vi "MC_7_26_12c_JW.vi"() -> ()   [LabVIEW 2011]
uses:
  <vilib>/Utility/file.llb/Read From Spreadsheet File (string).vi
  <vilib>/Utility/inputDevices.llb/keyboardAcquire.vi
  <vilib>/Utility/file.llb/Write To Spreadsheet File (DBL).vi
  <vilib>/Utility/file.llb/Write To Spreadsheet File (string).vi
  <vilib>/regexp/Match Regular Expression.xnode
panel:
  in  "Room Temp":dbl=294.0
  out "No Image 2":path=path "\\\\acad1\\physics/Jurchescu-group/JW-PD/Image Not Found.png"
  out "Save1 Array":string[][](array[string])
  out "XY Graph-Lin":cluster{dbl[], dbl[]}[](graph)
  out "Lin Vd":dbl
  out "Lin-Vg Array-Used":dbl[](array[numeric])
  out "Lin Id-Used":dbl[](array[numeric])
  out "Comments":string
  out "Folder Index":dbl caption="Length"
  out "Current \nRecord":string[](array[string])
  out "Transformer \nHeaders":string[](array[string])
  out "Current Device ID":string
  out "Column":string
  out "Row":string
  out "Rec: Concentration":dbl
  out "Rec: Solvent":string
  out "Rec: Method":string
  in  "?":T1(tab)
  out "Rec: Material":string
  in  "Treatment Concentration (mM):":dbl=30.0
  in  "Surface Treatment:":string
  in  "# Drops*:":dbl=inf
  in  "Solution Temp (C):":dbl=55.0
  in  "Relative Humidity (%):":dbl=nan
  in  "Room Temp (F):":dbl=nan
  in  "Time (s):":dbl=80.0
  out "Accel (RPM/s):":dbl
  in  "RPM:":dbl=1000.0
  in  "Wait Time (s):":dbl=10.0
  in  "Sample #:":dbl=1.0
  in  "Fabricator:":string="Jeremy"
  in  "Data File":path
  out "Data Folder":path
  in  "Image Folder":path
  out "Image File":path=path "D:/UserData/Desktop/Jeremy/WFU/Research/Programs/VI mods/Image Not Found.png"
  in  "Ramp (s):":dbl=3.0
  out "Calc: On/Off":dbl caption="On/Off-Sat" format="%#.2e"
  out "Calc: Off I-Sat":dbl caption="Off I-Sat" format="%#.2e"
  in  "Manuel-Dielectric":bool
  in  "Manuel-Length":bool
  out "Calc: VT-Lin":dbl
  out "New: VT-Lin":dbl
  out "Rec: VT-Lin":dbl caption="VT-Lin" format="%#_3g"
  out "Calc: Trap Density-STS":dbl format="%#.2e"
  out "New: Trap Density-STS":dbl format="%#.2e"
  out "Rec: Trap Density-STS":dbl caption="N-Sat (STS)" format="%#.2e"
  out "Calc: Trap Density-VT":dbl format="%#.2e"
  out "New: Trap Density-VT":dbl format="%#.2e"
  out "Rec: Trap Density-VT":dbl caption="N-Sat (VT)" format="%#.2e"
  out "Calc: Mobility-Lin":dbl format="%#.2e"
  out "New: Mobility-Lin":dbl format="%#_4e"
  out "Rec: Mobility-Lin":dbl caption="Mobility-Lin" format="%#_3e"
  out "Calc: Mobility-Sat":dbl format="%#.2e"
  out "Rec: Length":dbl caption="Length" format="%#_3g"
  out "Rec: Width":dbl caption="Width" format="%#_4g"
  out "Rec: Dielectric (d)":dbl caption="Dielectric (d)" format="%#_3g"
  out "XY Graph":cluster{dbl[], dbl[]}[](graph)
  in  "NumPts":dbl=5.0
  in  "Cancel Button":bool
  in  "Next Button":bool
  in  "Previous Button":bool
  in  "Up Button":bool
  in  "Down Button":bool
  out "Data Name:":string
  in  "Save Changes?":bool
  in  "New: Dielectric":dbl
  in  "New: Length":dbl
  in  "New: Width":dbl
  out "New: Mobility-Sat":dbl format="%#.2e"
  in  "Slide":dbl(slide) step=1.0 scale=-22.0..202.0 scale format="%#_1p"
  in  "Blank Button":bool
  in  "Zoom":i16(slide)=-3 scale=-5.0..5.0
  out "Image Out 2":T2(plugin-control)
  out "Image Out":T2(plugin-control)
  in  "Magnification":u16(ring) items=["5x", "10x", "20x", "50x", "80x"]
  out "Total Width":dbl
  out "Distances":dbl[](array[numeric])
  in  "Undo Button":bool
  in  "Remove Button":bool
  out "Rec: Mobility-Sat":dbl caption="Mobility-Sat" format="%#.2e"
  out "Index":string
  out "Image Name":string
  in  "Export":bool
  out "Calc: VT-Sat":dbl format="%#.2g"
  out "New: VT-Sat":dbl format="%#.2g"
  in  "Manual-Width":bool caption="Manual"
  out "XY Graph 2":cluster{dbl[], dbl[]}[](graph)
  in  "Next Button 2":bool
  in  "Previous Button 2":bool
  in  "Slide 2":dbl(slide) step=1.0 scale=-1.0..82.0 scale format="%#_1p"
  out "Calc: STS":dbl format="%#.2g"
  out "New: STS":dbl format="%#.2g"
  in  "NumPts 2":dbl=5.0 caption="NumPts"
  out "Rec: VT-Sat":dbl caption="VT-Sat" format="%#.2g"
  out "Rec: STS":dbl caption="STS-Sat" format="%#.2g"
  out "Rec: On/Off":dbl caption="On/Off-Sat" format="%#.2e"
  in  "Save Changes? 2":bool
  in  "Save Changes? 3":bool
  out "Date Recorded":string="Date Recorded" caption="Measured"
  out "Date Created":string caption="Fabricated"
  out "Rec: Temp":dbl caption="Sample Temp" format="%.1f"
  out "New: Temp":dbl format="%.1f"
  out "Rec: Off I-Sat":dbl caption="Off I-Sat" format="%#.2e"
  in  "Independant Variable":string(combo)="Length (um):"
  out "String":string
  in  "No Image":path=path "\\\\acad1\\physics/Jurchescu-group/JW-PD/Image Not Found.png"
  in  "Project":path=path "\\\\acad1\\physics/Jurchescu-group/JW-PD/Group Library/Origin Project Files/DeviceData_7_25a_JWW.opj"
  out "Index 2":dbl
  out "Sat Id-Log-Used":dbl[](array[numeric])
  out "Vg Array-Log-Used":dbl[](array[numeric])
  out "ROI Descriptor out":T3 {"Contours"."Type" items=["No Selection", "Point", "Line", "Rectangle", "Oval", "Polygon", "Freehand Region", "Annulus", "Unused2", "Unused3", "Broken Line", "Freehand Line", "Rotated Rectangle"]}
  out "ROI Descriptor":T3 {"Contours"."Type" items=["No Selection", "Point", "Line", "Rectangle", "Oval", "Polygon", "Freehand Region", "Annulus", "Unused2", "Unused3", "Broken Line", "Freehand Line", "Rotated Rectangle"]}
  out "Numeric 3":dbl
  out "Array 6":dbl[][](array[numeric])
  out "Cluster":T4
  out "Array 5":dbl[](array[numeric])
  out "Array 4":dbl[](array[numeric])
  out "Array 3":dbl[](array[numeric])
  out "Numeric 2":dbl
  out "Numeric":dbl
  out "Sat Id-Used":dbl[](array[numeric])
  out "Sat Vg Array-Used":dbl[](array[numeric])
  out "MobVi Index":dbl
  in  "Row Start":dbl=20.0
  # "Data Locations"
  # "Data Location"
  # "Image Location"
  # "Sample Properties"
  # "*     Inf = Full coverage\n   NaN = Unknown or Not Applicable"
  # "Recorded"
  # "Calculated"
  # "Re-Calculated"
  # "Manual"
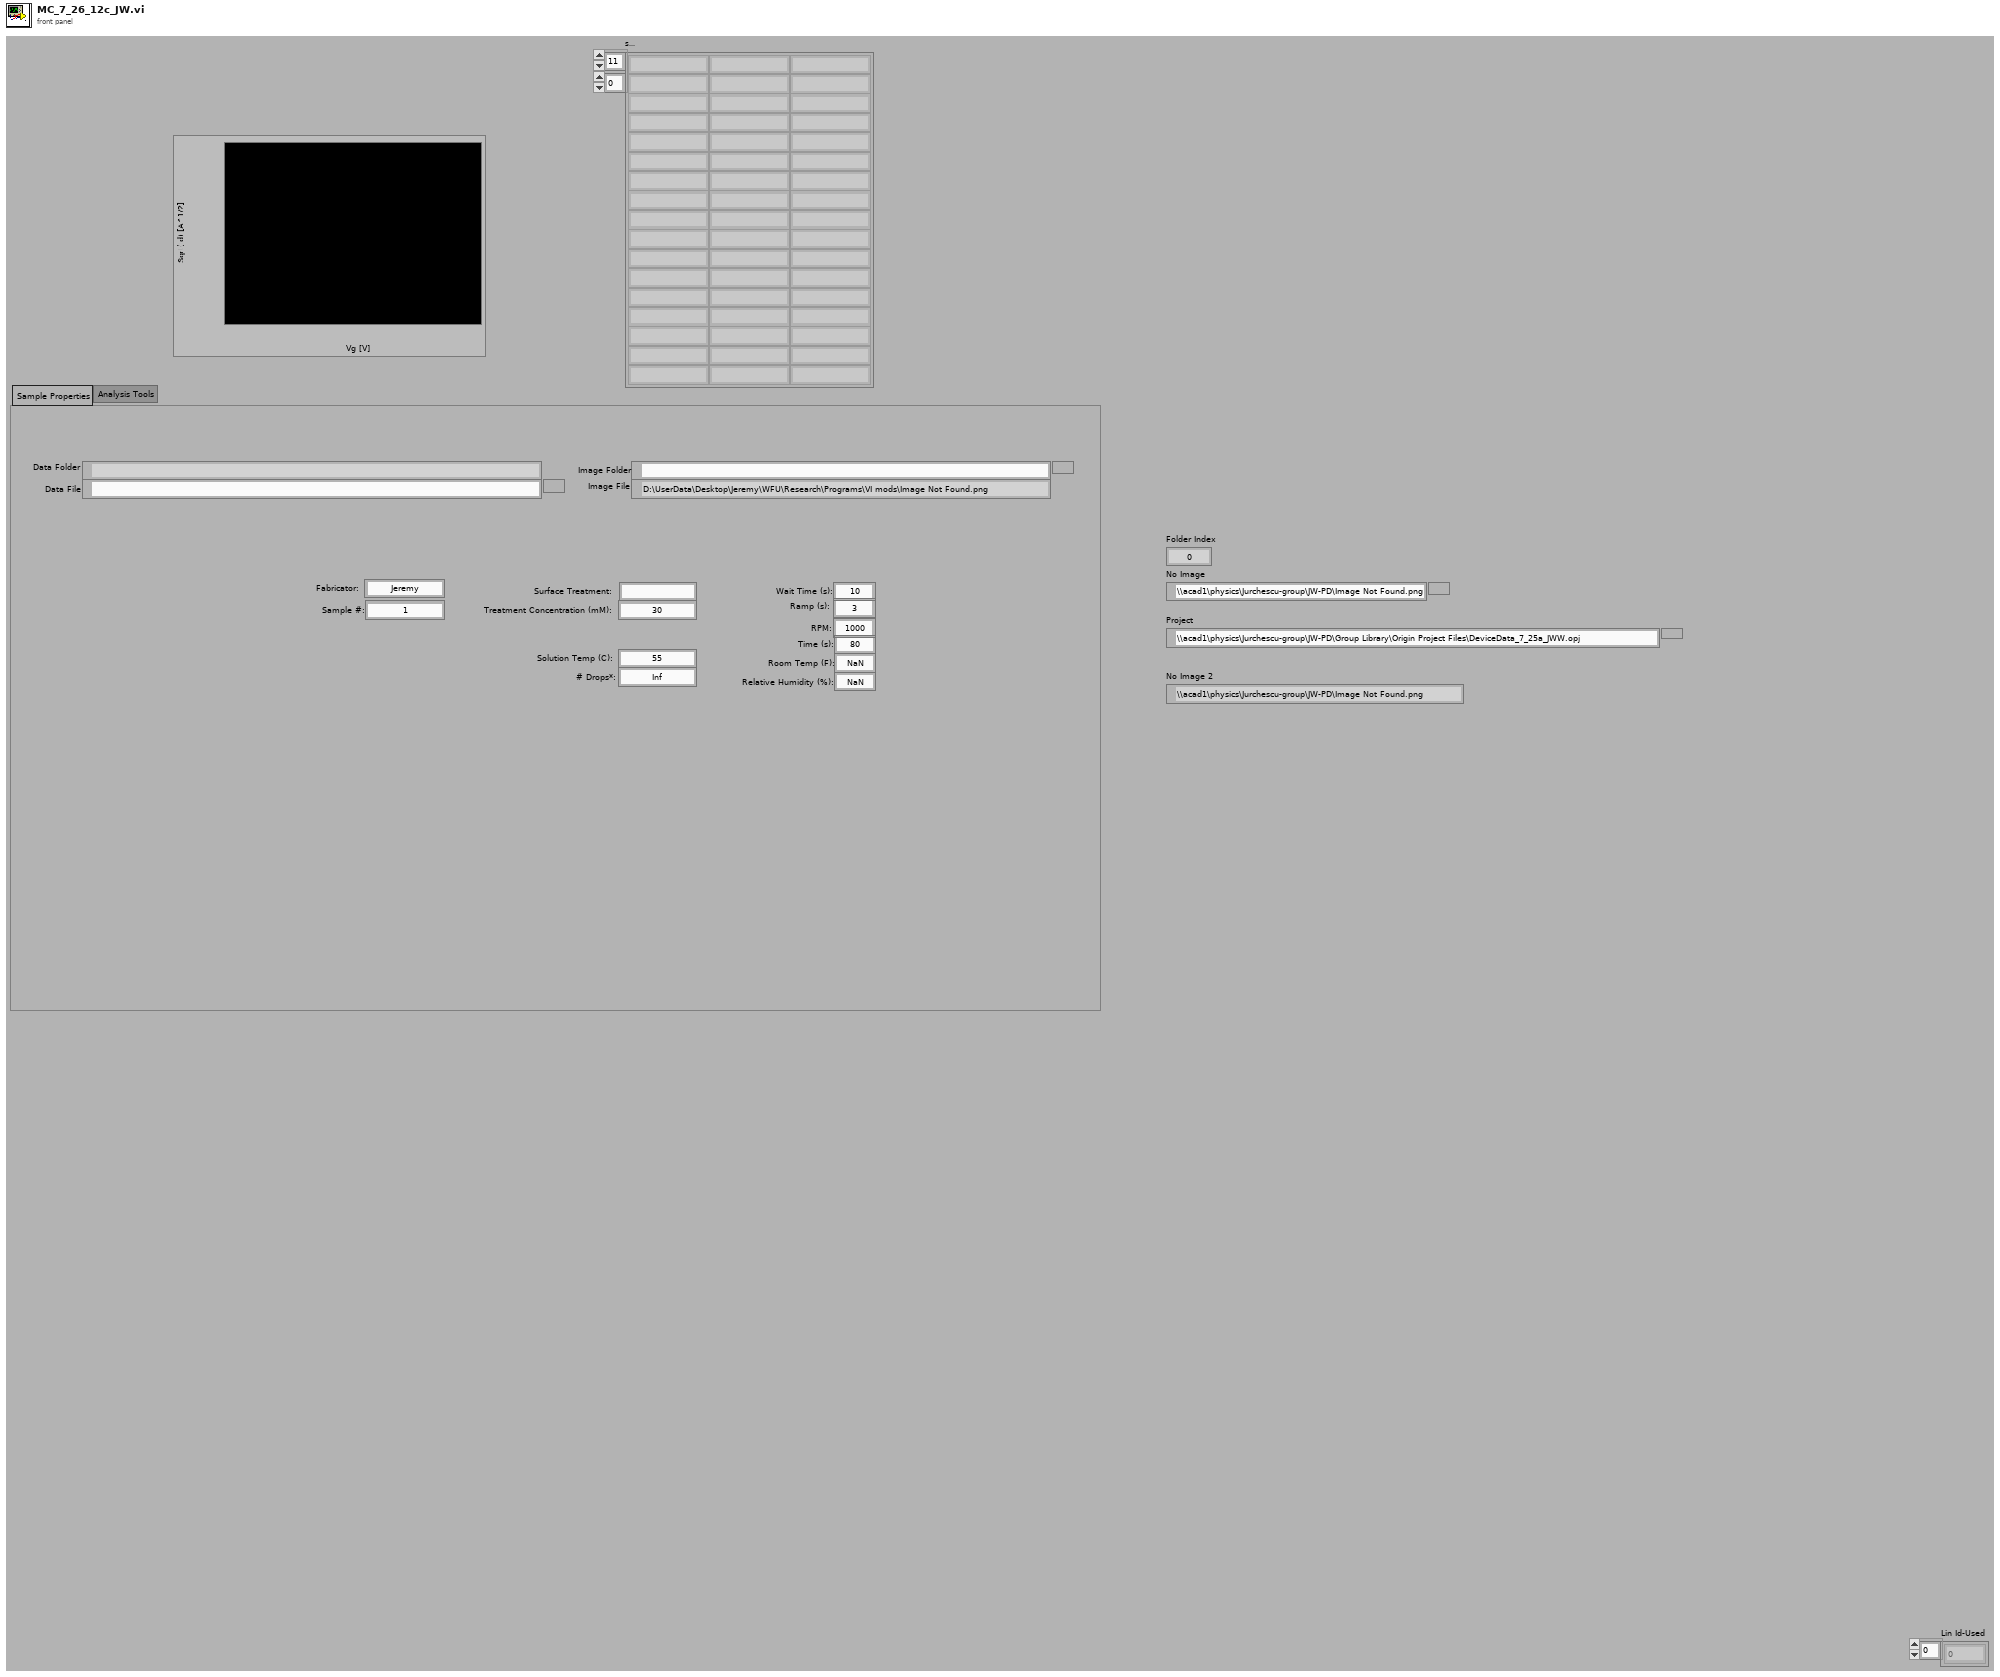
[diagram p1: front panel]
types:
  T1 = enum32{"Sample Properties", "Analysis Tools", "Current Database"}
  T2 = typedef "IMAQ Image.ctl" = refnum<image>
  T3 = typedef "ROI Descriptor" = cluster{"Global Rectangle":i32[], "Contours":cluster{"ID":enum32{"External", "Internal"}, "Type":u32, "Coordinates":i32[]}[]}
  T4 = cluster{"Numeric":dbl, "Numeric 2":dbl, "Numeric 3":dbl, "Numeric 4":dbl}
  T5 = cluster{"Mobility-Sat":dbl, "Moblitity-Lin":dbl, "On/Off":dbl, "Off Current":dbl, "Vt-Sat":dbl, "STS":dbl, "Trap Density-VT":dbl, "Trap Density-STS":dbl}
  T6 = cluster{"Date Recorded":string, "Index":string, "Length":dbl, "Width":dbl, "Sample Temp":dbl}
  T7 = cluster{"Date Created":string, "Material":string, "Solvent":string, "Concentration":dbl, "Method":string, "Dielectric (nm)":dbl, "Treatment":string, "Comments":string}
  T8 = cluster{"Mobility-Sat":dbl, "Vt-Sat":dbl, "Mobility-Lin":dbl, "Vt-Lin":dbl, "Off I-Sat":dbl, "On/Off I-Sat":dbl}
  T9 = cluster{"[0]":cluster{dbl[], dbl[]}, "[1]":cluster{dbl[], dbl[]}, "[2]":cluster{dbl[], dbl[]}, "[3]":cluster{dbl[], dbl[]}, "[4]":cluster{dbl[], dbl[]}, "[5]":cluster{dbl[], dbl[]}, "[6]":cluster{dbl[], dbl[]}, "[7]":cluster{dbl[], dbl[]}, "[8]":cluster{dbl[], dbl[]}}
  T10 = cluster{"Global Rectangle":i32[], "Contours":cluster{"Contour Type":u32, "ROI Type":u32, "Points":i32[]}[]}
  T11 = typedef "LVBoundsTypeDef.ctl" = cluster{"Width":u32, "Height":u32}
  T12 = enum16{"0", "1", "2", "3", "4", "5", "6", "7", "8", "9", "A", "B", "C", "D", "E", "F", "G", "H", "I", "J", "K", "L", "M", "N", "O", "P", "Q", "R", "S", "T", "U", "V", "W", "X", "Y", "Z", "F1", "F2", "F3", "F4", "F5", "F6", "F7", "F8", "F9", "F10", "F11", "F12", "F13", "F14", "F15", "ADD", "BACK", "BACKSLASH", "CAPITAL", "COMMA", "DECIMAL", "DELETE", "DIVIDE", "DOWN", "END", "EQUALS", "ESCAPE", "GRAVE (`)", "HOME", "INSERT", "LBRACKET", "LCONTROL", "LEFT", "L ALT", "LSHIFT", "LWIN", "MINUS", "MULTIPLY", "NEXT", "NUMLOCK", "NUMPAD_0", "NUMPAD_1", "NUMPAD_2", "NUMPAD_3", "NUMPAD_4", "NUMPAD_5", "NUMPAD_6", "NUMPAD_7", "NUMPAD_8", "NUMPAD_9", "PAUSE", "PERIOD", "PRIOR (PG UP)", "RBRACKET", "RCONTROL", "RETURN", "RIGHT", "R ALT", "RSHIFT", "RWIN", "SCROLL", "SEMICOLON", "SLASH", "SPACE", "SUBTRACT", "TAB", "UP", "ENTER (num pad)", "' (quote)"}[]
  T13 = enum16{"0", "1", "2", "3", "4", "5", "6", "7", "8", "9", "A", "B", "C", "D", "E", "F", "G", "H", "I", "J", "K", "L", "M", "N", "O", "P", "Q", "R", "S", "T", "U", "V", "W", "X", "Y", "Z", "F1", "F2", "F3", "F4", "F5", "F6", "F7", "F8", "F9", "F10", "F11", "F12", "F13", "F14", "F15", "ADD", "BACK", "BACKSLASH", "CAPITAL", "COMMA", "DECIMAL", "DELETE", "DIVIDE", "DOWN", "END", "EQUALS", "ESCAPE", "GRAVE (`)", "HOME", "INSERT", "LBRACKET", "LCONTROL", "LEFT", "L ALT", "LSHIFT", "LWIN", "MINUS", "MULTIPLY", "NEXT", "NUMLOCK", "NUMPAD_0", "NUMPAD_1", "NUMPAD_2", "NUMPAD_3", "NUMPAD_4", "NUMPAD_5", "NUMPAD_6", "NUMPAD_7", "NUMPAD_8", "NUMPAD_9", "PAUSE", "PERIOD", "PRIOR (PG UP)", "RBRACKET", "RCONTROL", "RETURN", "RIGHT", "R ALT", "RSHIFT", "RWIN", "SCROLL", "SEMICOLON", "SLASH", "SPACE", "SUBTRACT", "TAB", "UP", "ENTER (num pad)", "' (quote)"}
  T14 = cluster{"Contour Type":u32, "ROI Type":u32, "Points":i32[]}[]
  T15 = cluster{i32[], cluster{"Contour Type":u32, "ROI Type":u32, "Points":i32[]}[]}
  T16 = cluster{string, sgl, bool, bool, bool, bool, bool, bool, i32}
  T17 = cluster{i32, cluster{string, sgl, bool, bool, bool, bool, bool, bool, i32}, i32, i32}
  T18 = cluster{"Contour Type":u32, "ROI Type":u32, "Points":i32[]}
  T19 = cluster{"Points[0]":i32, "Points[1]":i32, "Points[2]":i32, "Points[3]":i32, "Points[4]":i32, "Points[5]":i32, "Points[6]":i32, "Points[7]":i32, "Points[8]":i32}
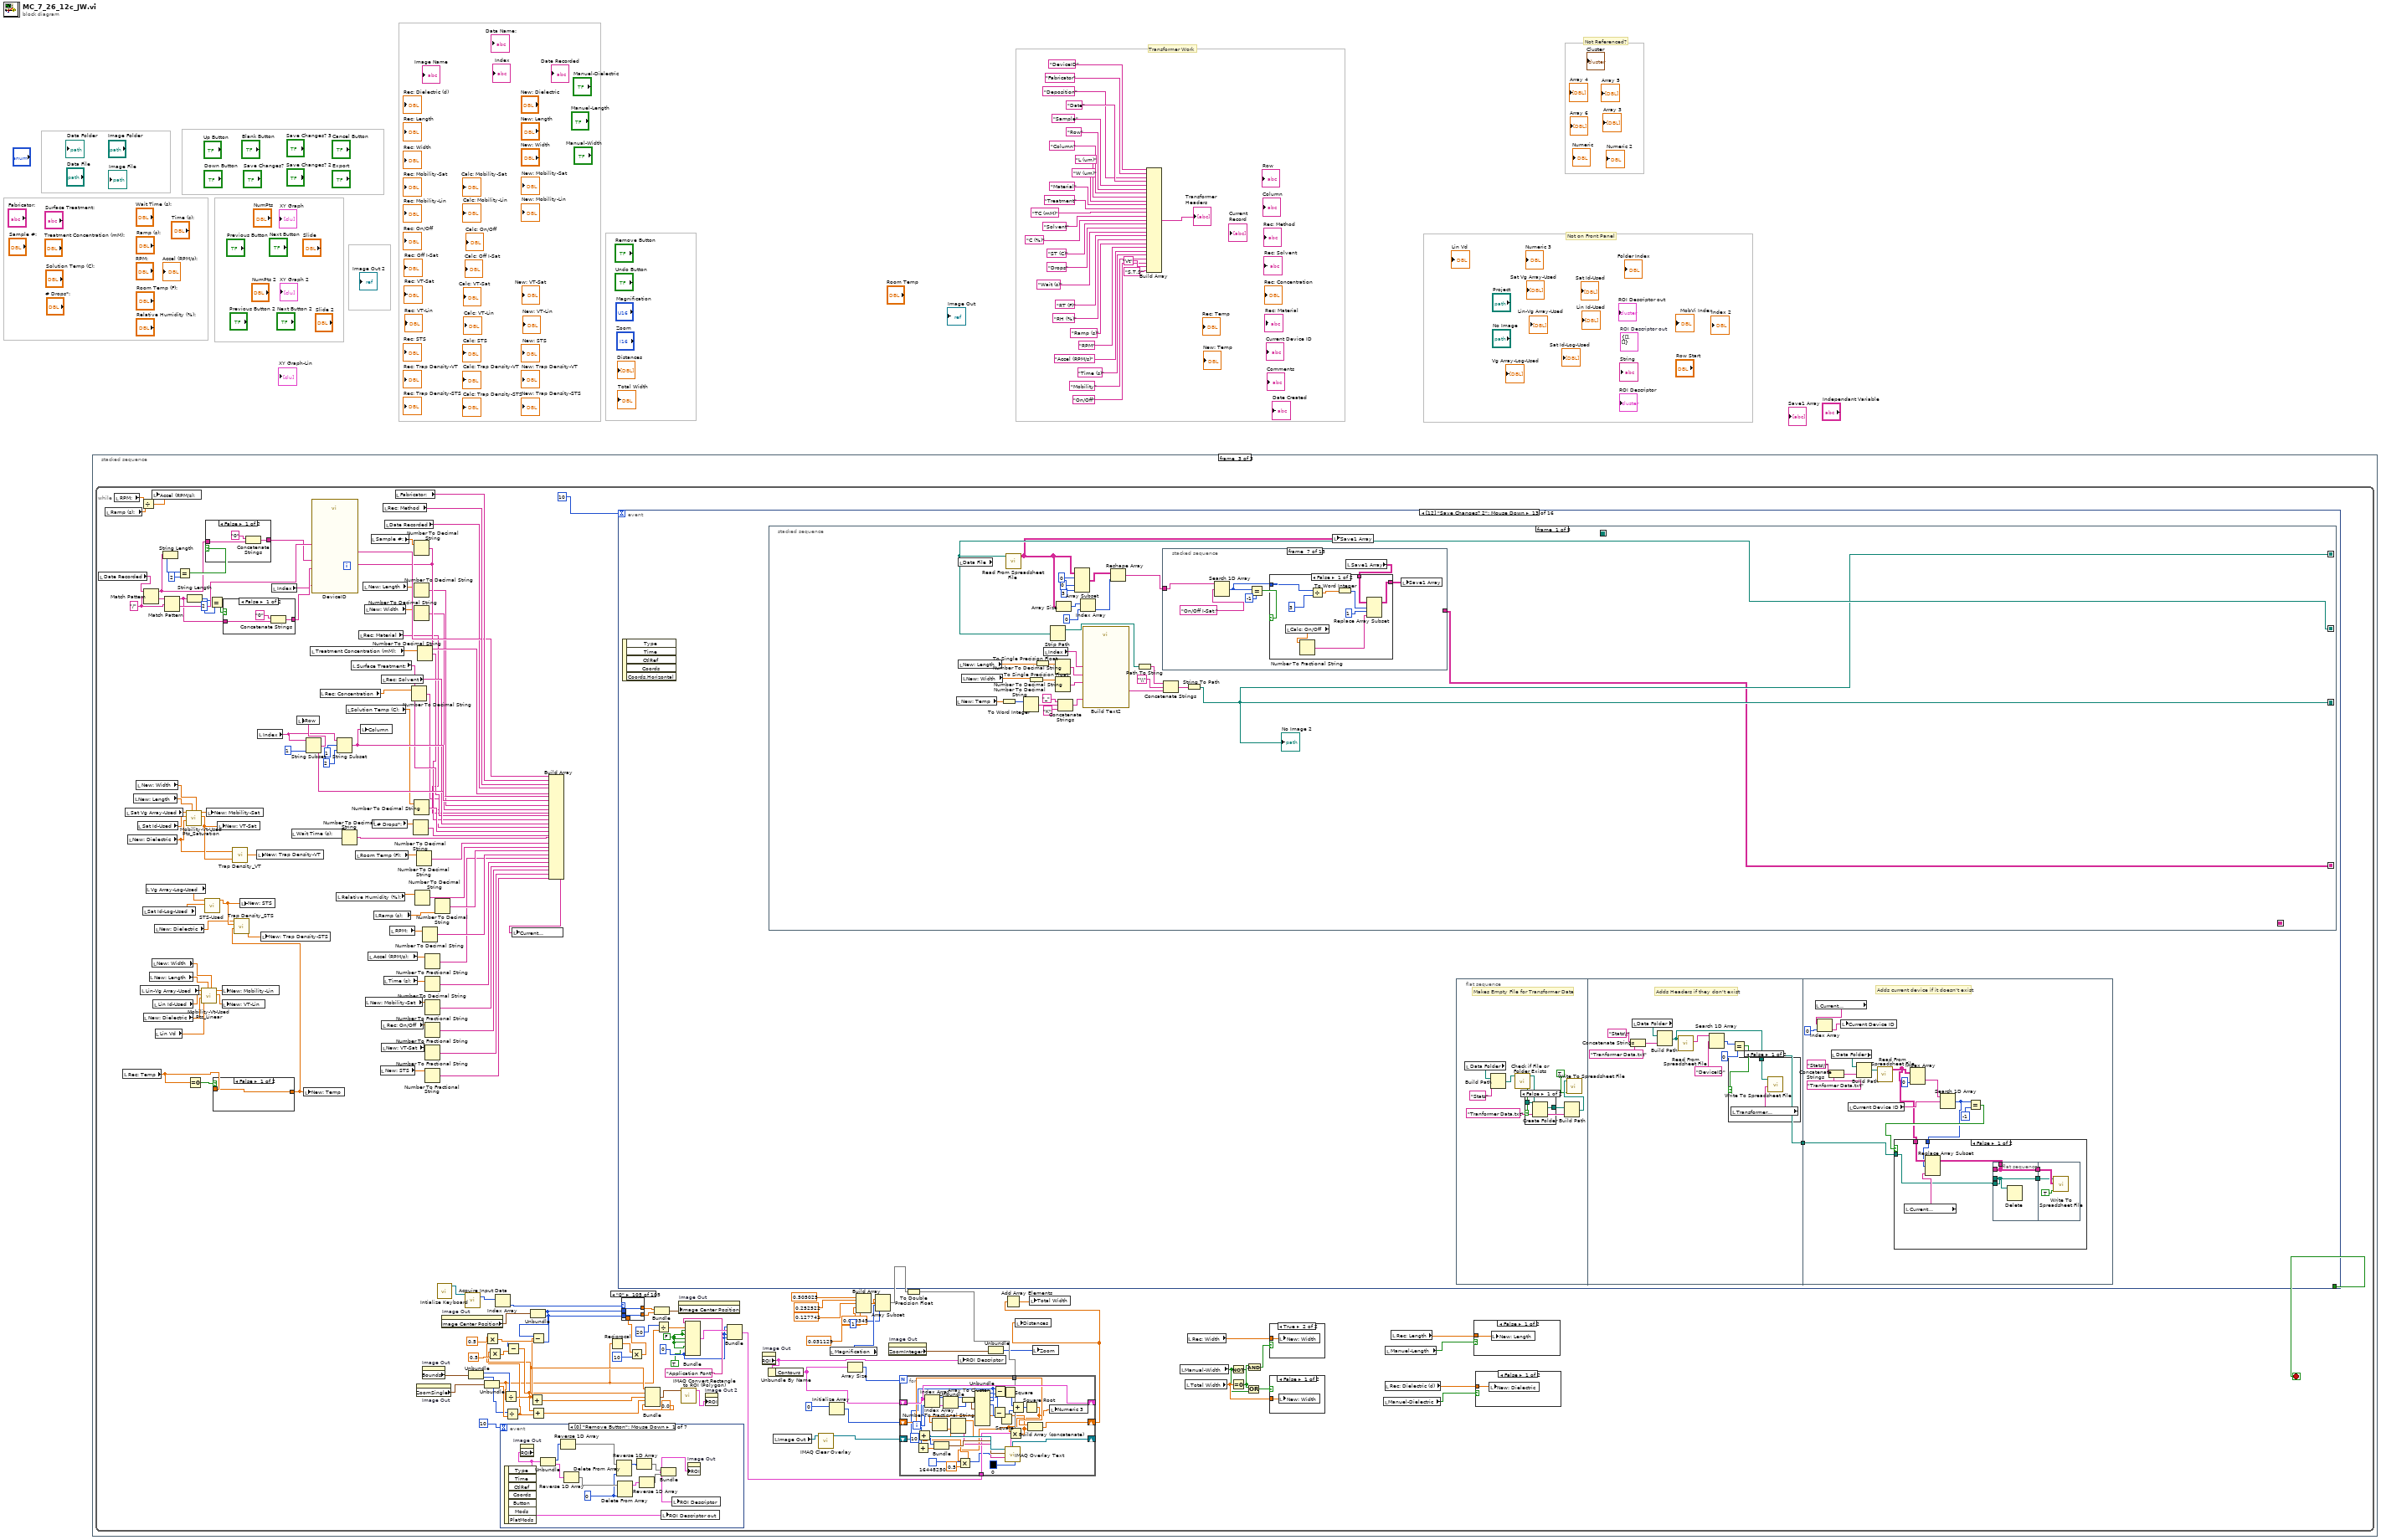
[diagram p0: block diagram]
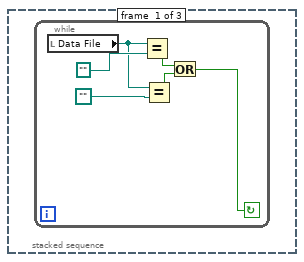
[diagram p2: hidden frame]
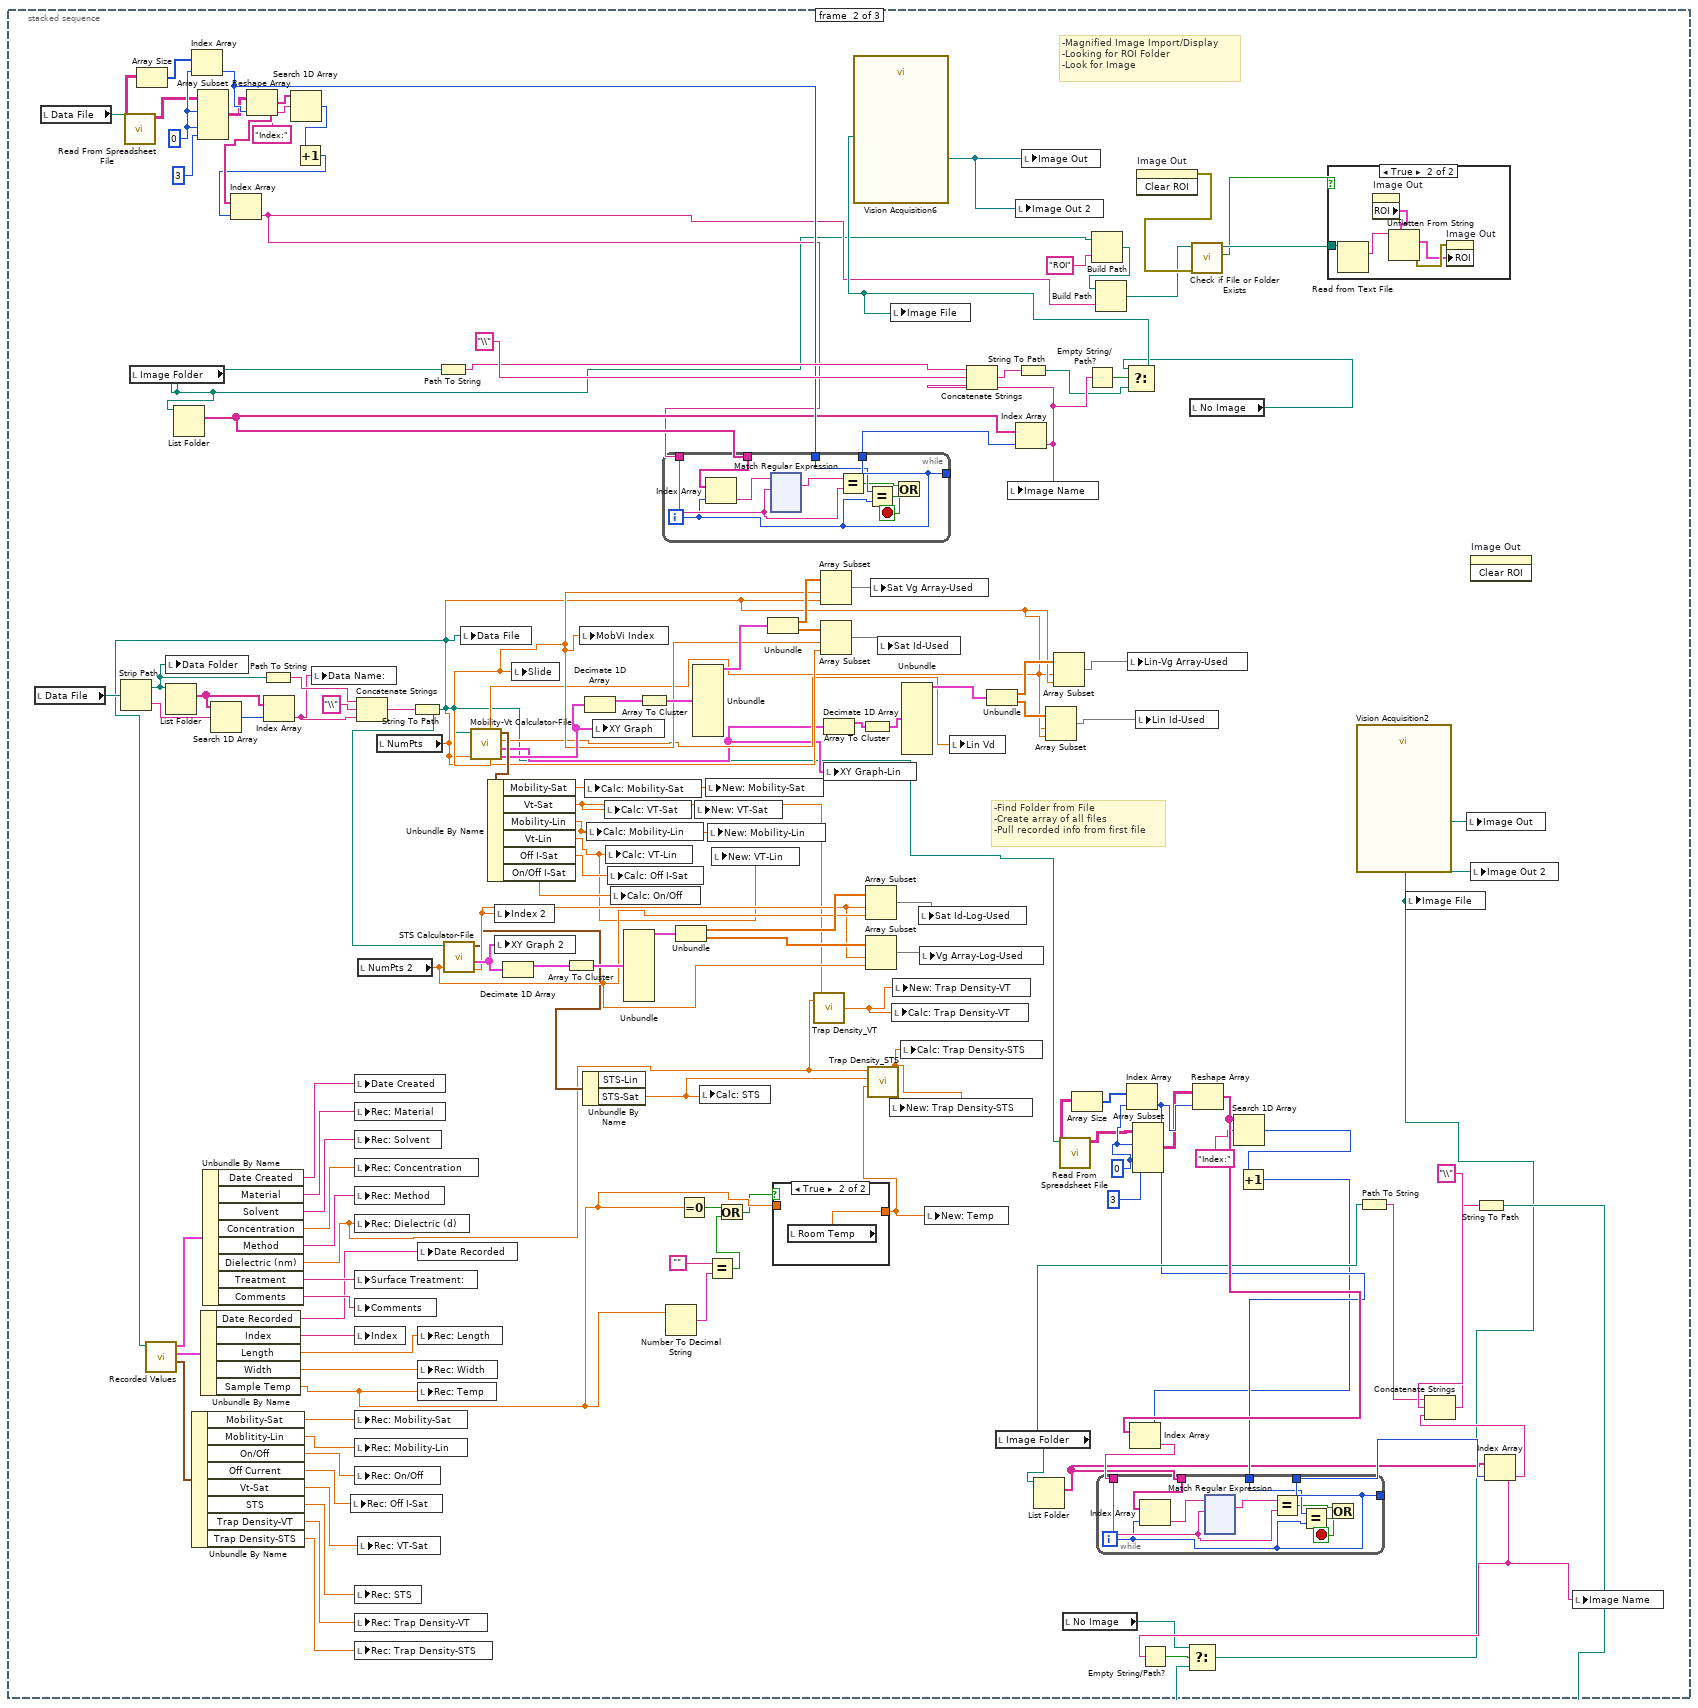
[diagram p3: hidden frame]
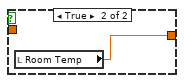
[diagram p6: hidden frame]
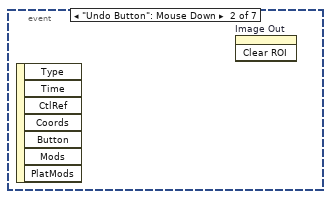
[diagram p13: hidden frame]
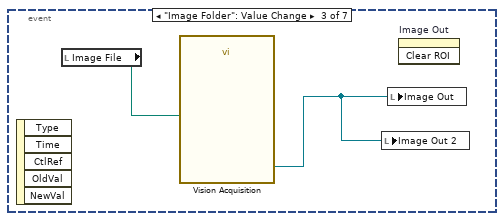
[diagram p14: hidden frame]
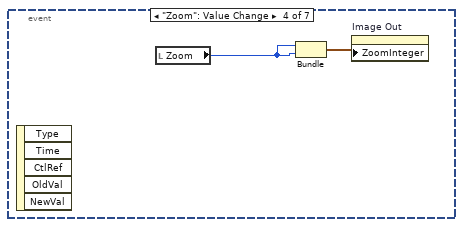
[diagram p15: hidden frame]
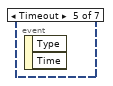
[diagram p16: hidden frame]
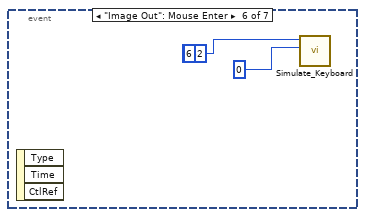
[diagram p17: hidden frame]
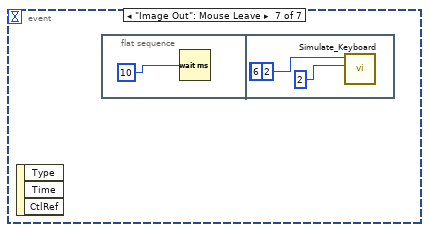
[diagram p18: hidden frame]
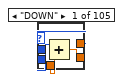
[diagram p19: hidden frame]
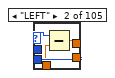
[diagram p20: hidden frame]
diagram:
  (unwired) T3 {"Global Rectangle"=[], "Contours"=[]}  # ROI Descriptor out
  # "Not Referenced?"
  # "Transformer Work"
  # "Not on Front Panel"
  n1 = stacked-sequence {
    frame #0 {
      n2 = while {
        stop <- w29 continue-if-true
        n3 = local read "Data File"() -> (w31:path)
        n4 = Equal?(x=w31, y=path "") -> (x = y?=w33:bool)
        n5 = Equal?(x=w31, y=path "") -> (x = y?=w32:bool)
        n6 = Or(x=w33, y=w32) -> (x .or. y?=w29:bool)
      }
    }
    frame #1 {
      w133 = 0
      w157 = 0
      # "-Find Folder from File\n-Create array of all files\n-Pull recorded info from first file"
      # "-Magnified Image Import/Display\n-Looking for ROI Folder\n-Look for Image"
      n7 = local read "Data File"() -> (w137:path)
      n8 = local read "Data File"() -> (w152:path)
      n9 = Strip Path(path=w137) -> (stripped path=w138:path, name=w124:string)
      n10 = call-poly <vilib>:"Read From Spreadsheet File.vi"("file path (dialog if empty)"=w152) -> ("all rows"=w155:string[][])  [unwired: 6 in, 4 out]
      n11 = local read "Image Folder"() -> (w94:path)
      n12 = Array Size(array=w155) -> (size(s)=w156:i32[])
      n13 = local write "Data Folder"(w138) -> ()
      n14 = List Folder(path=w138) -> (filenames=w128:string[])  [unwired: 3 in, 3 out]
      n15 = List Folder(path=w94) -> (filenames=w161:string[])  [unwired: 3 in, 3 out]
      n16 = Index Array(array=w156, index=w157) -> (element=w163:i32)
      n17 = Array Subset(array=w155, index (row)=w157, index (col)=w157, length (col)=3) -> (w154:string[][])  [unwired: 1 in]
      n18 = Search 1D Array(1D array=w128, element=w124) -> (index of element=w127:i32)  [unwired: 1 in]
      n19 = Reshape Array(w154, w163) -> (w168:string[])
      n20 = Path To String(path=w138) -> (string=w123:string)
      n21 = Index Array(array=w128, index=w127) -> (element=w93:string)
      n22 = Search 1D Array(1D array=w168, element="Index:") -> (index of element=w160:i32)  [unwired: 1 in]
      n23 = Increment(x=w160) -> (x+1=w159:i32)
      n24 = Index Array(array=w168, index=w159) -> (element=w95:string)
      n25 = local write "Data Name:"(w93) -> ()
      n26 = Concatenate Strings(w123, "\\", w93) -> (w125:string)
      n27 = local read "NumPts 2"() -> (w68:dbl)
      n28 = local read "NumPts"() -> (w59:dbl)
      n29 = String To Path(string=w125) -> (path=w52:path)
      n30 = call "Recorded Values.vi"("Path"=w52) -> ("Recorded Char"=w91:T5, "Recorded Prop"=w90:T6, "Fabrication Prop"=w92:T7)  [unwired: 8 in]
      n31 = Unbundle By Name(w91) -> ("Mobility-Sat"=w79:dbl, "Moblitity-Lin"=w78:dbl, "On/Off"=w77:dbl, "Off Current"=w76:dbl, "Vt-Sat"=w38:dbl, "STS"=w75:dbl, "Trap Density-VT"=w74:dbl, "Trap Density-STS"=w73:dbl)
      n32 = Unbundle By Name(w90) -> ("Date Recorded"=w83:string, "Index"=w82:string, "Length"=w81:dbl, "Width"=w80:dbl, "Sample Temp"=w44:dbl)
      n33 = Unbundle By Name(w92) -> ("Date Created"=w72:string, "Material"=w89:string, "Solvent"=w88:string, "Concentration"=w87:dbl, "Method"=w86:string, "Dielectric (nm)"=w48:dbl, "Treatment"=w85:string, "Comments"=w84:string)
      n34 = local write "Rec: Off I-Sat"(w76) -> ()
      n35 = local write "Date Created"(w72) -> ()
      n36 = local write "Rec: Material"(w89) -> ()
      n37 = local write "Rec: Solvent"(w88) -> ()
      n38 = local write "Rec: Concentration"(w87) -> ()
      n39 = local write "Rec: Method"(w86) -> ()
      n40 = local write "Rec: Dielectric (d)"(w48) -> ()
      n41 = local write "Surface Treatment:"(w85) -> ()
      n42 = local write "Comments"(w84) -> ()
      n43 = local write "Index"(w82) -> ()
      n44 = local write "Rec: Mobility-Sat"(w79) -> ()
      n45 = local write "Rec: Mobility-Lin"(w78) -> ()
      n46 = local write "Rec: On/Off"(w77) -> ()
      n47 = local write "Rec: STS"(w75) -> ()
      n48 = local write "Rec: Trap Density-VT"(w74) -> ()
      n49 = local write "Rec: Trap Density-STS"(w73) -> ()
      n50 = local write "Rec: VT-Sat"(w38) -> ()
      n51 = local write "Date Recorded"(w83) -> ()
      n52 = local write "Rec: Length"(w81) -> ()
      n53 = local write "Rec: Width"(w80) -> ()
      n54 = local write "Rec: Temp"(w44) -> ()
      n55 = Path To String(path=w94) -> (string=w165:string)
      n56 = call "STS Calculator-File.vi"("NumPts"=w68, "Path"=w52) -> ("STS Index-Sat"=w66:dbl, "XY Graph-Sat"=w67:cluster{dbl[], dbl[]}[], "Ouput"=w65:cluster{"STS-Sat":dbl, "STS-Lin":dbl})  [unwired: 5 in, 2 out]
      n57 = local write "Data File"(w52) -> ()
      n58 = call "Mobility-Vt Calculator-File.vi"("NumPts"=w59, "Path"=w52) -> ("XY Graph-Sat"=w70:cluster{dbl[], dbl[]}[], "XY Graph-Lin"=w54:cluster{dbl[], dbl[]}[], "Lin Vd"=w55:dbl, "Output"=w71:T8, "Index-Sat"=w69:dbl, "Index-Lin"=w58:dbl)  [unwired: 4 in]
      n59 = Unbundle By Name(w71) -> ("Mobility-Sat"=w47:dbl, "Vt-Sat"=w46:dbl, "Mobility-Lin"=w37:dbl, "Vt-Lin"=w35:dbl, "Off I-Sat"=w53:dbl, "On/Off I-Sat"=w36:dbl)
      n60 = local write "Index 2"(w66) -> ()
      n61 = local write "XY Graph 2"(w67) -> ()
      n62 = Decimate 1D Array(w67) -> (w115:cluster{dbl[], dbl[]}[])  [unwired: 1 out]
      n63 = local write "Slide"(w69) -> ()
      n64 = Array To Cluster(array=w115) -> (cluster=w117:T9)
      n65 = local write "MobVi Index"(w69) -> ()
      n66 = Unbundle By Name(w65) -> ("STS-Sat"=w51:dbl)  [unwired: 1 out]
      n67 = Decimate 1D Array(w70) -> (w151:cluster{dbl[], dbl[]}[])  [unwired: 1 out]
      n68 = local write "Calc: Mobility-Sat"(w47) -> ()
      n69 = local write "Calc: Mobility-Lin"(w37) -> ()
      n70 = local write "XY Graph"(w70) -> ()
      n71 = local write "Calc: VT-Sat"(w46) -> ()
      n72 = local write "Calc: VT-Lin"(w35) -> ()
      n73 = local write "Calc: Off I-Sat"(w53) -> ()
      n74 = local write "Calc: On/Off"(w36) -> ()
      n75 = Unbundle(w117) -> ("[0]"=w116:cluster{dbl[], dbl[]})  [unwired: 8 out]
      n76 = Array To Cluster(array=w151) -> (cluster=w149:T9)
      n77 = while {
        tunnel: w161 -> [w303]
        tunnel: w95 -> [w301]
        tunnel: [w300] -> _
        tunnel: [w300] -> w162
        tunnel: w163 -> [w299]
        i -> [w300]
        stop <- w296 stop-if-true
        n78 = Index Array(array=w303, index=w300) -> (element=w304:string)
        n79 = xnode "Match Regular Expression"("input string"=w304, "regular expression"=w301) -> ("whole match"=w302:string)  [unwired: 4 in, 4 out]
        n80 = Equal?(x=w302, y=w301) -> (x = y?=w298:bool)
        n81 = Equal?(x=w299, y=w300) -> (x = y?=w297:bool)
        n82 = Or(x=w298, y=w297) -> (x .or. y?=w296:bool)
      }
      n83 = Number To Decimal String(number=w44) -> (decimal integer string=w42:string)  [unwired: 1 in]
      n84 = Unbundle(w116) -> (w113:dbl[], w112:dbl[])
      n85 = Equal To 0?(x=w44) -> (x = 0?=w43:bool)
      n86 = Unbundle(w149) -> ("[0]"=w150:cluster{dbl[], dbl[]})  [unwired: 8 out]
      n87 = local write "New: VT-Sat"(w46) -> ()
      n88 = local write "Calc: STS"(w51) -> ()
      n89 = local write "New: Mobility-Sat"(w47) -> ()
      n90 = Equal?(x="", y=w42) -> (x = y?=w40:bool)
      n91 = local write "New: Mobility-Lin"(w37) -> ()
      n92 = local write "New: VT-Lin"(w35) -> ()
      n93 = Or(x=w43, y=w40) -> (x .or. y?=w39:bool)
      n94 = Unbundle(w150) -> (w114:dbl[], w118:dbl[])
      n95 = case shown="True" w39 {
        tunnel: [w169 w170] -> w50
        tunnel: w44 -> [w169 _]
        frame False {
        }
        frame True {
          n96 = local read "Room Temp"() -> (w170:dbl)
        }
      }
      n97 = call "Trap Density_VT.vi"("VT"=w46, "Dielectric"=w48) -> ("Trap Density-VT"=w45:dbl)
      n98 = Array Subset(array=w114, index=w69, length=w59) -> (w121:dbl[])
      n99 = Array Subset(array=w118, index=w69, length=w59) -> (w122:dbl[])
      n100 = Decimate 1D Array(w54) -> (w64:cluster{dbl[], dbl[]}[])  [unwired: 1 out]
      n101 = local write "XY Graph-Lin"(w54) -> ()
      n102 = Array To Cluster(array=w64) -> (cluster=w63:T9)
      n103 = Array Subset(array=w113, index=w66, length=w68) -> (w120:dbl[])
      n104 = Array Subset(array=w112, index=w66, length=w68) -> (w119:dbl[])
      n105 = call "Trap Density_STS.vi"("Temp (T) [K]"=w50, "S.T.S. (S)"=w51, "Dielectric"=w48) -> ("Trap Density (N)"=w49:dbl)  [unwired: 8 in]
      n106 = local write "Sat Vg Array-Used"(w121) -> ()
      n107 = local write "Sat Id-Used"(w122) -> ()
      n108 = local write "New: Trap Density-STS"(w49) -> ()
      n109 = local write "Calc: Trap Density-VT"(w45) -> ()
      n110 = local write "New: Trap Density-VT"(w45) -> ()
      n111 = local write "Calc: Trap Density-STS"(w49) -> ()
      n112 = Unbundle(w63) -> ("[0]"=w62:cluster{dbl[], dbl[]})  [unwired: 8 out]
      n113 = local write "Sat Id-Log-Used"(w120) -> ()
      n114 = local write "Vg Array-Log-Used"(w119) -> ()
      n115 = local write "New: Temp"(w50) -> ()
      n116 = local write "Lin Vd"(w55) -> ()
      n117 = Unbundle(w62) -> (w61:dbl[], w60:dbl[])
      n118 = local read "Image Folder"() -> (w144:path)
      n119 = Index Array(array=w161, index=w162) -> (element=w111:string)
      n120 = Concatenate Strings(w165, "\\", w111) -> (w166:string)
      n121 = local write "Image Name"(w111) -> ()
      n122 = String To Path(string=w166) -> (path=w109:path)
      n123 = List Folder(path=w144) -> (filenames=w140:string[])  [unwired: 3 in, 3 out]
      n124 = Array Subset(array=w60, index=w58, length=w59) -> (w56:dbl[])
      n125 = Array Subset(array=w61, index=w58, length=w59) -> (w57:dbl[])
      n126 = call-poly <vilib>:"Read From Spreadsheet File.vi"("file path (dialog if empty)"=w52) -> ("all rows"=w131:string[][])  [unwired: 6 in, 4 out]
      n127 = local read "No Image"() -> (w103:path)
      n128 = Array Size(array=w131) -> (size(s)=w132:i32[])
      n129 = Empty String/Path?(string/path=w111) -> (empty?=w110:bool)
      n130 = Build Path(base path=w94, name or relative path="ROI") -> (appended path=w97:path)
      n131 = Build Path(base path=w97, name or relative path=w95) -> (appended path=w96:path)
      n132 = Index Array(array=w132, index=w133) -> (element=w143:i32)
      n133 = local write "Lin-Vg Array-Used"(w57) -> ()
      n134 = Array Subset(array=w131, index (row)=w133, index (col)=w133, length (col)=3) -> (w130:string[][])  [unwired: 1 in]
      n135 = local write "Lin Id-Used"(w56) -> ()
      n136 = invoke on="Image Out" class="ImageControl" method="Clear ROI"() -> (error out=w101:errorcluster)  [unwired: 3 in, 2 out]
      n137 = local read "No Image"() -> (w102:path)
      n138 = Select(t=w102, s=w110, f=w109) -> (s? t:f=w108:path)
      n139 = call "Vision Acquisition6"("Image Path"=w108) -> ("Image Out"=w164:T2)  [unwired: 25 in, 1 out]
      n140 = local write "Image File"(w108) -> ()
      n141 = local write "Image Out 2"(w164) -> ()
      n142 = local write "Image Out"(w164) -> ()
      n143 = call <vilib>:"Check if File or Folder Exists.vi"("error in (no error)"=w101, "path"=w96) -> ("file or folder exists?"=w99:bool, "dup path"=w100:path)  [unwired: 7 in, 1 out]
      n144 = Reshape Array(w130, w143) -> (w148:string[])
      n145 = Search 1D Array(1D array=w148, element="Index:") -> (index of element=w136:i32)  [unwired: 1 in]
      n146 = Increment(x=w136) -> (x+1=w135:i32)
      n147 = Index Array(array=w148, index=w135) -> (element=w141:string)
      n148 = while {
        tunnel: w140 -> [w183]
        tunnel: w141 -> [w181]
        tunnel: [w180] -> _
        tunnel: [w180] -> w142
        tunnel: w143 -> [w179]
        i -> [w180]
        stop <- w176 stop-if-true
        n149 = Index Array(array=w183, index=w180) -> (element=w184:string)
        n150 = xnode "Match Regular Expression"("input string"=w184, "regular expression"=w181) -> ("whole match"=w182:string)  [unwired: 4 in, 4 out]
        n151 = Equal?(x=w182, y=w181) -> (x = y?=w178:bool)
        n152 = Equal?(x=w179, y=w180) -> (x = y?=w177:bool)
        n153 = Or(x=w178, y=w177) -> (x .or. y?=w176:bool)
      }
      n154 = case shown="True" w99 {
        tunnel: w100 -> [_ w171]
        frame False {
        }
        frame True {
          n155 = Read from Text File(file (use dialog)=w171) -> (text=w175:string)  [unwired: 3 in, 3 out]
          n156 = property on="Image Out" class="ImageControl"() -> ("ROI"=w172:T10)  [unwired: 2 in, 2 out]
          n157 = Unflatten From String(type=w172, binary string=w175) -> (value=w173:T10, error out=w174:errorcluster)  [unwired: 3 in, 1 out]
          n158 = property on="Image Out" class="ImageControl"(error in=w174, "ROI"=w173) -> ()  [unwired: 1 in, 2 out]
        }
      }
      n159 = Path To String(path=w144) -> (string=w145:string)
      n160 = invoke on="Image Out" class="ImageControl" method="Clear ROI"() -> ()  [unwired: 3 in, 3 out]
      n161 = Index Array(array=w140, index=w142) -> (element=w106:string)
      n162 = Empty String/Path?(string/path=w106) -> (empty?=w107:bool)
      n163 = Concatenate Strings(w145, "\\", w106) -> (w146:string)
      n164 = String To Path(string=w146) -> (path=w105:path)
      n165 = Select(t=w103, s=w107, f=w105) -> (s? t:f=w104:path)
      n166 = call "Vision Acquisition2"("Image Path"=w104) -> ("Image Out"=w139:T2)  [unwired: 25 in, 1 out]
      n167 = local write "Image File"(w104) -> ()
      n168 = local write "Image Out"(w139) -> ()
      n169 = local write "Image Out 2"(w139) -> ()
      n170 = local write "Image Name"(w106) -> ()
    }
    frame #2 {
      n171 = while {
        stop <- w581 stop-if-true
        w477 = "/"
        w531 = FALSE
        w529 = 0
        n172 = local read "Date Recorded"() -> (w480:string)
        n173 = local read "Ramp (s):"() -> (w447:dbl)
        n174 = local read "RPM:"() -> (w448:dbl)
        n175 = local read "Rec: Temp"() -> (w419:dbl)
        n176 = local read "Sat Vg Array-Used"() -> (w436:dbl[])
        n177 = local read "New: Dielectric"() -> (w421:dbl)
        n178 = local read "New: Length"() -> (w437:dbl)
        n179 = local read "New: Width"() -> (w439:dbl)
        n180 = local read "Sat Id-Used"() -> (w435:dbl[])
        n181 = local read "Lin-Vg Array-Used"() -> (w430:dbl[])
        n182 = Divide(x=w448, y=w447) -> (x/y=w446:dbl)
        n183 = local read "Sat Id-Log-Used"() -> (w434:dbl[])
        n184 = local read "New: Dielectric"() -> (w427:dbl)
        n185 = Match Pattern(string=w480, regular expression=w477) -> (before substring=w471:string, after substring=w478:string)  [unwired: 1 in, 2 out]
        n186 = local read "Vg Array-Log-Used"() -> (w433:dbl[])
        n187 = local read "New: Length"() -> (w429:dbl)
        n188 = local write "Accel (RPM/s):"(w446) -> ()
        n189 = local read "New: Width"() -> (w426:dbl)
        n190 = local read "Lin Id-Used"() -> (w431:dbl[])
        n191 = local read "New: Dielectric"() -> (w423:dbl)
        n192 = local read "Lin Vd"() -> (w425:dbl)
        n193 = String Length(string=w471) -> (length=w474:i32)
        n194 = Match Pattern(string=w478, regular expression=w477) -> (before substring=w465:string, after substring=w476:string)  [unwired: 1 in, 2 out]
        n195 = Equal?(x=w474, y=2) -> (x = y?=w472:bool)
        n196 = call "Mobility-Vt-Used Pts_Saturation.vi"("Width"=w439, "Length"=w437, "Dielectric (d)"=w421, "Sat Id Used"=w435, "Vg Used"=w436) -> ("Vt"=w422:dbl, "Mobility"=w438:dbl)  [unwired: 4 in, 1 out]
        n197 = String Length(string=w465) -> (length=w467:i32)
        n198 = Equal To 0?(x=w419) -> (x = 0?=w418:bool)
        n199 = call "Mobility-Vt-Used Pts_Linear.vi"("Width"=w426, "Length"=w429, "Vd"=w425, "Dielectric (d)"=w427, "Sat Id Used"=w431, "Vg Used"=w430) -> ("Vt"=w432:dbl, "Mobility"=w428:dbl)  [unwired: 3 in, 1 out]
        n200 = call "STS-Used.vi"("Id Used"=w434, "Vg-Used"=w433) -> ("STS"=w424:dbl)  [unwired: 9 in]
        n201 = case shown="False" w472 {
          tunnel: w471 -> [w591 w593]
          tunnel: [w590 w593] -> w470
          frame False {
            n202 = Concatenate Strings("0", w591) -> (w590:string)
          }
          frame True {
          }
        }
        n203 = local write "New: Mobility-Sat"(w438) -> ()
        n204 = Equal?(x=w467, y=2) -> (x = y?=w469:bool)
        n205 = case shown="False" w418 {
          tunnel: [w582 w583] -> w416
          tunnel: w419 -> [w582 _]
          frame False {
          }
          frame True {
            n206 = local read "Room Temp"() -> (w583:dbl)
          }
        }
        n207 = local write "New: VT-Sat"(w422) -> ()
        n208 = local write "New: Mobility-Lin"(w428) -> ()
        n209 = local write "New: VT-Lin"(w432) -> ()
        n210 = case shown="False" w469 {
          tunnel: w465 -> [w587 w589]
          tunnel: [w586 w589] -> w466
          frame False {
            n211 = Concatenate Strings("0", w587) -> (w586:string)
          }
          frame True {
          }
        }
        n212 = call "Trap Density_VT.vi"("VT"=w422, "Dielectric"=w421) -> ("Trap Density-VT"=w420:dbl)
        n213 = call "Trap Density_STS.vi"("Temp (T) [K]"=w416, "S.T.S. (S)"=w424, "Dielectric"=w423) -> ("Trap Density (N)"=w417:dbl)  [unwired: 8 in]
        n214 = local write "New: STS"(w424) -> ()
        n215 = local write "New: Trap Density-VT"(w420) -> ()
        n216 = local read "Index"() -> (w450:string)
        n217 = local write "New: Trap Density-STS"(w417) -> ()
        n218 = local read "Index"() -> (w464:string)
        n219 = local read "Wait Time (s):"() -> (w510:dbl)
        n220 = local write "New: Temp"(w416) -> ()
        n221 = String Subset(string=w450, length (rest)=1) -> (substring=w505:string)  [unwired: 1 in]
        n222 = local write "Row"(w505) -> ()
        n223 = local read "Treatment Concentration (mM):"() -> (w458:dbl)
        n224 = local read "Rec: Concentration"() -> (w445:dbl)
        n225 = local read "Relative Humidity (%):"() -> (w455:dbl)
        n226 = String Subset(string=w450, offset (0)=1, length (rest)=2) -> (substring=w506:string)
        n227 = Number To Decimal String(number=w510) -> (decimal integer string=w511:string)  [unwired: 1 in]
        n228 = local read "Solution Temp (C):"() -> (w499:dbl)
        n229 = local read "Surface Treatment:"() -> (w457:string)
        n230 = local read "Room Temp (F):"() -> (w503:dbl)
        n231 = local read "Rec: Material"() -> (w453:string)
        n232 = local write "Column"(w506) -> ()
        n233 = local read "New: Length"() -> (w463:dbl)
        n234 = local read "New: Width"() -> (w462:dbl)
        n235 = local read "New: Mobility-Sat"() -> (w492:dbl)
        n236 = local read "Accel (RPM/s):"() -> (w490:dbl)
        n237 = local read "Sample #:"() -> (w482:dbl)
        n238 = local read "# Drops*:"() -> (w500:dbl)
        n239 = local read "Ramp (s):"() -> (w508:dbl)
        n240 = local read "New: STS"() -> (w484:dbl)
        n241 = local read "Rec: Solvent"() -> (w459:string)
        n242 = local read "New: VT-Sat"() -> (w486:dbl)
        n243 = local read "Rec: On/Off"() -> (w488:dbl)
        n244 = local read "Rec: Method"() -> (w483:string)
        n245 = local read "Time (s):"() -> (w495:dbl)
        n246 = local read "Date Recorded"() -> (w479:string)
        n247 = local read "RPM:"() -> (w496:dbl)
        n248 = local read "Fabricator:"() -> (w504:string)
        n249 = Number To Decimal String(number=w445) -> (decimal integer string=w444:string)  [unwired: 1 in]
        n250 = Number To Decimal String(number=w500) -> (decimal integer string=w501:string)  [unwired: 1 in]
        n251 = Number To Decimal String(number=w482) -> (decimal integer string=w475:string)  [unwired: 1 in]
        n252 = call "DeviceID"("Sample"=w475, "Year"=w476, "Month"=w470, "Day"=w466, "Index"=w464) -> ("Result"=w481:string)  [unwired: 9 in, 1 out]
        n253 = Number To Decimal String(number=w463) -> (decimal integer string=w461:string)  [unwired: 1 in]
        n254 = Number To Decimal String(number=w462) -> (decimal integer string=w460:string)  [unwired: 1 in]
        n255 = Number To Decimal String(number=w499) -> (decimal integer string=w498:string)  [unwired: 1 in]
        n256 = Number To Decimal String(number=w455) -> (decimal integer string=w454:string)  [unwired: 1 in]
        n257 = Number To Decimal String(number=w503) -> (decimal integer string=w502:string)  [unwired: 1 in]
        n258 = property on="Image Out" class="ImageControl"() -> ("ZoomSingle"=w549:cluster{"X":sgl, "Y":sgl})  [unwired: 2 in, 2 out]
        n259 = Number To Decimal String(number=w458) -> (decimal integer string=w456:string)  [unwired: 1 in]
        n260 = property on="Image Out" class="ImageControl"() -> ("Bounds"=w550:T11)  [unwired: 2 in, 2 out]
        n261 = Number To Decimal String(number=w496) -> (decimal integer string=w497:string)  [unwired: 1 in]
        n262 = Number To Fractional String(number=w490) -> (F-format string=w491:string)  [unwired: 3 in]
        n263 = Number To Decimal String(number=w495) -> (decimal integer string=w494:string)  [unwired: 1 in]
        n264 = Number To Fractional String(number=w492) -> (F-format string=w493:string)  [unwired: 3 in]
        n265 = Number To Fractional String(number=w488) -> (F-format string=w489:string)  [unwired: 3 in]
        n266 = Number To Fractional String(number=w486) -> (F-format string=w487:string)  [unwired: 3 in]
        n267 = Number To Fractional String(number=w484) -> (F-format string=w485:string)  [unwired: 3 in]
        n268 = Number To Decimal String(number=w508) -> (decimal integer string=w509:string)  [unwired: 1 in]
        n269 = call <vilib>:"Intialize Keyboard.vi"() -> ("device ID"=w561:refnum<k1>)  [unwired: 10 in, 1 out]
        n270 = property on="Image Out" class="ImageControl"() -> ("Image Center Position"=w556:cluster{"X":u32, "Y":u32})  [unwired: 2 in, 2 out]
        n271 = call-poly <vilib>:"Acquire Input Data.vi"("device ID"=w561) -> ("keys pressed"=w560:T12)  [unwired: 16 in, 2 out]
        n272 = Unbundle(w550) -> ("Width"=w547:u32, "Height"=w546:u32)
        n273 = Unbundle(w549) -> ("X"=w524:sgl, "Y"=w548:sgl)
        n274 = Index Array(array=w560) -> (element=w564:T13)  [unwired: 1 in]
        n275 = event shown="[0] \"Remove Button\": Mouse Down" {
          selector: _ -> [_ _ _ _ _ _ _]
          dyn-events: _ -> [_ _ _ _ _ _ _]
          timeout: 10 -> [_ _ _ _ _ _ _]
          event "Remove Button": Mouse Down {
            w598 = 0
            n276 = event-data() -> ()  [unwired: 1 in, 7 out]
            n277 = property on="Image Out" class="ImageControl"() -> ("ROI"=w596:T10)  [unwired: 2 in, 2 out]
            n278 = Unbundle(w596) -> ("Global Rectangle"=w599:i32[], "Contours"=w601:T14)
            n279 = Reverse 1D Array(array=w599) -> (reversed array=w600:i32[])
            n280 = Reverse 1D Array(array=w601) -> (reversed array=w602:T14)
            n281 = Delete From Array(array=w600, index=w598) -> (array with subset deleted=w603:i32[])  [unwired: 1 in, 1 out]
            n282 = Delete From Array(array=w602, index=w598) -> (array with subset deleted=w604:T14)  [unwired: 1 in, 1 out]
            n283 = Reverse 1D Array(array=w603) -> (reversed array=w605:i32[])
            n284 = Reverse 1D Array(array=w604) -> (reversed array=w606:T14)
            n285 = Bundle(w605, w606) -> (w597:T15)  [unwired: 1 in]
            n286 = local write "ROI Descriptor out"(w596) -> ()
            n287 = local write "ROI Descriptor"(w597) -> ()
            n288 = property on="Image Out" class="ImageControl"("ROI"=w597) -> ()  [unwired: 2 in, 2 out]
          }
          event "Undo Button": Mouse Down {
            n289 = event-data() -> ()  [unwired: 1 in, 7 out]
            n290 = invoke on="Image Out" class="ImageControl" method="Clear ROI"() -> ()  [unwired: 3 in, 3 out]
          }
          event "Image Folder": Value Change {
            n291 = event-data() -> ()  [unwired: 1 in, 5 out]
            n292 = local read "Image File"() -> (w608:path)
            n293 = call "Vision Acquisition"("Image Path"=w608) -> ("Image Out"=w607:T2)  [unwired: 25 in, 1 out]
            n294 = local write "Image Out 2"(w607) -> ()
            n295 = local write "Image Out"(w607) -> ()
            n296 = invoke on="Image Out" class="ImageControl" method="Clear ROI"() -> ()  [unwired: 3 in, 3 out]
          }
          event "Zoom": Value Change {
            n297 = event-data() -> ()  [unwired: 1 in, 5 out]
            n298 = local read "Zoom"() -> (w609:i16)
            n299 = Bundle("Zoom"=w609, "Zoom"=w609) -> (w610:cluster{"Zoom":i16, "Zoom":i16})  [unwired: 1 in]
            n300 = property on="Image Out" class="ImageControl"("ZoomInteger"=w610) -> ()  [unwired: 2 in, 2 out]
          }
          event Timeout {
            n301 = event-data() -> ()  [unwired: 1 in, 2 out]
          }
          event "Image Out": Mouse Enter {
            (unwired) 6
            n302 = event-data() -> ()  [unwired: 1 in, 3 out]
            n303 = call "Simulate_Keyboard.vi"("Action"=0, "Virtual Key"=162) -> ()  [unwired: 7 in, 1 out]
          }
          event "Image Out": Mouse Leave {
            n304 = event-data() -> ()  [unwired: 1 in, 3 out]
            n305 = flat-sequence {
              frame #0 {
                n306 = Wait (ms)(milliseconds to wait=10) -> ()  [unwired: 1 out]
              }
              frame #1 {
                (unwired) 6
                n307 = call "Simulate_Keyboard.vi"("Action"=2, "Virtual Key"=162) -> ()  [unwired: 7 in, 1 out]
              }
            }
          }
        }
        n308 = Divide(x=w547, y=w524) -> (x/y=w537:sgl)
        n309 = Multiply(x=w537, y=0.5) -> (x*y=w543:dbl)
        n310 = Divide(x=w546, y=w548) -> (x/y=w536:sgl)
        n311 = Multiply(x=w536, y=0.5) -> (x*y=w542:dbl)
        n312 = Unbundle(w556) -> ("X"=w538:u32, "Y"=w539:u32)
        n313 = Subtract(x=w539, y=w542) -> (x-y=w540:dbl)
        n314 = Subtract(x=w538, y=w543) -> (x-y=w541:dbl)
        n315 = Add(x=w541, y=w537) -> (x+y=w555:dbl)
        n316 = Add(x=w540, y=w536) -> (x+y=w554:dbl)
        n317 = Build Array(w481, w504, w483, w479, w475, w505, w506, w461, w460, w453, w457, w456, w459, w444, w498, w501, w511, w502, w454, w509, w497, w491, w494, w493, w489, w487, w485) -> (w507:string[])
        n318 = local write "Current \nRecord"(w507) -> ()
        n319 = Reciprocal(x=w524) -> (1/x=w523:sgl)
        n320 = event shown="[12] \"Save Changes? 2\": Mouse Down" {
          selector: _ -> [_ _ _ _ _ _ _ _ _ _ _ _ _ _ _ _]
          dyn-events: _ -> [_ _ _ _ _ _ _ _ _ _ _ _ _ _ _ _]
          timeout: 10 -> [_ _ _ _ _ _ _ _ _ _ _ _ _ _ _ _]
          tunnel: [_ _ _ _ _ _ _ _ _ _ _ _ _ TRUE _ TRUE] -> w581
          event Timeout {
            n321 = event-data() -> ()  [unwired: 1 in, 2 out]
          }
          event "Down Button": Mouse Down {
            w950 = 0
            n322 = event-data() -> ()  [unwired: 1 in, 7 out]
            n323 = local read "Data File"() -> (w955:path)
            n324 = Strip Path(path=w955) -> (stripped path=w946:path, name=w964:string)
            n325 = local write "Data Folder"(w946) -> ()
            n326 = List Folder(path=w946) -> (filenames=w960:string[], error out=w900:errorcluster)  [unwired: 3 in, 2 out]
            n327 = local read "Folder Index"() -> (w902:dbl)
            n328 = property on="Image Out" class="ImageControl"() -> (error out=w903:errorcluster, "Image Center Position"=w907:cluster{"X":u32, "Y":u32})  [unwired: 2 in, 1 out]
            n329 = Array Size(array=w960) -> (size(s)=w956:i32)
            n330 = Search 1D Array(1D array=w960, element=w964) -> (index of element=w957:i32)  [unwired: 1 in]
            n331 = Decrement(x=w956) -> (x-1=w958:i32)
            n332 = Equal?(x=w957, y=w958) -> (x = y?=w959:bool)
            n333 = invoke on="Image Out" class="ImageControl" method="Clear ROI"() -> ()  [unwired: 3 in, 3 out]
            n334 = case shown="False" w959 {
              tunnel: w902 -> [w1117 _]
              tunnel: [w1116 0] -> w901
              tunnel: w900 -> [w1115 w1118]
              tunnel: [w1115 w1118] -> w899
              frame False {
                n335 = Increment(x=w1117) -> (x+1=w1116:dbl)
              }
              frame True {
              }
            }
            n336 = Unbundle(w907) -> ("X"=w905:u32)  [unwired: 1 out]
            n337 = local write "Folder Index"(w901) -> ()
            n338 = Bundle("X"=w905, 0) -> (w906:cluster{"X":u32, i32})  [unwired: 1 in]
            n339 = property on="Image Out" class="ImageControl"(error in=w903, "Image Center Position"=w906) -> ()  [unwired: 1 in, 2 out]
            n340 = Path To String(path=w946) -> (string=w965:string)
            n341 = Index Array(array=w960, index=w901) -> (element=w961:string)
            n342 = local write "Data Name:"(w961) -> ()
            n343 = Concatenate Strings(w965, "\\", w961) -> (w963:string)
            n344 = String To Path(string=w963) -> (path=w873:path)
            n345 = call "Recorded Values.vi"("Path"=w873) -> ("Recorded Char"=w967:T5, "Recorded Prop"=w968:T6, "Fabrication Prop"=w966:T7)  [unwired: 8 in]
            n346 = Unbundle By Name(w967) -> ("Mobility-Sat"=w980:dbl, "Moblitity-Lin"=w981:dbl, "On/Off"=w982:dbl, "Off Current"=w983:dbl, "Vt-Sat"=w868:dbl, "STS"=w984:dbl, "Trap Density-VT"=w985:dbl, "Trap Density-STS"=w986:dbl)
            n347 = Unbundle By Name(w966) -> ("Date Created"=w987:string, "Material"=w969:string, "Solvent"=w970:string, "Concentration"=w971:dbl, "Method"=w972:string, "Dielectric (nm)"=w973:dbl, "Treatment"=w974:string, "Comments"=w975:string)
            n348 = Unbundle By Name(w968) -> ("Date Recorded"=w976:string, "Index"=w977:string, "Length"=w978:dbl, "Width"=w979:dbl, "Sample Temp"=w870:dbl)
            n349 = local write "Date Created"(w987) -> ()
            n350 = local write "Rec: Off I-Sat"(w983) -> ()
            n351 = local write "Rec: Material"(w969) -> ()
            n352 = local write "Rec: VT-Sat"(w868) -> ()
            n353 = local write "Rec: Concentration"(w971) -> ()
            n354 = local write "Rec: Method"(w972) -> ()
            n355 = local write "Rec: Dielectric (d)"(w973) -> ()
            n356 = local write "Surface Treatment:"(w974) -> ()
            n357 = local write "Comments"(w975) -> ()
            n358 = local write "Index"(w977) -> ()
            n359 = local write "Rec: Mobility-Sat"(w980) -> ()
            n360 = local write "Rec: Mobility-Lin"(w981) -> ()
            n361 = local write "Rec: On/Off"(w982) -> ()
            n362 = local write "Rec: STS"(w984) -> ()
            n363 = local write "Rec: Trap Density-VT"(w985) -> ()
            n364 = local write "Rec: Trap Density-STS"(w986) -> ()
            n365 = local write "Rec: Solvent"(w970) -> ()
            n366 = local write "Date Recorded"(w976) -> ()
            n367 = local write "Rec: Length"(w978) -> ()
            n368 = local write "Rec: Width"(w979) -> ()
            n369 = local write "Rec: Temp"(w870) -> ()
            n370 = Equal To 0?(x=w870) -> (x = 0?=w871:bool)
            n371 = case shown="True" w871 {
              tunnel: [w988 w989] -> w869
              tunnel: w870 -> [w988 _]
              frame False {
              }
              frame True {
                n372 = local read "Room Temp"() -> (w989:dbl)
              }
            }
            n373 = local read "NumPts 2"() -> (w894:dbl)
            n374 = local read "NumPts"() -> (w898:dbl)
            n375 = local write "Data File"(w873) -> ()
            n376 = call-poly <vilib>:"Read From Spreadsheet File.vi"("file path (dialog if empty)"=w873) -> ("all rows"=w952:string[][])  [unwired: 6 in, 4 out]
            n377 = call "Mobility-Vt Calculator-File.vi"("NumPts"=w898, "Path"=w873) -> ("XY Graph-Sat"=w896:cluster{dbl[], dbl[]}[], "XY Graph-Lin"=w867:cluster{dbl[], dbl[]}[], "Output"=w897:T8, "Index-Sat"=w895:dbl, "Index-Lin"=w881:dbl)  [unwired: 4 in, 1 out]
            n378 = local read "New: Dielectric"() -> (w878:dbl)
            n379 = call "STS Calculator-File.vi"("NumPts"=w894, "Path"=w873) -> ("STS Index-Sat"=w893:dbl, "XY Graph-Sat"=w892:cluster{dbl[], dbl[]}[], "Ouput"=w891:cluster{"STS-Sat":dbl, "STS-Lin":dbl})  [unwired: 5 in, 2 out]
            n380 = Unbundle By Name(w897) -> ("Mobility-Sat"=w890:dbl, "Vt-Sat"=w877:dbl, "Mobility-Lin"=w889:dbl, "Vt-Lin"=w888:dbl, "Off I-Sat"=w874:dbl, "On/Off I-Sat"=w866:dbl)
            n381 = Unbundle By Name(w891) -> ("STS-Sat"=w872:dbl)  [unwired: 1 out]
            n382 = local write "Index 2"(w893) -> ()
            n383 = local write "XY Graph 2"(w892) -> ()
            n384 = local write "MobVi Index"(w895) -> ()
            n385 = local write "Slide"(w895) -> ()
            n386 = local write "XY Graph"(w896) -> ()
            n387 = Array Size(array=w952) -> (size(s)=w951:i32[])
            n388 = call "Trap Density_VT.vi"("VT"=w877, "Dielectric"=w878) -> ("Trap Density-VT"=w876:dbl)
            n389 = call "Trap Density_STS.vi"("Temp (T) [K]"=w869, "S.T.S. (S)"=w872, "Dielectric"=w878) -> ("Trap Density (N)"=w875:dbl)  [unwired: 8 in]
            n390 = local write "New: STS"(w872) -> ()
            n391 = local write "Calc: STS"(w872) -> ()
            n392 = local write "Calc: Mobility-Sat"(w890) -> ()
            n393 = local write "Calc: Off I-Sat"(w888) -> ()
            n394 = local write "Calc: Mobility-Lin"(w889) -> ()
            n395 = Index Array(array=w951, index=w950) -> (element=w932:i32)
            n396 = Decimate 1D Array(w892) -> (w926:cluster{dbl[], dbl[]}[])  [unwired: 1 out]
            n397 = Decimate 1D Array(w896) -> (w936:cluster{dbl[], dbl[]}[])  [unwired: 1 out]
            n398 = local write "Calc: Off I-Sat"(w874) -> ()
            n399 = local write "Calc: On/Off"(w866) -> ()
            n400 = Decimate 1D Array(w867) -> (w887:cluster{dbl[], dbl[]}[])  [unwired: 1 out]
            n401 = local write "Calc: VT-Sat"(w877) -> ()
            n402 = Array Subset(array=w952, index (row)=w950, index (col)=w950, length (col)=3) -> (w953:string[][])  [unwired: 1 in]
            n403 = local write "Calc: Trap Density-VT"(w876) -> ()
            n404 = local write "Calc: Trap Density-STS"(w875) -> ()
            n405 = local write "New: Trap Density-STS"(w875) -> ()
            n406 = local write "New: Trap Density-VT"(w876) -> ()
            n407 = local write "XY Graph-Lin"(w867) -> ()
            n408 = Array To Cluster(array=w926) -> (cluster=w924:T9)
            n409 = Array To Cluster(array=w936) -> (cluster=w938:T9)
            n410 = local write "New: VT-Lin"(w888) -> ()
            n411 = local write "New: VT-Sat"(w877) -> ()
            n412 = local write "New: Mobility-Sat"(w890) -> ()
            n413 = local write "New: Mobility-Lin"(w889) -> ()
            n414 = Reshape Array(w953, w932) -> (w939:string[])
            n415 = Array To Cluster(array=w887) -> (cluster=w886:T9)
            n416 = Subtract(x=w932, y=20) -> (x-y=w931:i32)
            n417 = property on="Slide" class="Slide (strict)"("Scale.Maximum"=w931) -> ()  [unwired: 2 in, 2 out]
            n418 = Unbundle(w924) -> ("[0]"=w925:cluster{dbl[], dbl[]})  [unwired: 8 out]
            n419 = Unbundle(w938) -> ("[0]"=w937:cluster{dbl[], dbl[]})  [unwired: 8 out]
            n420 = Unbundle(w886) -> ("[0]"=w883:cluster{dbl[], dbl[]})  [unwired: 8 out]
            n421 = Search 1D Array(1D array=w939, element="Index:") -> (index of element=w947:i32)  [unwired: 1 in]
            n422 = local read "NumPts"() -> (w882:dbl)
            n423 = Unbundle(w883) -> (w885:dbl[], w884:dbl[])
            n424 = Increment(x=w947) -> (x+1=w948:i32)
            n425 = Unbundle(w925) -> (w923:dbl[], w922:dbl[])
            n426 = Unbundle(w937) -> (w928:dbl[], w927:dbl[])
            n427 = Array Subset(array=w885, index=w881, length=w882) -> (w880:dbl[])
            n428 = Array Subset(array=w884, index=w881, length=w882) -> (w879:dbl[])
            n429 = Array Subset(array=w923, index=w893, length=w894) -> (w930:dbl[])
            n430 = Array Subset(array=w922, index=w893, length=w894) -> (w929:dbl[])
            n431 = Array Subset(array=w928, index=w895, length=w898) -> (w935:dbl[])
            n432 = Array Subset(array=w927, index=w895, length=w898) -> (w934:dbl[])
            n433 = Index Array(array=w939, index=w948) -> (element=w911:string)
            n434 = local write "Lin-Vg Array-Used"(w880) -> ()
            n435 = local write "Sat Vg Array-Used"(w935) -> ()
            n436 = local write "Vg Array-Log-Used"(w929) -> ()
            n437 = local write "Lin Id-Used"(w879) -> ()
            n438 = local read "Image Folder"() -> (w909:path)
            n439 = local write "Sat Id-Used"(w934) -> ()
            n440 = local write "Sat Id-Log-Used"(w930) -> ()
            n441 = List Folder(path=w909, error in=w899) -> (filenames=w945:string[], error out=w912:errorcluster)  [unwired: 2 in, 2 out]
            n442 = while {
              tunnel: w945 -> [w1002]
              tunnel: w911 -> [w1000]
              tunnel: [w999] -> _
              tunnel: [w999] -> w944
              tunnel: w932 -> [w998]
              i -> [w999]
              stop <- w995 stop-if-true
              n443 = Index Array(array=w1002, index=w999) -> (element=w1003:string)
              n444 = xnode "Match Regular Expression"("input string"=w1003, "regular expression"=w1000) -> ("whole match"=w1001:string)  [unwired: 4 in, 4 out]
              n445 = Equal?(x=w1001, y=w1000) -> (x = y?=w997:bool)
              n446 = Equal?(x=w998, y=w999) -> (x = y?=w996:bool)
              n447 = Or(x=w997, y=w996) -> (x .or. y?=w995:bool)
            }
            n448 = Build Path(base path=w909, name or relative path="ROI") -> (appended path=w908:path)
            n449 = Path To String(path=w909) -> (string=w942:string)
            n450 = Index Array(array=w945, index=w944) -> (element=w920:string)
            n451 = invoke on="Image Out" class="ImageControl" method="Clear ROI"(error in=w912) -> (error out=w915:errorcluster)  [unwired: 2 in, 2 out]
            n452 = local write "Image Name"(w920) -> ()
            n453 = Build Path(base path=w908, name or relative path=w911) -> (appended path=w916:path)
            n454 = call <vilib>:"Check if File or Folder Exists.vi"("error in (no error)"=w915, "path"=w916) -> ("file or folder exists?"=w913:bool, "dup path"=w914:path)  [unwired: 7 in, 1 out]
            n455 = Concatenate Strings(w942, "\\", w920) -> (w941:string)
            n456 = case shown="False" w913 {
              tunnel: w914 -> [_ w990]
              frame False {
              }
              frame True {
                n457 = Read from Text File(file (use dialog)=w990) -> (text=w994:string)  [unwired: 3 in, 3 out]
                n458 = property on="Image Out" class="ImageControl"() -> ("ROI"=w991:T10)  [unwired: 2 in, 2 out]
                n459 = Unflatten From String(type=w991, binary string=w994) -> (value=w992:T10, error out=w993:errorcluster)  [unwired: 3 in, 1 out]
                n460 = property on="Image Out" class="ImageControl"(error in=w993, "ROI"=w992) -> ()  [unwired: 1 in, 2 out]
              }
            }
            n461 = String To Path(string=w941) -> (path=w919:path)
            n462 = Empty String/Path?(string/path=w920) -> (empty?=w921:bool)
            n463 = local read "No Image"() -> (w917:path)
            n464 = Select(t=w917, s=w921, f=w919) -> (s? t:f=w918:path)
            n465 = local write "Image File"(w918) -> ()
            n466 = call "Vision Acquisition4"("Image Path"=w918) -> ("Image Out"=w943:T2)  [unwired: 25 in, 1 out]
            n467 = local write "Image Out"(w943) -> ()
            n468 = local write "Image Out 2"(w943) -> ()
          }
          event "Data File": Value Change {
            w1226 = 0
            n469 = event-data() -> ()  [unwired: 1 in, 5 out]
            n470 = local read "Data File"() -> (w1222:path)
            n471 = Strip Path(path=w1222) -> (stripped path=w1221:path, name=w1235:string)
            n472 = local write "Data Folder"(w1221) -> ()
            n473 = property on="Image Out" class="ImageControl"() -> (error out=w1177:errorcluster, "Image Center Position"=w1181:cluster{"X":u32, "Y":u32})  [unwired: 2 in, 1 out]
            n474 = List Folder(path=w1221) -> (filenames=w1231:string[], error out=w1187:errorcluster)  [unwired: 3 in, 2 out]
            n475 = Search 1D Array(1D array=w1231, element=w1235) -> (index of element=w1176:i32)  [unwired: 1 in]
            n476 = local write "Folder Index"(w1176) -> ()
            n477 = Unbundle(w1181) -> ("X"=w1179:u32)  [unwired: 1 out]
            n478 = Path To String(path=w1221) -> (string=w1236:string)
            n479 = Index Array(array=w1231, index=w1176) -> (element=w1232:string)
            n480 = Bundle("X"=w1179, 0) -> (w1180:cluster{"X":u32, i32})  [unwired: 1 in]
            n481 = local write "Data Name:"(w1232) -> ()
            n482 = property on="Image Out" class="ImageControl"(error in=w1177, "Image Center Position"=w1180) -> ()  [unwired: 1 in, 2 out]
            n483 = Concatenate Strings(w1236, "\\", w1232) -> (w1234:string)
            n484 = String To Path(string=w1234) -> (path=w1127:path)
            n485 = call "Recorded Values.vi"("Path"=w1127) -> ("Recorded Char"=w1174:T5, "Recorded Prop"=w1173:T6, "Fabrication Prop"=w1175:T7)  [unwired: 8 in]
            n486 = Unbundle By Name(w1174) -> ("Mobility-Sat"=w1161:dbl, "Moblitity-Lin"=w1160:dbl, "On/Off"=w1159:dbl, "Off Current"=w1158:dbl, "Vt-Sat"=w1123:dbl, "STS"=w1157:dbl, "Trap Density-VT"=w1156:dbl, "Trap Density-STS"=w1155:dbl)
            n487 = Unbundle By Name(w1175) -> ("Date Created"=w1154:string, "Material"=w1172:string, "Solvent"=w1171:string, "Concentration"=w1170:dbl, "Method"=w1169:string, "Dielectric (nm)"=w1168:dbl, "Treatment"=w1167:string, "Comments"=w1166:string)
            n488 = Unbundle By Name(w1173) -> ("Date Recorded"=w1165:string, "Index"=w1164:string, "Length"=w1163:dbl, "Width"=w1162:dbl, "Sample Temp"=w1125:dbl)
            n489 = local write "Date Created"(w1154) -> ()
            n490 = local write "Rec: Material"(w1172) -> ()
            n491 = local write "Rec: Off I-Sat"(w1158) -> ()
            n492 = local write "Rec: VT-Sat"(w1123) -> ()
            n493 = local write "Rec: Concentration"(w1170) -> ()
            n494 = local write "Rec: Method"(w1169) -> ()
            n495 = local write "Rec: Dielectric (d)"(w1168) -> ()
            n496 = local write "Surface Treatment:"(w1167) -> ()
            n497 = local write "Comments"(w1166) -> ()
            n498 = local write "Index"(w1164) -> ()
            n499 = local write "Rec: Mobility-Sat"(w1161) -> ()
            n500 = local write "Rec: Mobility-Lin"(w1160) -> ()
            n501 = local write "Rec: On/Off"(w1159) -> ()
            n502 = local write "Rec: STS"(w1157) -> ()
            n503 = local write "Rec: Trap Density-VT"(w1156) -> ()
            n504 = local write "Rec: Trap Density-STS"(w1155) -> ()
            n505 = local write "Rec: Solvent"(w1171) -> ()
            n506 = local write "Date Recorded"(w1165) -> ()
            n507 = local write "Rec: Length"(w1163) -> ()
            n508 = local write "Rec: Width"(w1162) -> ()
            n509 = local write "Rec: Temp"(w1125) -> ()
            n510 = Equal To 0?(x=w1125) -> (x = 0?=w1126:bool)
            n511 = case shown="False" w1126 {
              tunnel: [w1237 w1238] -> w1124
              tunnel: w1125 -> [w1237 _]
              frame False {
              }
              frame True {
                n512 = local read "Room Temp"() -> (w1238:dbl)
              }
            }
            n513 = local read "NumPts 2"() -> (w1149:dbl)
            n514 = local write "Data File"(w1127) -> ()
            n515 = local read "NumPts"() -> (w1150:dbl)
            n516 = call-poly <vilib>:"Read From Spreadsheet File.vi"("file path (dialog if empty)"=w1127) -> ("all rows"=w1228:string[][])  [unwired: 6 in, 4 out]
            n517 = local read "New: Dielectric"() -> (w1133:dbl)
            n518 = call "STS Calculator-File.vi"("NumPts"=w1149, "Path"=w1127) -> ("STS Index-Sat"=w1147:dbl, "XY Graph-Sat"=w1148:cluster{dbl[], dbl[]}[], "Ouput"=w1146:cluster{"STS-Sat":dbl, "STS-Lin":dbl})  [unwired: 5 in, 2 out]
            n519 = call "Mobility-Vt Calculator-File.vi"("NumPts"=w1150, "Path"=w1127) -> ("XY Graph-Sat"=w1153:cluster{dbl[], dbl[]}[], "XY Graph-Lin"=w1122:cluster{dbl[], dbl[]}[], "Output"=w1151:T8, "Index-Sat"=w1152:dbl, "Index-Lin"=w1139:dbl)  [unwired: 4 in, 1 out]
            n520 = Unbundle By Name(w1151) -> ("Mobility-Sat"=w1135:dbl, "Vt-Sat"=w1129:dbl, "Mobility-Lin"=w1134:dbl, "Vt-Lin"=w1120:dbl, "Off I-Sat"=w1128:dbl, "On/Off I-Sat"=w1121:dbl)
            n521 = local write "Index 2"(w1147) -> ()
            n522 = local write "XY Graph 2"(w1148) -> ()
            n523 = Unbundle By Name(w1146) -> ("STS-Sat"=w1130:dbl)  [unwired: 1 out]
            n524 = local write "MobVi Index"(w1152) -> ()
            n525 = Array Size(array=w1228) -> (size(s)=w1227:i32[])
            n526 = call "Trap Density_VT.vi"("VT"=w1129, "Dielectric"=w1133) -> ("Trap Density-VT"=w1132:dbl)
            n527 = call "Trap Density_STS.vi"("Temp (T) [K]"=w1124, "S.T.S. (S)"=w1130, "Dielectric"=w1133) -> ("Trap Density (N)"=w1131:dbl)  [unwired: 8 in]
            n528 = local write "Slide"(w1152) -> ()
            n529 = local write "Calc: Mobility-Lin"(w1134) -> ()
            n530 = local write "Calc: Mobility-Sat"(w1135) -> ()
            n531 = local write "Calc: VT-Sat"(w1129) -> ()
            n532 = local write "Calc: Off I-Sat"(w1128) -> ()
            n533 = local write "Calc: VT-Lin"(w1120) -> ()
            n534 = local write "Calc: On/Off"(w1121) -> ()
            n535 = local write "Calc: STS"(w1130) -> ()
            n536 = Decimate 1D Array(w1122) -> (w1145:cluster{dbl[], dbl[]}[])  [unwired: 1 out]
            n537 = local write "Calc: Trap Density-VT"(w1132) -> ()
            n538 = local write "Calc: Trap Density-STS"(w1131) -> ()
            n539 = local write "New: Trap Density-STS"(w1131) -> ()
            n540 = local write "New: Trap Density-VT"(w1132) -> ()
            n541 = local write "XY Graph-Lin"(w1122) -> ()
            n542 = local write "New: VT-Sat"(w1129) -> ()
            n543 = Decimate 1D Array(w1148) -> (w1202:cluster{dbl[], dbl[]}[])  [unwired: 1 out]
            n544 = Index Array(array=w1227, index=w1226) -> (element=w1208:i32)
            n545 = Decimate 1D Array(w1153) -> (w1211:cluster{dbl[], dbl[]}[])  [unwired: 1 out]
            n546 = local write "XY Graph"(w1153) -> ()
            n547 = local write "New: Mobility-Lin"(w1134) -> ()
            n548 = Array Subset(array=w1228, index (row)=w1226, index (col)=w1226, length (col)=3) -> (w1229:string[][])  [unwired: 1 in]
            n549 = local write "New: VT-Lin"(w1120) -> ()
            n550 = Array To Cluster(array=w1145) -> (cluster=w1144:T9)
            n551 = local write "New: STS"(w1130) -> ()
            n552 = local write "New: Mobility-Sat"(w1135) -> ()
            n553 = Array To Cluster(array=w1202) -> (cluster=w1200:T9)
            n554 = Array To Cluster(array=w1211) -> (cluster=w1213:T9)
            n555 = Reshape Array(w1229, w1208) -> (w1214:string[])
            n556 = Subtract(x=w1208, y=20) -> (x-y=w1206:i32)
            n557 = Unbundle(w1144) -> ("[0]"=w1143:cluster{dbl[], dbl[]})  [unwired: 8 out]
            n558 = property on="Slide" class="Slide (strict)"("Scale.Maximum"=w1206) -> ()  [unwired: 2 in, 2 out]
            n559 = local read "NumPts"() -> (w1140:dbl)
            n560 = Unbundle(w1143) -> (w1142:dbl[], w1141:dbl[])
            n561 = Unbundle(w1200) -> ("[0]"=w1201:cluster{dbl[], dbl[]})  [unwired: 8 out]
            n562 = Unbundle(w1213) -> ("[0]"=w1212:cluster{dbl[], dbl[]})  [unwired: 8 out]
            n563 = Search 1D Array(1D array=w1214, element="Index:") -> (index of element=w1223:i32)  [unwired: 1 in]
            n564 = local read "NumPts"() -> (w1136:dbl)
            n565 = Array Subset(array=w1142, index=w1139, length=w1140) -> (w1138:dbl[])
            n566 = Array Subset(array=w1141, index=w1139, length=w1140) -> (w1137:dbl[])
            n567 = Increment(x=w1223) -> (x+1=w1224:i32)
            n568 = Unbundle(w1201) -> (w1198:dbl[], w1197:dbl[])
            n569 = Unbundle(w1212) -> (w1199:dbl[], w1203:dbl[])
            n570 = local read "Image Folder"() -> (w1183:path)
            n571 = local write "Lin-Vg Array-Used"(w1138) -> ()
            n572 = Array Subset(array=w1198, index=w1147, length=w1149) -> (w1205:dbl[])
            n573 = Array Subset(array=w1197, index=w1147, length=w1149) -> (w1204:dbl[])
            n574 = Array Subset(array=w1199, index=w1152, length=w1136) -> (w1210:dbl[])
            n575 = Array Subset(array=w1203, index=w1152, length=w1136) -> (w1209:dbl[])
            n576 = Index Array(array=w1214, index=w1224) -> (element=w1185:string)
            n577 = local write "Lin Id-Used"(w1137) -> ()
            n578 = local write "Sat Vg Array-Used"(w1210) -> ()
            n579 = local write "Vg Array-Log-Used"(w1204) -> ()
            n580 = local write "Sat Id-Log-Used"(w1205) -> ()
            n581 = local write "Sat Id-Used"(w1209) -> ()
            n582 = local write "Index"(w1185) -> ()
            n583 = List Folder(path=w1183, error in=w1187) -> (filenames=w1219:string[], error out=w1186:errorcluster)  [unwired: 2 in, 2 out]
            n584 = Build Path(base path=w1183, name or relative path="ROI") -> (appended path=w1182:path)
            n585 = while {
              tunnel: w1219 -> [w1251]
              tunnel: w1185 -> [w1249]
              tunnel: [w1248] -> _
              tunnel: [w1248] -> w1218
              tunnel: w1208 -> [w1247]
              i -> [w1248]
              stop <- w1244 stop-if-true
              n586 = Index Array(array=w1251, index=w1248) -> (element=w1252:string)
              n587 = xnode "Match Regular Expression"("input string"=w1252, "regular expression"=w1249) -> ("whole match"=w1250:string)  [unwired: 4 in, 4 out]
              n588 = Equal?(x=w1250, y=w1249) -> (x = y?=w1246:bool)
              n589 = Equal?(x=w1247, y=w1248) -> (x = y?=w1245:bool)
              n590 = Or(x=w1246, y=w1245) -> (x .or. y?=w1244:bool)
            }
            n591 = invoke on="Image Out" class="ImageControl" method="Clear ROI"(error in=w1186) -> (error out=w1190:errorcluster)  [unwired: 2 in, 2 out]
            n592 = Build Path(base path=w1182, name or relative path=w1185) -> (appended path=w1191:path)
            n593 = call <vilib>:"Check if File or Folder Exists.vi"("error in (no error)"=w1190, "path"=w1191) -> ("file or folder exists?"=w1188:bool, "dup path"=w1189:path)  [unwired: 7 in, 1 out]
            n594 = case shown="True" w1188 {
              tunnel: w1189 -> [_ w1239]
              frame False {
              }
              frame True {
                n595 = Read from Text File(file (use dialog)=w1239) -> (text=w1243:string)  [unwired: 3 in, 3 out]
                n596 = property on="Image Out" class="ImageControl"() -> ("ROI"=w1240:T10)  [unwired: 2 in, 2 out]
                n597 = Unflatten From String(type=w1240, binary string=w1243) -> (value=w1241:T10, error out=w1242:errorcluster)  [unwired: 3 in, 1 out]
                n598 = property on="Image Out" class="ImageControl"(error in=w1242, "ROI"=w1241) -> ()  [unwired: 1 in, 2 out]
              }
            }
            n599 = invoke on="Image Out" class="ImageControl" method="Clear ROI"() -> ()  [unwired: 3 in, 3 out]
            n600 = Path To String(path=w1183) -> (string=w1217:string)
            n601 = Index Array(array=w1219, index=w1218) -> (element=w1195:string)
            n602 = Concatenate Strings(w1217, "\\", w1195) -> (w1216:string)
            n603 = local write "Image Name"(w1195) -> ()
            n604 = String To Path(string=w1216) -> (path=w1194:path)
            n605 = Empty String/Path?(string/path=w1195) -> (empty?=w1196:bool)
            n606 = local read "No Image"() -> (w1192:path)
            n607 = Select(t=w1192, s=w1196, f=w1194) -> (s? t:f=w1193:path)
            n608 = local write "Image File"(w1193) -> ()
            n609 = call "Vision Acquisition3"("Image Path"=w1193) -> ("Image Out"=w1220:T2)  [unwired: 25 in, 1 out]
            n610 = local write "Image Out"(w1220) -> ()
            n611 = local write "Image Out 2"(w1220) -> ()
          }
          event "Up Button": Mouse Down {
            w1471 = 0
            n612 = event-data() -> ()  [unwired: 1 in, 5 out]
            n613 = local read "Data File"() -> (w1467:path)
            n614 = Strip Path(path=w1467) -> (stripped path=w1466:path, name=w1482:string)
            n615 = local write "Data Folder"(w1466) -> ()
            n616 = List Folder(path=w1466) -> (filenames=w1476:string[], error out=w1433:errorcluster)  [unwired: 3 in, 2 out]
            n617 = Array Size(array=w1476) -> (size(s)=w1421:i32)
            n618 = Search 1D Array(1D array=w1476, element=w1482) -> (index of element=w1477:i32)  [unwired: 1 in]
            n619 = Equal To 0?(x=w1477) -> (x = 0?=w1478:bool)
            n620 = local read "Folder Index"() -> (w1420:dbl)
            n621 = property on="Image Out" class="ImageControl"() -> (error out=w1423:errorcluster, "Image Center Position"=w1427:cluster{"X":u32, "Y":u32})  [unwired: 2 in, 1 out]
            n622 = case shown="True" w1478 {
              tunnel: w1420 -> [w1612 _]
              tunnel: [w1611 w1613] -> w1419
              tunnel: w1421 -> [_ w1614]
              frame False {
                n623 = Decrement(x=w1612) -> (x-1=w1611:dbl)
              }
              frame True {
                n624 = Decrement(x=w1614) -> (x-1=w1613:i32)
              }
            }
            n625 = Unbundle(w1427) -> ("X"=w1425:u32)  [unwired: 1 out]
            n626 = local write "Folder Index"(w1419) -> ()
            n627 = Bundle("X"=w1425, 0) -> (w1426:cluster{"X":u32, i32})  [unwired: 1 in]
            n628 = Path To String(path=w1466) -> (string=w1483:string)
            n629 = Index Array(array=w1476, index=w1419) -> (element=w1479:string)
            n630 = local write "Data Name:"(w1479) -> ()
            n631 = property on="Image Out" class="ImageControl"(error in=w1423, "Image Center Position"=w1426) -> ()  [unwired: 1 in, 2 out]
            n632 = Concatenate Strings(w1483, "\\", w1479) -> (w1481:string)
            n633 = String To Path(string=w1481) -> (path=w1370:path)
            n634 = call "Recorded Values.vi"("Path"=w1370) -> ("Recorded Char"=w1417:T5, "Recorded Prop"=w1416:T6, "Fabrication Prop"=w1418:T7)  [unwired: 8 in]
            n635 = Unbundle By Name(w1417) -> ("Mobility-Sat"=w1404:dbl, "Moblitity-Lin"=w1403:dbl, "On/Off"=w1402:dbl, "Off Current"=w1401:dbl, "Vt-Sat"=w1366:dbl, "STS"=w1400:dbl, "Trap Density-VT"=w1399:dbl, "Trap Density-STS"=w1398:dbl)
            n636 = Unbundle By Name(w1418) -> ("Date Created"=w1397:string, "Material"=w1415:string, "Solvent"=w1414:string, "Concentration"=w1413:dbl, "Method"=w1412:string, "Dielectric (nm)"=w1411:dbl, "Treatment"=w1410:string, "Comments"=w1409:string)
            n637 = Unbundle By Name(w1416) -> ("Date Recorded"=w1408:string, "Index"=w1407:string, "Length"=w1406:dbl, "Width"=w1405:dbl, "Sample Temp"=w1367:dbl)
            n638 = local write "Date Created"(w1397) -> ()
            n639 = local write "Rec: Material"(w1415) -> ()
            n640 = local write "Rec: Off I-Sat"(w1401) -> ()
            n641 = local write "Rec: VT-Sat"(w1366) -> ()
            n642 = local write "Rec: Solvent"(w1414) -> ()
            n643 = local write "Rec: Concentration"(w1413) -> ()
            n644 = local write "Rec: Method"(w1412) -> ()
            n645 = local write "Rec: Dielectric (d)"(w1411) -> ()
            n646 = local write "Surface Treatment:"(w1410) -> ()
            n647 = local write "Comments"(w1409) -> ()
            n648 = local write "Index"(w1407) -> ()
            n649 = local write "Rec: Mobility-Sat"(w1404) -> ()
            n650 = local write "Rec: Mobility-Lin"(w1403) -> ()
            n651 = local write "Rec: On/Off"(w1402) -> ()
            n652 = local write "Rec: STS"(w1400) -> ()
            n653 = local write "Rec: Trap Density-VT"(w1399) -> ()
            n654 = local write "Rec: Trap Density-STS"(w1398) -> ()
            n655 = local write "Date Recorded"(w1408) -> ()
            n656 = local write "Rec: Length"(w1406) -> ()
            n657 = local write "Rec: Width"(w1405) -> ()
            n658 = local write "Rec: Temp"(w1367) -> ()
            n659 = Equal To 0?(x=w1367) -> (x = 0?=w1369:bool)
            n660 = case shown="False" w1369 {
              tunnel: [w1484 w1485] -> w1368
              tunnel: w1367 -> [w1484 _]
              frame False {
              }
              frame True {
                n661 = local read "Room Temp"() -> (w1485:dbl)
              }
            }
            n662 = local read "NumPts 2"() -> (w1392:dbl)
            n663 = local write "Data File"(w1370) -> ()
            n664 = local read "NumPts"() -> (w1396:dbl)
            n665 = local read "New: Dielectric"() -> (w1376:dbl)
            n666 = call "Mobility-Vt Calculator-File.vi"("NumPts"=w1396, "Path"=w1370) -> ("XY Graph-Sat"=w1394:cluster{dbl[], dbl[]}[], "XY Graph-Lin"=w1365:cluster{dbl[], dbl[]}[], "Output"=w1395:T8, "Index-Sat"=w1393:dbl, "Index-Lin"=w1380:dbl)  [unwired: 4 in, 1 out]
            n667 = call "STS Calculator-File.vi"("NumPts"=w1392, "Path"=w1370) -> ("STS Index-Sat"=w1391:dbl, "XY Graph-Sat"=w1390:cluster{dbl[], dbl[]}[], "Ouput"=w1389:cluster{"STS-Sat":dbl, "STS-Lin":dbl})  [unwired: 5 in, 2 out]
            n668 = call-poly <vilib>:"Read From Spreadsheet File.vi"("file path (dialog if empty)"=w1370) -> ("all rows"=w1473:string[][])  [unwired: 6 in, 4 out]
            n669 = Unbundle By Name(w1395) -> ("Mobility-Sat"=w1379:dbl, "Vt-Sat"=w1372:dbl, "Mobility-Lin"=w1378:dbl, "Vt-Lin"=w1377:dbl, "Off I-Sat"=w1371:dbl, "On/Off I-Sat"=w1364:dbl)
            n670 = Unbundle By Name(w1389) -> ("STS-Sat"=w1373:dbl)  [unwired: 1 out]
            n671 = local write "Index 2"(w1391) -> ()
            n672 = local write "XY Graph 2"(w1390) -> ()
            n673 = local write "MobVi Index"(w1393) -> ()
            n674 = local write "Slide"(w1393) -> ()
            n675 = local write "XY Graph"(w1394) -> ()
            n676 = local write "Calc: Mobility-Sat"(w1379) -> ()
            n677 = local write "Calc: VT-Sat"(w1372) -> ()
            n678 = local write "Calc: Mobility-Lin"(w1378) -> ()
            n679 = local write "Calc: Off I-Sat"(w1371) -> ()
            n680 = local write "Calc: On/Off"(w1364) -> ()
            n681 = Array Size(array=w1473) -> (size(s)=w1472:i32[])
            n682 = local write "Calc: VT-Lin"(w1377) -> ()
            n683 = call "Trap Density_VT.vi"("VT"=w1372, "Dielectric"=w1376) -> ("Trap Density-VT"=w1375:dbl)
            n684 = call "Trap Density_STS.vi"("Temp (T) [K]"=w1368, "S.T.S. (S)"=w1373, "Dielectric"=w1376) -> ("Trap Density (N)"=w1374:dbl)  [unwired: 8 in]
            n685 = local write "Calc: STS"(w1373) -> ()
            n686 = local write "New: STS"(w1373) -> ()
            n687 = Decimate 1D Array(w1365) -> (w1388:cluster{dbl[], dbl[]}[])  [unwired: 1 out]
            n688 = local write "Calc: Trap Density-VT"(w1375) -> ()
            n689 = local write "New: VT-Sat"(w1372) -> ()
            n690 = local write "Calc: Trap Density-STS"(w1374) -> ()
            n691 = local write "New: Trap Density-STS"(w1374) -> ()
            n692 = local write "New: Trap Density-VT"(w1375) -> ()
            n693 = local write "XY Graph-Lin"(w1365) -> ()
            n694 = local write "New: VT-Lin"(w1377) -> ()
            n695 = local write "New: Mobility-Sat"(w1379) -> ()
            n696 = local write "New: Mobility-Lin"(w1378) -> ()
            n697 = Decimate 1D Array(w1390) -> (w1450:cluster{dbl[], dbl[]}[])  [unwired: 1 out]
            n698 = Index Array(array=w1472, index=w1471) -> (element=w1456:i32)
            n699 = Decimate 1D Array(w1394) -> (w1460:cluster{dbl[], dbl[]}[])  [unwired: 1 out]
            n700 = Array To Cluster(array=w1388) -> (cluster=w1387:T9)
            n701 = Array Subset(array=w1473, index (row)=w1471, index (col)=w1471, length (col)=3) -> (w1474:string[][])  [unwired: 1 in]
            n702 = Array To Cluster(array=w1450) -> (cluster=w1448:T9)
            n703 = Array To Cluster(array=w1460) -> (cluster=w1462:T9)
            n704 = Reshape Array(w1474, w1456) -> (w1463:string[])
            n705 = Subtract(x=w1456, y=20) -> (x-y=w1455:i32)
            n706 = Unbundle(w1387) -> ("[0]"=w1384:cluster{dbl[], dbl[]})  [unwired: 8 out]
            n707 = property on="Slide" class="Slide (strict)"("Scale.Maximum"=w1455) -> ()  [unwired: 2 in, 2 out]
            n708 = Unbundle(w1448) -> ("[0]"=w1449:cluster{dbl[], dbl[]})  [unwired: 8 out]
            n709 = Unbundle(w1462) -> ("[0]"=w1461:cluster{dbl[], dbl[]})  [unwired: 8 out]
            n710 = local read "NumPts"() -> (w1381:dbl)
            n711 = Unbundle(w1384) -> (w1383:dbl[], w1382:dbl[])
            n712 = Search 1D Array(1D array=w1463, element="Index:") -> (index of element=w1468:i32)  [unwired: 1 in]
            n713 = Increment(x=w1468) -> (x+1=w1469:i32)
            n714 = Unbundle(w1449) -> (w1447:dbl[], w1446:dbl[])
            n715 = Unbundle(w1461) -> (w1454:dbl[], w1453:dbl[])
            n716 = Array Subset(array=w1383, index=w1380, length=w1381) -> (w1385:dbl[])
            n717 = Array Subset(array=w1382, index=w1380, length=w1381) -> (w1386:dbl[])
            n718 = local read "Image Folder"() -> (w1422:path)
            n719 = local write "Lin-Vg Array-Used"(w1385) -> ()
            n720 = Array Subset(array=w1447, index=w1391, length=w1392) -> (w1452:dbl[])
            n721 = Array Subset(array=w1446, index=w1391, length=w1392) -> (w1451:dbl[])
            n722 = Array Subset(array=w1454, index=w1393, length=w1396) -> (w1459:dbl[])
            n723 = Array Subset(array=w1453, index=w1393, length=w1396) -> (w1458:dbl[])
            n724 = local write "Lin Id-Used"(w1386) -> ()
            n725 = Index Array(array=w1463, index=w1469) -> (element=w1429:string)
            n726 = local write "Sat Vg Array-Used"(w1459) -> ()
            n727 = local write "Vg Array-Log-Used"(w1451) -> ()
            n728 = local write "Sat Id-Log-Used"(w1452) -> ()
            n729 = local write "Sat Id-Used"(w1458) -> ()
            n730 = local write "Index"(w1429) -> ()
            n731 = List Folder(path=w1422, error in=w1433) -> (filenames=w1465:string[], error out=w1432:errorcluster)  [unwired: 2 in, 2 out]
            n732 = Build Path(base path=w1422, name or relative path="ROI") -> (appended path=w1430:path)
            n733 = while {
              tunnel: w1465 -> [w1498]
              tunnel: w1429 -> [w1496]
              tunnel: [w1495] -> w1464
              tunnel: w1456 -> [w1494]
              i -> [w1495]
              stop <- w1491 stop-if-true
              n734 = Index Array(array=w1498, index=w1495) -> (element=w1499:string)
              n735 = xnode "Match Regular Expression"("input string"=w1499, "regular expression"=w1496) -> ("whole match"=w1497:string)  [unwired: 4 in, 4 out]
              n736 = Equal?(x=w1497, y=w1496) -> (x = y?=w1493:bool)
              n737 = Equal?(x=w1494, y=w1495) -> (x = y?=w1492:bool)
              n738 = Or(x=w1493, y=w1492) -> (x .or. y?=w1491:bool)
            }
            n739 = invoke on="Image Out" class="ImageControl" method="Clear ROI"(error in=w1432) -> (error out=w1436:errorcluster)  [unwired: 2 in, 2 out]
            n740 = Build Path(base path=w1430, name or relative path=w1429) -> (appended path=w1428:path)
            n741 = call <vilib>:"Check if File or Folder Exists.vi"("error in (no error)"=w1436, "path"=w1428) -> ("file or folder exists?"=w1434:bool, "dup path"=w1435:path)  [unwired: 7 in, 1 out]
            n742 = case shown="True" w1434 {
              tunnel: w1435 -> [_ w1486]
              frame False {
              }
              frame True {
                n743 = Read from Text File(file (use dialog)=w1486) -> (text=w1490:string)  [unwired: 3 in, 3 out]
                n744 = property on="Image Out" class="ImageControl"() -> ("ROI"=w1487:T10)  [unwired: 2 in, 2 out]
                n745 = Unflatten From String(type=w1487, binary string=w1490) -> (value=w1488:T10, error out=w1489:errorcluster)  [unwired: 3 in, 1 out]
                n746 = property on="Image Out" class="ImageControl"(error in=w1489, "ROI"=w1488) -> ()  [unwired: 1 in, 2 out]
              }
            }
            n747 = Index Array(array=w1465, index=w1464) -> (element=w1438:string)
            n748 = local write "Image Name"(w1438) -> ()
            n749 = Empty String/Path?(string/path=w1438) -> (empty?=w1445:bool)
            n750 = Build Path(base path=w1422, name or relative path=w1438) -> (appended path=w1437:path)
            n751 = local read "No Image"() -> (w1444:path)
            n752 = Select(t=w1444, s=w1445, f=w1437) -> (s? t:f=w1439:path)
            n753 = call <vilib>:"Get File Extension.vi"("file"=w1439) -> ("lowercase file extension"=w1441:string)  [unwired: 7 in, 3 out]
            n754 = local write "Image File"(w1439) -> ()
            n755 = local write "String"(w1441) -> ()
            n756 = Search 1D Array(1D array=string[] ["bmp", "jpeg", "png", "jpg", "gif"], element=w1441) -> (index of element=w1440:i32)  [unwired: 1 in]
            n757 = call "Vision Acquisition5"("Image Path"=w1439) -> ("Image Out"=w1443:T2)  [unwired: 25 in, 1 out]
            n758 = Less Than 0?(x=w1440) -> ()  [unwired: 1 out]
            n759 = local write "Image Out"(w1443) -> ()
            n760 = local write "Image Out 2"(w1443) -> ()
          }
          event "Save Changes? 3": Mouse Down {
            n761 = event-data() -> ()  [unwired: 1 in, 7 out]
            n762 = local read "Image Folder"() -> (w1615:path)
            n763 = Build Path(base path=w1615, name or relative path="ROI") -> (appended path=w1622:path)
            n764 = call <vilib>:"Check if File or Folder Exists.vi"("path"=w1622) -> ("file or folder exists?"=w1624:bool, "dup path"=w1621:path)  [unwired: 8 in, 1 out]
            n765 = case shown="False" w1624 {
              tunnel: w1621 -> [w1626 w1627]
              tunnel: [w1625 w1627] -> w1616
              frame False {
                n766 = Create Folder(path (use dialog)=w1626) -> (created path=w1625:path)  [unwired: 2 in, 2 out]
              }
              frame True {
              }
            }
            n767 = local read "Index"() -> (w1618:string)
            n768 = property on="Image Out" class="ImageControl"() -> ("ROI"=w1620:T10)  [unwired: 2 in, 2 out]
            n769 = Build Path(base path=w1616, name or relative path=w1618) -> (appended path=w1617:path)
            n770 = Flatten To String(anything=w1620) -> (data string=w1619:string)  [unwired: 3 in, 2 out]
            n771 = Write to Text File(file (use dialog)=w1617, text=w1619) -> ()  [unwired: 2 in, 3 out]
          }
          event "Next Button": Mouse Down {
            n772 = event-data() -> ()  [unwired: 1 in, 5 out]
            n773 = local read "XY Graph"() -> (w1640:cluster{dbl[], dbl[]}[])
            n774 = Decimate 1D Array(w1640) -> (w1636:cluster{dbl[], dbl[]}[], w1635:cluster{dbl[], dbl[]}[])
            n775 = Array To Cluster(array=w1636) -> (cluster=w1646:T9)
            n776 = local read "MobVi Index"() -> (w1642:dbl)
            n777 = Unbundle(w1646) -> ("[0]"=w1645:cluster{dbl[], dbl[]})  [unwired: 8 out]
            n778 = local read "NumPts"() -> (w1641:dbl)
            n779 = Unbundle(w1645) -> (w1644:dbl[], w1643:dbl[])
            n780 = Increment(x=w1642) -> (x+1=w1637:dbl)
            n781 = local read "New: Dielectric"() -> (w1631:dbl)
            n782 = local read "New: Length"() -> (w1630:dbl)
            n783 = local read "New: Width"() -> (w1629:dbl)
            n784 = local write "MobVi Index"(w1637) -> ()
            n785 = Array Subset(array=w1644, index=w1637, length=w1641) -> (w1633:dbl[])
            n786 = Array Subset(array=w1643, index=w1637, length=w1641) -> (w1632:dbl[])
            n787 = local write "Sat Vg Array-Used"(w1633) -> ()
            n788 = local write "Sat Id-Used"(w1632) -> ()
            n789 = call "Mobility-Vt-Used Pts_Saturation.vi"("Width"=w1629, "Length"=w1630, "Dielectric (d)"=w1631, "Sat Id Used"=w1632, "Vg Used"=w1633) -> ("Vt"=w1628:dbl, "Mobility"=w1634:dbl)  [unwired: 4 in, 1 out]
            n790 = Bundle(w1633, w1632) -> (w1639:cluster{dbl[], dbl[]})  [unwired: 1 in]
            n791 = Build Array (concatenate)(w1636, w1635, w1639) -> (w1638:cluster{dbl[], dbl[]}[])
            n792 = local write "New: Mobility-Sat"(w1634) -> ()
            n793 = local write "New: VT-Sat"(w1628) -> ()
            n794 = local write "XY Graph"(w1638) -> ()
          }
          event "Next Button 2": Mouse Down {
            n795 = event-data() -> ()  [unwired: 1 in, 7 out]
            n796 = local read "XY Graph 2"() -> (w1655:cluster{dbl[], dbl[]}[])
            n797 = Decimate 1D Array(w1655) -> (w1651:cluster{dbl[], dbl[]}[], w1650:cluster{dbl[], dbl[]}[])
            n798 = Array To Cluster(array=w1651) -> (cluster=w1661:T9)
            n799 = local read "Index 2"() -> (w1657:dbl)
            n800 = Unbundle(w1661) -> ("[0]"=w1660:cluster{dbl[], dbl[]})  [unwired: 8 out]
            n801 = local read "NumPts 2"() -> (w1656:dbl)
            n802 = Unbundle(w1660) -> (w1659:dbl[], w1658:dbl[])
            n803 = Increment(x=w1657) -> (x+1=w1652:dbl)
            n804 = local write "Index 2"(w1652) -> ()
            n805 = Array Subset(array=w1658, index=w1652, length=w1656) -> (w1647:dbl[])
            n806 = Array Subset(array=w1659, index=w1652, length=w1656) -> (w1648:dbl[])
            n807 = call "STS-Used.vi"("Id Used"=w1648, "Vg-Used"=w1647) -> ("STS"=w1649:dbl)  [unwired: 9 in]
            n808 = Bundle(w1648, w1647) -> (w1654:cluster{dbl[], dbl[]})  [unwired: 1 in]
            n809 = local write "Vg Array-Log-Used"(w1647) -> ()
            n810 = local write "Sat Id-Log-Used"(w1648) -> ()
            n811 = local write "New: STS"(w1649) -> ()
            n812 = Build Array (concatenate)(w1651, w1650, w1654) -> (w1653:cluster{dbl[], dbl[]}[])
            n813 = local write "XY Graph 2"(w1653) -> ()
          }
          event "Previous Button 2": Mouse Down {
            n814 = event-data() -> ()  [unwired: 1 in, 7 out]
            n815 = local read "XY Graph 2"() -> (w1671:cluster{dbl[], dbl[]}[])
            n816 = Decimate 1D Array(w1671) -> (w1668:cluster{dbl[], dbl[]}[], w1667:cluster{dbl[], dbl[]}[])
            n817 = Array To Cluster(array=w1668) -> (cluster=w1676:T9)
            n818 = local read "Index 2"() -> (w1664:dbl)
            n819 = Unbundle(w1676) -> ("[0]"=w1675:cluster{dbl[], dbl[]})  [unwired: 8 out]
            n820 = local read "NumPts 2"() -> (w1672:dbl)
            n821 = Unbundle(w1675) -> (w1674:dbl[], w1673:dbl[])
            n822 = Decrement(x=w1664) -> (x-1=w1665:dbl)
            n823 = local write "Index 2"(w1665) -> ()
            n824 = Array Subset(array=w1674, index=w1665, length=w1672) -> (w1662:dbl[])
            n825 = Array Subset(array=w1673, index=w1665, length=w1672) -> (w1663:dbl[])
            n826 = local write "Vg Array-Log-Used"(w1663) -> ()
            n827 = local write "Sat Id-Log-Used"(w1662) -> ()
            n828 = Bundle(w1662, w1663) -> (w1670:cluster{dbl[], dbl[]})  [unwired: 1 in]
            n829 = call "STS-Used.vi"("Id Used"=w1662, "Vg-Used"=w1663) -> ("STS"=w1666:dbl)  [unwired: 9 in]
            n830 = Build Array (concatenate)(w1668, w1667, w1670) -> (w1669:cluster{dbl[], dbl[]}[])
            n831 = local write "New: STS"(w1666) -> ()
            n832 = local write "XY Graph 2"(w1669) -> ()
          }
          event "Previous Button": Mouse Down {
            n833 = event-data() -> ()  [unwired: 1 in, 5 out]
            n834 = local read "XY Graph"() -> (w1690:cluster{dbl[], dbl[]}[])
            n835 = Decimate 1D Array(w1690) -> (w1687:cluster{dbl[], dbl[]}[], w1686:cluster{dbl[], dbl[]}[])
            n836 = Array To Cluster(array=w1687) -> (cluster=w1695:T9)
            n837 = local read "MobVi Index"() -> (w1685:dbl)
            n838 = Unbundle(w1695) -> ("[0]"=w1694:cluster{dbl[], dbl[]})  [unwired: 8 out]
            n839 = local read "NumPts"() -> (w1691:dbl)
            n840 = Unbundle(w1694) -> (w1693:dbl[], w1692:dbl[])
            n841 = Decrement(x=w1685) -> (x-1=w1684:dbl)
            n842 = local read "New: Dielectric"() -> (w1678:dbl)
            n843 = local read "New: Length"() -> (w1679:dbl)
            n844 = local read "New: Width"() -> (w1680:dbl)
            n845 = local write "MobVi Index"(w1684) -> ()
            n846 = Array Subset(array=w1693, index=w1684, length=w1691) -> (w1683:dbl[])
            n847 = Array Subset(array=w1692, index=w1684, length=w1691) -> (w1682:dbl[])
            n848 = local write "Sat Vg Array-Used"(w1683) -> ()
            n849 = local write "Sat Id-Used"(w1682) -> ()
            n850 = call "Mobility-Vt-Used Pts_Linear.vi"("Width"=w1680, "Length"=w1679, "Dielectric (d)"=w1678, "Sat Id Used"=w1682, "Vg Used"=w1683) -> ("Vt"=w1677:dbl, "Mobility"=w1681:dbl)  [unwired: 4 in, 1 out]
            n851 = Bundle(w1683, w1682) -> (w1689:cluster{dbl[], dbl[]})  [unwired: 1 in]
            n852 = local write "New: VT-Sat"(w1677) -> ()
            n853 = Build Array (concatenate)(w1687, w1686, w1689) -> (w1688:cluster{dbl[], dbl[]}[])
            n854 = local write "New: Mobility-Sat"(w1681) -> ()
            n855 = local write "XY Graph"(w1688) -> ()
          }
          event "Slide": Value Change {
            n856 = event-data() -> ()  [unwired: 1 in, 5 out]
            n857 = local read "XY Graph"() -> (w1708:cluster{dbl[], dbl[]}[])
            n858 = Decimate 1D Array(w1708) -> (w1705:cluster{dbl[], dbl[]}[], w1704:cluster{dbl[], dbl[]}[])
            n859 = Array To Cluster(array=w1705) -> (cluster=w1713:T9)
            n860 = Unbundle(w1713) -> ("[0]"=w1712:cluster{dbl[], dbl[]})  [unwired: 8 out]
            n861 = local read "NumPts"() -> (w1709:dbl)
            n862 = local read "Slide"() -> (w1697:dbl)
            n863 = Unbundle(w1712) -> (w1711:dbl[], w1710:dbl[])
            n864 = local read "New: Dielectric"() -> (w1698:dbl)
            n865 = local read "New: Length"() -> (w1699:dbl)
            n866 = local read "New: Width"() -> (w1700:dbl)
            n867 = local write "MobVi Index"(w1697) -> ()
            n868 = Array Subset(array=w1711, index=w1697, length=w1709) -> (w1703:dbl[])
            n869 = Array Subset(array=w1710, index=w1697, length=w1709) -> (w1702:dbl[])
            n870 = local write "Sat Vg Array-Used"(w1703) -> ()
            n871 = local write "Sat Id-Used"(w1702) -> ()
            n872 = call "Mobility-Vt-Used Pts_Linear.vi"("Width"=w1700, "Length"=w1699, "Dielectric (d)"=w1698, "Sat Id Used"=w1702, "Vg Used"=w1703) -> ("Vt"=w1696:dbl, "Mobility"=w1701:dbl)  [unwired: 4 in, 1 out]
            n873 = Bundle(w1703, w1702) -> (w1707:cluster{dbl[], dbl[]})  [unwired: 1 in]
            n874 = local write "New: VT-Sat"(w1696) -> ()
            n875 = Build Array (concatenate)(w1705, w1704, w1707) -> (w1706:cluster{dbl[], dbl[]}[])
            n876 = local write "New: Mobility-Sat"(w1701) -> ()
            n877 = local write "XY Graph"(w1706) -> ()
          }
          event "Slide 2": Value Change {
            n878 = event-data() -> ()  [unwired: 1 in, 5 out]
            n879 = local read "XY Graph 2"() -> (w1722:cluster{dbl[], dbl[]}[])
            n880 = Decimate 1D Array(w1722) -> (w1719:cluster{dbl[], dbl[]}[], w1718:cluster{dbl[], dbl[]}[])
            n881 = Array To Cluster(array=w1719) -> (cluster=w1727:T9)
            n882 = Unbundle(w1727) -> ("[0]"=w1726:cluster{dbl[], dbl[]})  [unwired: 8 out]
            n883 = local read "NumPts 2"() -> (w1723:dbl)
            n884 = local read "Slide 2"() -> (w1717:dbl)
            n885 = Unbundle(w1726) -> (w1725:dbl[], w1724:dbl[])
            n886 = local write "Index 2"(w1717) -> ()
            n887 = Array Subset(array=w1725, index=w1717, length=w1723) -> (w1715:dbl[])
            n888 = Array Subset(array=w1724, index=w1717, length=w1723) -> (w1714:dbl[])
            n889 = local write "Vg Array-Log-Used"(w1714) -> ()
            n890 = local write "Sat Id-Log-Used"(w1715) -> ()
            n891 = call "STS-Used.vi"("Id Used"=w1715, "Vg-Used"=w1714) -> ("STS"=w1716:dbl)  [unwired: 9 in]
            n892 = Bundle(w1715, w1714) -> (w1721:cluster{dbl[], dbl[]})  [unwired: 1 in]
            n893 = local write "New: STS"(w1716) -> ()
            n894 = Build Array (concatenate)(w1719, w1718, w1721) -> (w1720:cluster{dbl[], dbl[]}[])
            n895 = local write "XY Graph 2"(w1720) -> ()
          }
          event "Save Changes?": Mouse Down {
            n896 = event-data() -> ()  [unwired: 1 in, 5 out]
            n897 = flat-sequence {
              tunnel: [w1755] -> w1732
              tunnel: [w1749] -> w1731
              tunnel: [w1735] -> w1730
              tunnel: w1732 -> [w2054]
              tunnel: w1731 -> [w2051]
              tunnel: [w2052] -> w1729
              tunnel: w1730 -> [w2052]
              tunnel: [w2051] -> w1728
              tunnel: w1729 -> [w2059]
              tunnel: w1728 -> [w2058]
              frame #0 {
                n898 = local read "New: Temp"() -> (w1736:dbl)
                n899 = local read "Data File"() -> (w1755:path)
                n900 = local read "New: Length"() -> (w1740:dbl)
                n901 = local read "New: Width"() -> (w1738:dbl)
                n902 = To Single Precision Float(number=w1736) -> (single precision float=w1737:sgl)
                n903 = call-poly <vilib>:"Read From Spreadsheet File.vi"("file path (dialog if empty)"=w1755) -> ("all rows"=w1733:string[][])  [unwired: 6 in, 4 out]
                n904 = Number To Decimal String(number=w1737) -> (decimal integer string=w1752:string)  [unwired: 1 in]
                n905 = To Single Precision Float(number=w1738) -> (single precision float=w1739:sgl)
                n906 = To Single Precision Float(number=w1740) -> (single precision float=w1741:sgl)
                n907 = local read "Index"() -> (w1758:string)
                n908 = Strip Path(path=w1755) -> (stripped path=w1763:path)  [unwired: 1 out]
                n909 = Number To Decimal String(number=w1741) -> (decimal integer string=w1756:string)  [unwired: 1 in]
                n910 = Number To Decimal String(number=w1739) -> (decimal integer string=w1757:string)  [unwired: 1 in]
                n911 = Array Size(array=w1733) -> (size(s)=w1746:i32[])
                n912 = Concatenate Strings("_", w1752, "K") -> (w1750:string)
                n913 = Array Subset(array=w1733, index (row)=0, index (col)=0, length (col)=3) -> (w1742:string[][])  [unwired: 1 in]
                n914 = Index Array(array=w1746, index=0) -> (element=w1748:i32)
                n915 = call "Build Text"("Temp"=w1750, "Index"=w1758, "Length"=w1756, "Width"=w1757) -> ("Result"=w1759:string)  [unwired: 10 in, 1 out]
                n916 = flat-sequence {
                  tunnel: [w2008] -> w1754
                  tunnel: w1754 -> [w2025]
                  frame #0 {
                    # "Makes Empty File for Transformer Data"
                    n917 = local read "Data Folder"() -> (w1997:path)
                    n918 = Build Path(base path=w1997, name or relative path="Stats") -> (appended path=w1999:path)
                    n919 = call <vilib>:"Check if File or Folder Exists.vi"("path"=w1999) -> ("file or folder exists?"=w2000:bool, "dup path"=w2001:path)  [unwired: 8 in, 1 out]
                    n920 = case shown="False" w2000 {
                      tunnel: [w2005 w2007] -> w2002
                      tunnel: w2001 -> [w2006 w2007]
                      frame False {
                        n921 = Create Folder(path (use dialog)=w2006) -> (created path=w2005:path)  [unwired: 2 in, 2 out]
                      }
                      frame True {
                      }
                    }
                    n922 = Build Path(base path=w2002, name or relative path="Tranformer Data.txt") -> (appended path=w2004:path)
                    n923 = call-poly <vilib>:"Write To Spreadsheet File.vi"("append to file? (new file:F)"=TRUE, "file path (dialog if empty)"=w2004) -> ()  [unwired: 6 in, 1 out]
                  }
                  frame #1 {
                    # "Adds Headers if they don't exist"
                    n924 = Concatenate Strings("Stats\\", "Tranformer Data.txt") -> (w2015:string)
                    n925 = local read "Data Folder"() -> (w2014:path)
                    n926 = Build Path(base path=w2014, name or relative path=w2015) -> (appended path=w2008:path)
                    n927 = call-poly <vilib>:"Read From Spreadsheet File.vi"("file path (dialog if empty)"=w2008) -> ("first row"=w2013:string[])  [unwired: 6 in, 4 out]
                    n928 = Search 1D Array(1D array=w2013, element="DeviceID") -> (index of element=w2011:i32)  [unwired: 1 in]
                    n929 = Equal?(x=w2011, y=0) -> (x = y?=w2009:bool)
                    n930 = case shown="False" w2009 {
                      tunnel: w2008 -> [w2019 _]
                      frame False {
                        n931 = local read "Transformer \nHeaders"() -> (w2018:string[])
                        n932 = call-poly <vilib>:"Write To Spreadsheet File.vi"("1D data"=w2018, "file path (dialog if empty)"=w2019) -> ()  [unwired: 6 in, 1 out]
                      }
                      frame True {
                      }
                    }
                  }
                  frame #2 {
                    # "Adds current device if it doesn't exist"
                    n933 = local read "Current \nRecord"() -> (w2024:string[])
                    n934 = Index Array(array=w2024, index=0) -> (element=w2023:string)
                    n935 = Concatenate Strings("Stats\\", "Tranformer Data.txt") -> (w2028:string)
                    n936 = local read "Data Folder"() -> (w2027:path)
                    n937 = local write "Current Device ID"(w2023) -> ()
                    n938 = local read "Current Device ID"() -> (w2033:string)
                    n939 = Build Path(base path=w2027, name or relative path=w2028) -> (appended path=w2026:path)
                    n940 = call-poly <vilib>:"Read From Spreadsheet File.vi"("file path (dialog if empty)"=w2026) -> ("all rows"=w2020:string[][])  [unwired: 6 in, 4 out]
                    n941 = Index Array(array=w2020, index (col)=0) -> (element=w2021:string[])  [unwired: 1 in]
                    n942 = Search 1D Array(1D array=w2021, element=w2033) -> (index of element=w2022:i32)  [unwired: 1 in]
                    n943 = Equal?(x=w2022, y=-1) -> (x = y?=w2035:bool)
                    n944 = case shown="False" w2035 {
                      tunnel: w2025 -> [w2038 w2049]
                      tunnel: w2022 -> [w2041 _]
                      tunnel: w2020 -> [w2042 _]
                      frame False {
                        n945 = local read "Current \nRecord"() -> (w2040:string[])
                        n946 = Replace Array Subset(array=w2042, new element=w2040, index (row)=w2041) -> (w2039:string[][])  [unwired: 1 in]
                        n947 = flat-sequence {
                          tunnel: w2038 -> [w2043]
                          tunnel: w2039 -> [w2044]
                          tunnel: [w2044] -> w2037
                          tunnel: [w2043] -> w2036
                          tunnel: w2037 -> [w2046]
                          tunnel: w2036 -> [w2045]
                          frame #0 {
                            n948 = Delete(path (use dialog)=w2043) -> ()  [unwired: 4 in, 3 out]
                          }
                          frame #1 {
                            n949 = call-poly <vilib>:"Write To Spreadsheet File.vi"("append to file? (new file:F)"=TRUE, "2D data"=w2046, "file path (dialog if empty)"=w2045) -> ()  [unwired: 5 in, 1 out]
                          }
                        }
                      }
                      frame True {
                        n950 = local read "Current \nRecord"() -> (w2048:string[])
                        n951 = call-poly <vilib>:"Write To Spreadsheet File.vi"("append to file? (new file:F)"=TRUE, "1D data"=w2048, "file path (dialog if empty)"=w2049) -> ()  [unwired: 5 in, 1 out]
                      }
                    }
                  }
                }
                n952 = Reshape Array(w1742, w1748) -> (w1734:string[])
                n953 = Path To String(path=w1763) -> (string=w1761:string)
                n954 = stacked-sequence {
                  tunnel: w1734 -> [w1770 w1783 w1801 w1819 w1837 w1855 w1871 w1891 w1909 w1926 w1944 w1962 w1980]
                  tunnel: [_ _ _ _ _ _ _ _ _ _ _ _ w1978] -> w1735
                  frame #0 {
                    n955 = Search 1D Array(1D array=w1770, element="Dielectric (nm):") -> (index of element=w1767:i32)  [unwired: 1 in]
                    n956 = Equal?(x=w1767, y=-1) -> (x = y?=w1766:bool)
                    n957 = local read "Save1 Array"() -> (w1765:string[][])
                    n958 = case shown="False" w1766 {
                      tunnel: w1765 -> [w1776 w1780]
                      tunnel: w1767 -> [w1772 _]
                      tunnel: [w1771 w1780] -> w1764
                      frame False {
                        n959 = local read "New: Dielectric"() -> (w1778:dbl)
                        n960 = Number To Fractional String(number=w1778) -> (F-format string=w1773:string)  [unwired: 3 in]
                        n961 = Divide(x=w1772, y=3) -> (x/y=w1775:dbl)
                        n962 = To Word Integer(number=w1775) -> (16bit integer=w1774:i16)
                        n963 = Replace Array Subset(array=w1776, new element=w1773, index (row)=w1774, index (col)=1) -> (w1771:string[][])
                      }
                      frame True {
                      }
                    }
                    n964 = local write "Save1 Array"(w1764) -> ()
                  }
                  frame #1 {
                    n965 = Search 1D Array(1D array=w1783, element="Length (um):") -> (index of element=w1785:i32)  [unwired: 1 in]
                    n966 = Equal?(x=w1785, y=-1) -> (x = y?=w1784:bool)
                    n967 = local read "Save1 Array"() -> (w1782:string[][])
                    n968 = case shown="False" w1784 {
                      tunnel: w1782 -> [w1795 w1798]
                      tunnel: w1785 -> [w1792 _]
                      tunnel: [w1791 w1798] -> w1781
                      frame False {
                        n969 = local read "New: Length"() -> (w1788:dbl)
                        n970 = Divide(x=w1792, y=3) -> (x/y=w1794:dbl)
                        n971 = Format Value(format string="%#g", value (0)=w1788) -> (output string=w1789:string)  [unwired: 1 in]
                        n972 = To Word Integer(number=w1794) -> (16bit integer=w1793:i16)
                        n973 = Replace Array Subset(array=w1795, new element=w1789, index (row)=w1793, index (col)=1) -> (w1791:string[][])
                      }
                      frame True {
                      }
                    }
                    n974 = local write "Save1 Array"(w1781) -> ()
                  }
                  frame #2 {
                    n975 = Search 1D Array(1D array=w1801, element="Width (um):") -> (index of element=w1803:i32)  [unwired: 1 in]
                    n976 = Equal?(x=w1803, y=-1) -> (x = y?=w1802:bool)
                    n977 = local read "Save1 Array"() -> (w1800:string[][])
                    n978 = case shown="False" w1802 {
                      tunnel: w1803 -> [w1811 _]
                      tunnel: w1800 -> [w1810 w1816]
                      tunnel: [w1809 w1816] -> w1799
                      frame False {
                        n979 = local read "New: Width"() -> (w1806:dbl)
                        n980 = Divide(x=w1811, y=3) -> (x/y=w1813:dbl)
                        n981 = To Word Integer(number=w1813) -> (16bit integer=w1812:i16)
                        n982 = Format Value(format string="%#g", value (0)=w1806) -> (output string=w1807:string)  [unwired: 1 in]
                        n983 = Replace Array Subset(array=w1810, new element=w1807, index (row)=w1812, index (col)=1) -> (w1809:string[][])
                      }
                      frame True {
                      }
                    }
                    n984 = local write "Save1 Array"(w1799) -> ()
                  }
                  frame #3 {
                    n985 = Search 1D Array(1D array=w1819, element="Sample Temp (K):") -> (index of element=w1821:i32)  [unwired: 1 in]
                    n986 = Equal?(x=w1821, y=-1) -> (x = y?=w1820:bool)
                    n987 = local read "Save1 Array"() -> (w1818:string[][])
                    n988 = case shown="False" w1820 {
                      tunnel: w1818 -> [w1831 w1834]
                      tunnel: w1821 -> [w1828 _]
                      tunnel: [w1827 w1834] -> w1817
                      frame False {
                        n989 = local read "New: Temp"() -> (w1825:dbl)
                        n990 = Divide(x=w1828, y=3) -> (x/y=w1830:dbl)
                        n991 = Format Value(format string="%#g", value (0)=w1825) -> (output string=w1824:string)  [unwired: 1 in]
                        n992 = To Word Integer(number=w1830) -> (16bit integer=w1829:i16)
                        n993 = Replace Array Subset(array=w1831, new element=w1824, index (row)=w1829, index (col)=1) -> (w1827:string[][])
                      }
                      frame True {
                      }
                    }
                    n994 = local write "Save1 Array"(w1817) -> ()
                  }
                  frame #4 {
                    n995 = Search 1D Array(1D array=w1837, element="Mobility-Sat (cm^2/Vs):") -> (index of element=w1839:i32)  [unwired: 1 in]
                    n996 = Equal?(x=w1839, y=-1) -> (x = y?=w1838:bool)
                    n997 = local read "Save1 Array"() -> (w1835:string[][])
                    n998 = case shown="False" w1838 {
                      tunnel: w1835 -> [w1849 w1852]
                      tunnel: w1839 -> [w1846 _]
                      tunnel: [w1845 w1852] -> w1836
                      frame False {
                        n999 = local read "New: Mobility-Sat"() -> (w1842:dbl)
                        n1000 = Divide(x=w1846, y=3) -> (x/y=w1848:dbl)
                        n1001 = To Word Integer(number=w1848) -> (16bit integer=w1847:i16)
                        n1002 = Format Value(format string="%#g", value (0)=w1842) -> (output string=w1843:string)  [unwired: 1 in]
                        n1003 = Replace Array Subset(array=w1849, new element=w1843, index (row)=w1847, index (col)=1) -> (w1845:string[][])
                      }
                      frame True {
                      }
                    }
                    n1004 = local write "Save1 Array"(w1836) -> ()
                  }
                  frame #5 {
                    n1005 = Search 1D Array(1D array=w1855, element="On/Off I-Sat:") -> (index of element=w1857:i32)  [unwired: 1 in]
                    n1006 = Equal?(x=w1857, y=-1) -> (x = y?=w1856:bool)
                    n1007 = local read "Save1 Array"() -> (w1854:string[][])
                    n1008 = case shown="False" w1856 {
                      tunnel: w1854 -> [w1867 w1870]
                      tunnel: w1857 -> [w1864 _]
                      tunnel: [w1863 w1870] -> w1853
                      frame False {
                        n1009 = local read "Calc: On/Off"() -> (w1860:dbl)
                        n1010 = Divide(x=w1864, y=3) -> (x/y=w1866:dbl)
                        n1011 = To Word Integer(number=w1866) -> (16bit integer=w1865:i16)
                        n1012 = Format Value(format string="%#g", value (0)=w1860) -> (output string=w1861:string)  [unwired: 1 in]
                        n1013 = Replace Array Subset(array=w1867, new element=w1861, index (row)=w1865, index (col)=1) -> (w1863:string[][])
                      }
                      frame True {
                      }
                    }
                    n1014 = local write "Save1 Array"(w1853) -> ()
                  }
                  frame #6 {
                    n1015 = Search 1D Array(1D array=w1871, element="Mobility-Lin (cm^2/Vs):") -> (index of element=w1875:i32)  [unwired: 1 in]
                    n1016 = Equal?(x=w1875, y=-1) -> (x = y?=w1874:bool)
                    n1017 = local read "Save1 Array"() -> (w1873:string[][])
                    n1018 = case shown="False" w1874 {
                      tunnel: w1873 -> [w1885 w1888]
                      tunnel: w1875 -> [w1882 _]
                      tunnel: [w1881 w1888] -> w1872
                      frame False {
                        n1019 = local read "Calc: Mobility-Lin"() -> (w1878:dbl)
                        n1020 = Divide(x=w1882, y=3) -> (x/y=w1884:dbl)
                        n1021 = To Word Integer(number=w1884) -> (16bit integer=w1883:i16)
                        n1022 = Format Value(format string="%#g", value (0)=w1878) -> (output string=w1879:string)  [unwired: 1 in]
                        n1023 = Replace Array Subset(array=w1885, new element=w1879, index (row)=w1883, index (col)=1) -> (w1881:string[][])
                      }
                      frame True {
                      }
                    }
                    n1024 = local write "Save1 Array"(w1872) -> ()
                  }
                  frame #7 {
                    n1025 = Search 1D Array(1D array=w1891, element="Off I-Sat (A):") -> (index of element=w1893:i32)  [unwired: 1 in]
                    n1026 = Equal?(x=w1893, y=-1) -> (x = y?=w1892:bool)
                    n1027 = local read "Save1 Array"() -> (w1890:string[][])
                    n1028 = case shown="False" w1892 {
                      tunnel: w1890 -> [w1903 w1906]
                      tunnel: w1893 -> [w1900 _]
                      tunnel: [w1899 w1906] -> w1889
                      frame False {
                        n1029 = local read "Calc: Off I-Sat"() -> (w1898:dbl)
                        n1030 = Divide(x=w1900, y=3) -> (x/y=w1902:dbl)
                        n1031 = Format Value(format string="%#g", value (0)=w1898) -> (output string=w1896:string)  [unwired: 1 in]
                        n1032 = To Word Integer(number=w1902) -> (16bit integer=w1901:i16)
                        n1033 = Replace Array Subset(array=w1903, new element=w1896, index (row)=w1901, index (col)=1) -> (w1899:string[][])
                      }
                      frame True {
                      }
                    }
                    n1034 = local write "Save1 Array"(w1889) -> ()
                  }
                  frame #8 {
                    n1035 = Search 1D Array(1D array=w1909, element="Vt-Sat (V):") -> (index of element=w1911:i32)  [unwired: 1 in]
                    n1036 = Equal?(x=w1911, y=-1) -> (x = y?=w1910:bool)
                    n1037 = local read "Save1 Array"() -> (w1908:string[][])
                    n1038 = case shown="False" w1910 {
                      tunnel: w1908 -> [w1919 w1923]
                      tunnel: w1911 -> [w1915 _]
                      tunnel: [w1914 w1923] -> w1907
                      frame False {
                        n1039 = local read "New: VT-Sat"() -> (w1921:dbl)
                        n1040 = Number To Fractional String(number=w1921) -> (F-format string=w1916:string)  [unwired: 3 in]
                        n1041 = Divide(x=w1915, y=3) -> (x/y=w1918:dbl)
                        n1042 = To Word Integer(number=w1918) -> (16bit integer=w1917:i16)
                        n1043 = Replace Array Subset(array=w1919, new element=w1916, index (row)=w1917, index (col)=1) -> (w1914:string[][])
                      }
                      frame True {
                      }
                    }
                    n1044 = local write "Save1 Array"(w1907) -> ()
                  }
                  frame #9 {
                    n1045 = Search 1D Array(1D array=w1926, element="VT-Lin (V):") -> (index of element=w1928:i32)  [unwired: 1 in]
                    n1046 = Equal?(x=w1928, y=-1) -> (x = y?=w1927:bool)
                    n1047 = local read "Save1 Array"() -> (w1925:string[][])
                    n1048 = case shown="False" w1927 {
                      tunnel: w1925 -> [w1938 w1941]
                      tunnel: w1928 -> [w1935 _]
                      tunnel: [w1934 w1941] -> w1924
                      frame False {
                        n1049 = local read "New: VT-Lin"() -> (w1932:dbl)
                        n1050 = Divide(x=w1935, y=3) -> (x/y=w1937:dbl)
                        n1051 = Format Value(format string="%#g", value (0)=w1932) -> (output string=w1931:string)  [unwired: 1 in]
                        n1052 = To Word Integer(number=w1937) -> (16bit integer=w1936:i16)
                        n1053 = Replace Array Subset(array=w1938, new element=w1931, index (row)=w1936, index (col)=1) -> (w1934:string[][])
                      }
                      frame True {
                      }
                    }
                    n1054 = local write "Save1 Array"(w1924) -> ()
                  }
                  frame #10 {
                    n1055 = Search 1D Array(1D array=w1944, element="STS-Sat (V/decade):") -> (index of element=w1946:i32)  [unwired: 1 in]
                    n1056 = Equal?(x=w1946, y=-1) -> (x = y?=w1945:bool)
                    n1057 = local read "Save1 Array"() -> (w1943:string[][])
                    n1058 = case shown="False" w1945 {
                      tunnel: w1943 -> [w1956 w1959]
                      tunnel: w1946 -> [w1953 _]
                      tunnel: [w1952 w1959] -> w1942
                      frame False {
                        n1059 = local read "New: STS"() -> (w1950:dbl)
                        n1060 = Divide(x=w1953, y=3) -> (x/y=w1955:dbl)
                        n1061 = Format Value(format string="%#g", value (0)=w1950) -> (output string=w1949:string)  [unwired: 1 in]
                        n1062 = To Word Integer(number=w1955) -> (16bit integer=w1954:i16)
                        n1063 = Replace Array Subset(array=w1956, new element=w1949, index (row)=w1954, index (col)=1) -> (w1952:string[][])
                      }
                      frame True {
                      }
                    }
                    n1064 = local write "Save1 Array"(w1942) -> ()
                  }
                  frame #11 {
                    n1065 = Search 1D Array(1D array=w1962, element="Trap Density-VT (Traps/Vcm^2):") -> (index of element=w1964:i32)  [unwired: 1 in]
                    n1066 = Equal?(x=w1964, y=-1) -> (x = y?=w1963:bool)
                    n1067 = local read "Save1 Array"() -> (w1961:string[][])
                    n1068 = case shown="False" w1963 {
                      tunnel: w1961 -> [w1974 w1977]
                      tunnel: w1964 -> [w1970 _]
                      tunnel: [w1969 w1977] -> w1960
                      frame False {
                        n1069 = local read "New: Trap Density-VT"() -> (w1968:dbl)
                        n1070 = Format Value(format string="%#g", value (0)=w1968) -> (output string=w1971:string)  [unwired: 1 in]
                        n1071 = Divide(x=w1970, y=3) -> (x/y=w1973:dbl)
                        n1072 = To Word Integer(number=w1973) -> (16bit integer=w1972:i16)
                        n1073 = Replace Array Subset(array=w1974, new element=w1971, index (row)=w1972, index (col)=1) -> (w1969:string[][])
                      }
                      frame True {
                      }
                    }
                    n1074 = local write "Save1 Array"(w1960) -> ()
                  }
                  frame #12 {
                    n1075 = Search 1D Array(1D array=w1980, element="Trap Density-STS (Traps/Vcm^2):") -> (index of element=w1982:i32)  [unwired: 1 in]
                    n1076 = Equal?(x=w1982, y=-1) -> (x = y?=w1981:bool)
                    n1077 = local read "Save1 Array"() -> (w1979:string[][])
                    n1078 = case shown="False" w1981 {
                      tunnel: w1979 -> [w1992 w1995]
                      tunnel: w1982 -> [w1989 _]
                      tunnel: [w1988 w1995] -> w1978
                      frame False {
                        n1079 = local read "New: Trap Density-STS"() -> (w1986:dbl)
                        n1080 = Divide(x=w1989, y=3) -> (x/y=w1991:dbl)
                        n1081 = To Word Integer(number=w1991) -> (16bit integer=w1990:i16)
                        n1082 = Format Value(format string="%#g", value (0)=w1986) -> (output string=w1985:string)  [unwired: 1 in]
                        n1083 = Replace Array Subset(array=w1992, new element=w1985, index (row)=w1990, index (col)=1) -> (w1988:string[][])
                      }
                      frame True {
                      }
                    }
                    n1084 = local write "Save1 Array"(w1978) -> ()
                  }
                }
                n1085 = Concatenate Strings(w1761, "\\", w1759) -> (w1760:string)
                n1086 = String To Path(string=w1760) -> (path=w1749:path)
                n1087 = local write "Save1 Array"(w1733) -> ()
              }
              frame #1 {
                n1088 = Equal?(x=w2054, y=w2051) -> (x = y?=w2053:bool)
                n1089 = case shown="False" w2053 {
                  tunnel: w2054 -> [w2057 _]
                  tunnel: w2051 -> [w2056 _]
                  frame False {
                    n1090 = Move(source path=w2057, 9:TRUE, 10:w2056) -> ()  [unwired: 2 in, 3 out]
                  }
                  frame True {
                  }
                }
              }
              frame #2 {
                n1091 = local write "Data File"(w2058) -> ()
                n1092 = call-poly <vilib>:"Write To Spreadsheet File.vi"("2D data"=w2059, "file path (dialog if empty)"=w2058) -> ()  [unwired: 6 in, 1 out]
              }
            }
          }
          event "Save Changes? 2": Mouse Down {
            n1093 = event-data() -> ()  [unwired: 1 in, 5 out]
            n1094 = stacked-sequence {
              seq-local: [w2119 _ _ _ _] -> [_ w2371 _ _ _]
              seq-local: [w2122 _ _ _ _] -> [_ w2372 _ _ _]
              seq-local: [w2119 _ _ _ _] -> [_ w2370 _ _ _]
              seq-local: [w2117 _ _ _ _] -> [_ w2368 _ _ _]
              seq-local: [_ w2372 _ _ _] -> [_ _ w2377 _ _]
              seq-local: [_ w2368 _ _ _] -> [_ _ w2376 _ _]
              frame #0 {
                n1095 = local read "New: Temp"() -> (w2121:dbl)
                n1096 = local read "Data File"() -> (w2122:path)
                n1097 = local read "New: Length"() -> (w2125:dbl)
                n1098 = local read "New: Width"() -> (w2123:dbl)
                n1099 = To Word Integer(number=w2121) -> (16bit integer=w2120:i16)
                n1100 = call-poly <vilib>:"Read From Spreadsheet File.vi"("file path (dialog if empty)"=w2122) -> ("all rows"=w2116:string[][])  [unwired: 6 in, 4 out]
                n1101 = Number To Decimal String(number=w2120) -> (decimal integer string=w2136:string)  [unwired: 1 in]
                n1102 = To Single Precision Float(number=w2123) -> (single precision float=w2124:sgl)
                n1103 = To Single Precision Float(number=w2125) -> (single precision float=w2126:sgl)
                n1104 = local read "Index"() -> (w2140:string)
                n1105 = Strip Path(path=w2122) -> (stripped path=w2145:path)  [unwired: 1 out]
                n1106 = Number To Decimal String(number=w2126) -> (decimal integer string=w2138:string)  [unwired: 1 in]
                n1107 = Number To Decimal String(number=w2124) -> (decimal integer string=w2139:string)  [unwired: 1 in]
                n1108 = Array Size(array=w2116) -> (size(s)=w2131:i32[])
                n1109 = Concatenate Strings("_", w2136, "K") -> (w2134:string)
                n1110 = Array Subset(array=w2116, index (row)=0, index (col)=0, length (col)=3) -> (w2127:string[][])  [unwired: 1 in]
                n1111 = Index Array(array=w2131, index=0) -> (element=w2133:i32)
                n1112 = call "Build Text2"("Temp"=w2134, "Index"=w2140, "Length"=w2138, "Width"=w2139) -> ("Result"=w2141:string)  [unwired: 10 in, 1 out]
                n1113 = Reshape Array(w2127, w2133) -> (w2118:string[])
                n1114 = Path To String(path=w2145) -> (string=w2143:string)
                n1115 = stacked-sequence {
                  tunnel: w2118 -> [w2152 w2165 w2182 w2199 w2216 w2233 w2248 w2267 w2285 w2302 w2319 w2336 w2353]
                  tunnel: [_ _ _ _ _ _ _ _ _ _ _ _ w2351] -> w2117
                  frame #0 {
                    n1116 = Search 1D Array(1D array=w2152, element="Dielectric (nm):") -> (index of element=w2149:i32)  [unwired: 1 in]
                    n1117 = Equal?(x=w2149, y=-1) -> (x = y?=w2148:bool)
                    n1118 = local read "Save1 Array"() -> (w2147:string[][])
                    n1119 = case shown="False" w2148 {
                      tunnel: w2147 -> [w2158 w2162]
                      tunnel: w2149 -> [w2154 _]
                      tunnel: [w2153 w2162] -> w2146
                      frame False {
                        n1120 = local read "New: Dielectric"() -> (w2160:dbl)
                        n1121 = Number To Fractional String(number=w2160) -> (F-format string=w2155:string)  [unwired: 3 in]
                        n1122 = Divide(x=w2154, y=3) -> (x/y=w2157:dbl)
                        n1123 = To Word Integer(number=w2157) -> (16bit integer=w2156:i16)
                        n1124 = Replace Array Subset(array=w2158, new element=w2155, index (row)=w2156, index (col)=1) -> (w2153:string[][])
                      }
                      frame True {
                      }
                    }
                    n1125 = local write "Save1 Array"(w2146) -> ()
                  }
                  frame #1 {
                    n1126 = Search 1D Array(1D array=w2165, element="Length (um):") -> (index of element=w2167:i32)  [unwired: 1 in]
                    n1127 = Equal?(x=w2167, y=-1) -> (x = y?=w2166:bool)
                    n1128 = local read "Save1 Array"() -> (w2164:string[][])
                    n1129 = case shown="True" w2166 {
                      tunnel: w2164 -> [w2175 w2179]
                      tunnel: w2167 -> [w2171 _]
                      tunnel: [w2170 w2179] -> w2163
                      frame False {
                        n1130 = local read "New: Length"() -> (w2177:dbl)
                        n1131 = Number To Fractional String(number=w2177) -> (F-format string=w2172:string)  [unwired: 3 in]
                        n1132 = Divide(x=w2171, y=3) -> (x/y=w2174:dbl)
                        n1133 = To Word Integer(number=w2174) -> (16bit integer=w2173:i16)
                        n1134 = Replace Array Subset(array=w2175, new element=w2172, index (row)=w2173, index (col)=1) -> (w2170:string[][])
                      }
                      frame True {
                      }
                    }
                    n1135 = local write "Save1 Array"(w2163) -> ()
                  }
                  frame #2 {
                    n1136 = Search 1D Array(1D array=w2182, element="Width (um):") -> (index of element=w2184:i32)  [unwired: 1 in]
                    n1137 = Equal?(x=w2184, y=-1) -> (x = y?=w2183:bool)
                    n1138 = local read "Save1 Array"() -> (w2181:string[][])
                    n1139 = case shown="False" w2183 {
                      tunnel: w2184 -> [w2189 _]
                      tunnel: w2181 -> [w2188 w2196]
                      tunnel: [w2187 w2196] -> w2180
                      frame False {
                        n1140 = local read "New: Width"() -> (w2194:dbl)
                        n1141 = Number To Fractional String(number=w2194) -> (F-format string=w2190:string)  [unwired: 3 in]
                        n1142 = Divide(x=w2189, y=3) -> (x/y=w2192:dbl)
                        n1143 = To Word Integer(number=w2192) -> (16bit integer=w2191:i16)
                        n1144 = Replace Array Subset(array=w2188, new element=w2190, index (row)=w2191, index (col)=1) -> (w2187:string[][])
                      }
                      frame True {
                      }
                    }
                    n1145 = local write "Save1 Array"(w2180) -> ()
                  }
                  frame #3 {
                    n1146 = Search 1D Array(1D array=w2199, element="Sample Temp (K):") -> (index of element=w2201:i32)  [unwired: 1 in]
                    n1147 = Equal?(x=w2201, y=-1) -> (x = y?=w2200:bool)
                    n1148 = local read "Save1 Array"() -> (w2198:string[][])
                    n1149 = case shown="False" w2200 {
                      tunnel: w2198 -> [w2209 w2213]
                      tunnel: w2201 -> [w2205 _]
                      tunnel: [w2204 w2213] -> w2197
                      frame False {
                        n1150 = local read "New: Temp"() -> (w2211:dbl)
                        n1151 = Number To Fractional String(number=w2211) -> (F-format string=w2206:string)  [unwired: 3 in]
                        n1152 = Divide(x=w2205, y=3) -> (x/y=w2208:dbl)
                        n1153 = To Word Integer(number=w2208) -> (16bit integer=w2207:i16)
                        n1154 = Replace Array Subset(array=w2209, new element=w2206, index (row)=w2207, index (col)=1) -> (w2204:string[][])
                      }
                      frame True {
                      }
                    }
                    n1155 = local write "Save1 Array"(w2197) -> ()
                  }
                  frame #4 {
                    n1156 = Search 1D Array(1D array=w2216, element="Mobility-Sat (cm^2/Vs):") -> (index of element=w2218:i32)  [unwired: 1 in]
                    n1157 = Equal?(x=w2218, y=-1) -> (x = y?=w2217:bool)
                    n1158 = local read "Save1 Array"() -> (w2214:string[][])
                    n1159 = case shown="False" w2217 {
                      tunnel: w2214 -> [w2226 w2230]
                      tunnel: w2218 -> [w2222 _]
                      tunnel: [w2221 w2230] -> w2215
                      frame False {
                        n1160 = local read "New: Mobility-Sat"() -> (w2228:dbl)
                        n1161 = Number To Fractional String(number=w2228) -> (F-format string=w2223:string)  [unwired: 3 in]
                        n1162 = Divide(x=w2222, y=3) -> (x/y=w2225:dbl)
                        n1163 = To Word Integer(number=w2225) -> (16bit integer=w2224:i16)
                        n1164 = Replace Array Subset(array=w2226, new element=w2223, index (row)=w2224, index (col)=1) -> (w2221:string[][])
                      }
                      frame True {
                      }
                    }
                    n1165 = local write "Save1 Array"(w2215) -> ()
                  }
                  frame #5 {
                    n1166 = Search 1D Array(1D array=w2233, element="Mobility-Lin (cm^2/Vs):") -> (index of element=w2235:i32)  [unwired: 1 in]
                    n1167 = Equal?(x=w2235, y=-1) -> (x = y?=w2234:bool)
                    n1168 = local read "Save1 Array"() -> (w2232:string[][])
                    n1169 = case shown="False" w2234 {
                      tunnel: w2232 -> [w2243 w2247]
                      tunnel: w2235 -> [w2239 _]
                      tunnel: [w2238 w2247] -> w2231
                      frame False {
                        n1170 = local read "Calc: Mobility-Lin"() -> (w2245:dbl)
                        n1171 = Number To Fractional String(number=w2245) -> (F-format string=w2240:string)  [unwired: 3 in]
                        n1172 = Divide(x=w2239, y=3) -> (x/y=w2242:dbl)
                        n1173 = To Word Integer(number=w2242) -> (16bit integer=w2241:i16)
                        n1174 = Replace Array Subset(array=w2243, new element=w2240, index (row)=w2241, index (col)=1) -> (w2238:string[][])
                      }
                      frame True {
                      }
                    }
                    n1175 = local write "Save1 Array"(w2231) -> ()
                  }
                  frame #6 {
                    n1176 = Search 1D Array(1D array=w2248, element="On/Off I-Sat:") -> (index of element=w2252:i32)  [unwired: 1 in]
                    n1177 = Equal?(x=w2252, y=-1) -> (x = y?=w2251:bool)
                    n1178 = local read "Save1 Array"() -> (w2250:string[][])
                    n1179 = case shown="False" w2251 {
                      tunnel: w2250 -> [w2260 w2264]
                      tunnel: w2252 -> [w2256 _]
                      tunnel: [w2255 w2264] -> w2249
                      frame False {
                        n1180 = local read "Calc: On/Off"() -> (w2262:dbl)
                        n1181 = Number To Fractional String(number=w2262) -> (F-format string=w2257:string)  [unwired: 3 in]
                        n1182 = Divide(x=w2256, y=3) -> (x/y=w2259:dbl)
                        n1183 = To Word Integer(number=w2259) -> (16bit integer=w2258:i16)
                        n1184 = Replace Array Subset(array=w2260, new element=w2257, index (row)=w2258, index (col)=1) -> (w2255:string[][])
                      }
                      frame True {
                      }
                    }
                    n1185 = local write "Save1 Array"(w2249) -> ()
                  }
                  frame #7 {
                    n1186 = Search 1D Array(1D array=w2267, element="Off I-Sat (A):") -> (index of element=w2269:i32)  [unwired: 1 in]
                    n1187 = Equal?(x=w2269, y=-1) -> (x = y?=w2268:bool)
                    n1188 = local read "Save1 Array"() -> (w2266:string[][])
                    n1189 = case shown="False" w2268 {
                      tunnel: w2266 -> [w2279 w2282]
                      tunnel: w2269 -> [w2276 _]
                      tunnel: [w2275 w2282] -> w2265
                      frame False {
                        n1190 = local read "Calc: Off I-Sat"() -> (w2274:dbl)
                        n1191 = Format Value(format string="%#g", value (0)=w2274) -> (output string=w2273:string)  [unwired: 1 in]
                        n1192 = Divide(x=w2276, y=3) -> (x/y=w2278:dbl)
                        n1193 = To Word Integer(number=w2278) -> (16bit integer=w2277:i16)
                        n1194 = Replace Array Subset(array=w2279, new element=w2273, index (row)=w2277, index (col)=1) -> (w2275:string[][])
                      }
                      frame True {
                      }
                    }
                    n1195 = local write "Save1 Array"(w2265) -> ()
                  }
                  frame #8 {
                    n1196 = Search 1D Array(1D array=w2285, element="Vt-Sat (V):") -> (index of element=w2287:i32)  [unwired: 1 in]
                    n1197 = Equal?(x=w2287, y=-1) -> (x = y?=w2286:bool)
                    n1198 = local read "Save1 Array"() -> (w2284:string[][])
                    n1199 = case shown="False" w2286 {
                      tunnel: w2284 -> [w2295 w2299]
                      tunnel: w2287 -> [w2291 _]
                      tunnel: [w2290 w2299] -> w2283
                      frame False {
                        n1200 = local read "New: VT-Sat"() -> (w2297:dbl)
                        n1201 = Number To Fractional String(number=w2297) -> (F-format string=w2292:string)  [unwired: 3 in]
                        n1202 = Divide(x=w2291, y=3) -> (x/y=w2294:dbl)
                        n1203 = To Word Integer(number=w2294) -> (16bit integer=w2293:i16)
                        n1204 = Replace Array Subset(array=w2295, new element=w2292, index (row)=w2293, index (col)=1) -> (w2290:string[][])
                      }
                      frame True {
                      }
                    }
                    n1205 = local write "Save1 Array"(w2283) -> ()
                  }
                  frame #9 {
                    n1206 = Search 1D Array(1D array=w2302, element="VT-Lin (V):") -> (index of element=w2304:i32)  [unwired: 1 in]
                    n1207 = Equal?(x=w2304, y=-1) -> (x = y?=w2303:bool)
                    n1208 = local read "Save1 Array"() -> (w2301:string[][])
                    n1209 = case shown="True" w2303 {
                      tunnel: w2301 -> [w2312 w2316]
                      tunnel: w2304 -> [w2308 _]
                      tunnel: [w2307 w2316] -> w2300
                      frame False {
                        n1210 = local read "New: VT-Lin"() -> (w2314:dbl)
                        n1211 = Number To Fractional String(number=w2314) -> (F-format string=w2309:string)  [unwired: 3 in]
                        n1212 = Divide(x=w2308, y=3) -> (x/y=w2311:dbl)
                        n1213 = To Word Integer(number=w2311) -> (16bit integer=w2310:i16)
                        n1214 = Replace Array Subset(array=w2312, new element=w2309, index (row)=w2310, index (col)=1) -> (w2307:string[][])
                      }
                      frame True {
                      }
                    }
                    n1215 = local write "Save1 Array"(w2300) -> ()
                  }
                  frame #10 {
                    n1216 = Search 1D Array(1D array=w2319, element="STS-Sat (V/decade):") -> (index of element=w2321:i32)  [unwired: 1 in]
                    n1217 = Equal?(x=w2321, y=-1) -> (x = y?=w2320:bool)
                    n1218 = local read "Save1 Array"() -> (w2318:string[][])
                    n1219 = case shown="False" w2320 {
                      tunnel: w2318 -> [w2329 w2333]
                      tunnel: w2321 -> [w2325 _]
                      tunnel: [w2324 w2333] -> w2317
                      frame False {
                        n1220 = local read "New: STS"() -> (w2331:dbl)
                        n1221 = Number To Fractional String(number=w2331) -> (F-format string=w2326:string)  [unwired: 3 in]
                        n1222 = Divide(x=w2325, y=3) -> (x/y=w2328:dbl)
                        n1223 = To Word Integer(number=w2328) -> (16bit integer=w2327:i16)
                        n1224 = Replace Array Subset(array=w2329, new element=w2326, index (row)=w2327, index (col)=1) -> (w2324:string[][])
                      }
                      frame True {
                      }
                    }
                    n1225 = local write "Save1 Array"(w2317) -> ()
                  }
                  frame #11 {
                    n1226 = Search 1D Array(1D array=w2336, element="Trap Density-VT (Traps/Vcm^2):") -> (index of element=w2338:i32)  [unwired: 1 in]
                    n1227 = Equal?(x=w2338, y=-1) -> (x = y?=w2337:bool)
                    n1228 = local read "Save1 Array"() -> (w2335:string[][])
                    n1229 = case shown="False" w2337 {
                      tunnel: w2335 -> [w2346 w2350]
                      tunnel: w2338 -> [w2342 _]
                      tunnel: [w2341 w2350] -> w2334
                      frame False {
                        n1230 = local read "New: Trap Density-VT"() -> (w2348:dbl)
                        n1231 = Number To Fractional String(number=w2348) -> (F-format string=w2343:string)  [unwired: 3 in]
                        n1232 = Divide(x=w2342, y=3) -> (x/y=w2345:dbl)
                        n1233 = To Word Integer(number=w2345) -> (16bit integer=w2344:i16)
                        n1234 = Replace Array Subset(array=w2346, new element=w2343, index (row)=w2344, index (col)=1) -> (w2341:string[][])
                      }
                      frame True {
                      }
                    }
                    n1235 = local write "Save1 Array"(w2334) -> ()
                  }
                  frame #12 {
                    n1236 = Search 1D Array(1D array=w2353, element="Trap Density-STS (Traps/Vcm^2):") -> (index of element=w2355:i32)  [unwired: 1 in]
                    n1237 = Equal?(x=w2355, y=-1) -> (x = y?=w2354:bool)
                    n1238 = local read "Save1 Array"() -> (w2352:string[][])
                    n1239 = case shown="False" w2354 {
                      tunnel: w2352 -> [w2363 w2367]
                      tunnel: w2355 -> [w2359 _]
                      tunnel: [w2358 w2367] -> w2351
                      frame False {
                        n1240 = local read "New: Trap Density-STS"() -> (w2365:dbl)
                        n1241 = Number To Fractional String(number=w2365) -> (F-format string=w2360:string)  [unwired: 3 in]
                        n1242 = Divide(x=w2359, y=3) -> (x/y=w2362:dbl)
                        n1243 = To Word Integer(number=w2362) -> (16bit integer=w2361:i16)
                        n1244 = Replace Array Subset(array=w2363, new element=w2360, index (row)=w2361, index (col)=1) -> (w2358:string[][])
                      }
                      frame True {
                      }
                    }
                    n1245 = local write "Save1 Array"(w2351) -> ()
                  }
                }
                n1246 = Concatenate Strings(w2143, "\\", w2141) -> (w2142:string)
                n1247 = String To Path(string=w2142) -> (path=w2119:path)
                "No Image 2" <- w2119
                n1248 = local write "Save1 Array"(w2116) -> ()
              }
              frame #1 {
                n1249 = Equal?(x=w2371, y=w2370) -> (x = y?=w2369:bool)
                n1250 = case shown="False" w2369 {
                  tunnel: w2371 -> [w2375 _]
                  tunnel: w2370 -> [w2374 _]
                  frame False {
                    n1251 = Move(source path=w2375, 9:TRUE, 10:w2374) -> ()  [unwired: 2 in, 3 out]
                  }
                  frame True {
                  }
                }
              }
              frame #2 {
                n1252 = local write "Data File"(w2377) -> ()
                n1253 = call-poly <vilib>:"Write To Spreadsheet File.vi"("2D data"=w2376, "file path (dialog if empty)"=w2377) -> ()  [unwired: 6 in, 1 out]
              }
              frame #3 {
                w2477 = 0
                # "Moves to next file and displays new image/data"
                n1254 = property on="Image Out" class="ImageControl"() -> (error out=w2439:errorcluster, "Image Center Position"=w2443:cluster{"X":u32, "Y":u32})  [unwired: 2 in, 1 out]
                n1255 = local read "Data File"() -> (w2482:path)
                n1256 = Strip Path(path=w2482) -> (stripped path=w2473:path, name=w2491:string)
                n1257 = Unbundle(w2443) -> ("X"=w2441:u32)  [unwired: 1 out]
                n1258 = local write "Data Folder"(w2473) -> ()
                n1259 = Bundle("X"=w2441, 0) -> (w2442:cluster{"X":u32, i32})  [unwired: 1 in]
                n1260 = property on="Image Out" class="ImageControl"(error in=w2439, "Image Center Position"=w2442) -> ()  [unwired: 1 in, 2 out]
                n1261 = List Folder(path=w2473) -> (filenames=w2487:string[])  [unwired: 3 in, 3 out]
                n1262 = Search 1D Array(1D array=w2487, element=w2491) -> (index of element=w2484:i32)  [unwired: 1 in]
                n1263 = Array Size(array=w2487) -> (size(s)=w2483:i32)
                n1264 = Decrement(x=w2483) -> (x-1=w2485:i32)
                n1265 = Equal?(x=w2484, y=w2485) -> (x = y?=w2486:bool)
                n1266 = local read "Folder Index"() -> (w2435:dbl)
                n1267 = case shown="False" w2486 {
                  tunnel: w2435 -> [w2616 _]
                  tunnel: [w2615 0] -> w2434
                  frame False {
                    n1268 = Increment(x=w2616) -> (x+1=w2615:dbl)
                  }
                  frame True {
                  }
                }
                n1269 = invoke on="Image Out" class="ImageControl" method="Clear ROI"() -> ()  [unwired: 3 in, 3 out]
                n1270 = local write "Folder Index"(w2434) -> ()
                n1271 = Path To String(path=w2473) -> (string=w2492:string)
                n1272 = Index Array(array=w2487, index=w2434) -> (element=w2488:string)
                n1273 = local write "Data Name:"(w2488) -> ()
                n1274 = Concatenate Strings(w2492, "\\", w2488) -> (w2490:string)
                n1275 = String To Path(string=w2490) -> (path=w2386:path)
                n1276 = call "Recorded Values.vi"("Path"=w2386) -> ("Recorded Char"=w2388:T5, "Recorded Prop"=w2389:T6, "Fabrication Prop"=w2387:T7)  [unwired: 8 in]
                n1277 = Unbundle By Name(w2388) -> ("Mobility-Sat"=w2401:dbl, "Moblitity-Lin"=w2402:dbl, "On/Off"=w2403:dbl, "Off Current"=w2404:dbl, "Vt-Sat"=w2380:dbl, "STS"=w2405:dbl, "Trap Density-VT"=w2406:dbl, "Trap Density-STS"=w2407:dbl)
                n1278 = Unbundle By Name(w2389) -> ("Date Recorded"=w2397:string, "Index"=w2398:string, "Length"=w2399:dbl, "Width"=w2400:dbl, "Sample Temp"=w2383:dbl)
                n1279 = Unbundle By Name(w2387) -> ("Date Created"=w2408:string, "Material"=w2390:string, "Solvent"=w2391:string, "Concentration"=w2392:dbl, "Method"=w2393:string, "Dielectric (nm)"=w2394:dbl, "Treatment"=w2395:string, "Comments"=w2396:string)
                n1280 = local write "Rec: Off I-Sat"(w2404) -> ()
                n1281 = local write "Rec: VT-Sat"(w2380) -> ()
                n1282 = local write "Date Created"(w2408) -> ()
                n1283 = local write "Rec: Material"(w2390) -> ()
                n1284 = local write "Rec: Solvent"(w2391) -> ()
                n1285 = local write "Rec: Concentration"(w2392) -> ()
                n1286 = local write "Rec: Method"(w2393) -> ()
                n1287 = local write "Rec: Dielectric (d)"(w2394) -> ()
                n1288 = local write "Surface Treatment:"(w2395) -> ()
                n1289 = local write "Comments"(w2396) -> ()
                n1290 = local write "Index"(w2398) -> ()
                n1291 = local write "Rec: Mobility-Sat"(w2401) -> ()
                n1292 = local write "Rec: Mobility-Lin"(w2402) -> ()
                n1293 = local write "Rec: On/Off"(w2403) -> ()
                n1294 = local write "Rec: STS"(w2405) -> ()
                n1295 = local write "Rec: Trap Density-VT"(w2406) -> ()
                n1296 = local write "Rec: Trap Density-STS"(w2407) -> ()
                n1297 = local write "Date Recorded"(w2397) -> ()
                n1298 = local write "Rec: Length"(w2399) -> ()
                n1299 = local write "Rec: Width"(w2400) -> ()
                n1300 = local write "Rec: Temp"(w2383) -> ()
                n1301 = Equal To 0?(x=w2383) -> (x = 0?=w2384:bool)
                n1302 = case shown="False" w2384 {
                  tunnel: [w2493 w2494] -> w2381
                  tunnel: w2383 -> [w2493 _]
                  frame False {
                  }
                  frame True {
                    n1303 = local read "Room Temp"() -> (w2494:dbl)
                  }
                }
                n1304 = local write "Data File"(w2386) -> ()
                n1305 = local read "NumPts 2"() -> (w2430:dbl)
                n1306 = local read "NumPts"() -> (w2419:dbl)
                n1307 = local read "NumPts"() -> (w2431:dbl)
                n1308 = call-poly <vilib>:"Read From Spreadsheet File.vi"("file path (dialog if empty)"=w2386) -> ("all rows"=w2479:string[][])  [unwired: 6 in, 4 out]
                n1309 = call "Mobility-Vt Calculator-File.vi"("NumPts"=w2431, "Path"=w2386) -> ("XY Graph-Sat"=w2432:cluster{dbl[], dbl[]}[], "XY Graph-Lin"=w2414:cluster{dbl[], dbl[]}[], "Output"=w2433:T8, "Index-Sat"=w2411:dbl, "Index-Lin"=w2418:dbl)  [unwired: 4 in, 1 out]
                n1310 = Decimate 1D Array(w2414) -> (w2426:cluster{dbl[], dbl[]}[])  [unwired: 1 out]
                n1311 = Array To Cluster(array=w2426) -> (cluster=w2424:T9)
                n1312 = Unbundle(w2424) -> ("[0]"=w2425:cluster{dbl[], dbl[]})  [unwired: 8 out]
                n1313 = local write "XY Graph-Lin"(w2414) -> ()
                n1314 = Unbundle(w2425) -> (w2423:dbl[], w2422:dbl[])
                n1315 = Array Subset(array=w2422, index=w2418, length=w2419) -> (w2420:dbl[])
                n1316 = Array Subset(array=w2423, index=w2418, length=w2419) -> (w2421:dbl[])
                n1317 = call "STS Calculator-File.vi"("NumPts"=w2430, "Path"=w2386) -> ("STS Index-Sat"=w2429:dbl, "XY Graph-Sat"=w2428:cluster{dbl[], dbl[]}[], "Ouput"=w2427:cluster{"STS-Sat":dbl, "STS-Lin":dbl})  [unwired: 5 in, 2 out]
                n1318 = local read "New: Dielectric"() -> (w2413:dbl)
                n1319 = local write "Lin Id-Used"(w2420) -> ()
                n1320 = local write "Lin-Vg Array-Used"(w2421) -> ()
                n1321 = local write "MobVi Index"(w2411) -> ()
                n1322 = local write "Slide"(w2411) -> ()
                n1323 = local write "XY Graph"(w2432) -> ()
                n1324 = local write "Index 2"(w2429) -> ()
                n1325 = local write "XY Graph 2"(w2428) -> ()
                n1326 = Unbundle By Name(w2433) -> ("Mobility-Sat"=w2417:dbl, "Vt-Sat"=w2378:dbl, "Mobility-Lin"=w2416:dbl, "Mobility-Lin"=w2415:dbl, "Off I-Sat"=w2409:dbl, "On/Off I-Sat"=w2379:dbl)
                n1327 = Array Size(array=w2479) -> (size(s)=w2478:i32[])
                n1328 = local write "New: Temp"(w2381) -> ()
                n1329 = Unbundle By Name(w2427) -> ("STS-Sat"=w2412:dbl)
                n1330 = call "Trap Density_STS.vi"("Temp (T) [K]"=w2381, "S.T.S. (S)"=w2412, "Dielectric"=w2413) -> ("Trap Density (N)"=w2385:dbl)  [unwired: 8 in]
                n1331 = local write "Calc: Mobility-Lin"(w2416) -> ()
                n1332 = local write "Calc: Mobility-Sat"(w2417) -> ()
                n1333 = local write "Calc: Off I-Sat"(w2409) -> ()
                n1334 = local write "Calc: VT-Sat"(w2378) -> ()
                n1335 = local write "New: VT-Lin"(w2415) -> ()
                n1336 = local write "New: Trap Density-STS"(w2385) -> ()
                n1337 = local write "Calc: Trap Density-STS"(w2385) -> ()
                n1338 = local read "Image Folder"() -> (w2467:path)
                n1339 = local read "New: Dielectric"() -> (w2410:dbl)
                n1340 = Decimate 1D Array(w2432) -> (w2462:cluster{dbl[], dbl[]}[])  [unwired: 1 out]
                n1341 = Decimate 1D Array(w2428) -> (w2452:cluster{dbl[], dbl[]}[])  [unwired: 1 out]
                n1342 = Index Array(array=w2478, index=w2477) -> (element=w2458:i32)
                n1343 = Array Subset(array=w2479, index (row)=w2477, index (col)=w2477, length (col)=3) -> (w2480:string[][])  [unwired: 1 in]
                n1344 = local write "Calc: STS"(w2412) -> ()
                n1345 = local write "New: VT-Sat"(w2378) -> ()
                n1346 = local write "New: Mobility-Sat"(w2417) -> ()
                n1347 = local write "Calc: On/Off"(w2379) -> ()
                n1348 = local write "New: Mobility-Lin"(w2416) -> ()
                n1349 = List Folder(path=w2467) -> (filenames=w2472:string[])  [unwired: 3 in, 3 out]
                n1350 = local write "New: VT-Lin"(w2415) -> ()
                n1351 = Array To Cluster(array=w2462) -> (cluster=w2464:T9)
                n1352 = Array To Cluster(array=w2452) -> (cluster=w2450:T9)
                n1353 = Reshape Array(w2480, w2458) -> (w2465:string[])
                n1354 = Subtract(x=w2458, y=20) -> (x-y=w2457:i32)
                n1355 = local write "New: STS"(w2412) -> ()
                n1356 = property on="Slide" class="Slide (strict)"("Scale.Maximum"=w2457) -> ()  [unwired: 2 in, 2 out]
                n1357 = call "Trap Density_VT.vi"("VT"=w2378, "Dielectric"=w2410) -> ("Trap Density-VT"=w2382:dbl)
                n1358 = Unbundle(w2464) -> ("[0]"=w2463:cluster{dbl[], dbl[]})  [unwired: 8 out]
                n1359 = Unbundle(w2450) -> ("[0]"=w2451:cluster{dbl[], dbl[]})  [unwired: 8 out]
                n1360 = Search 1D Array(1D array=w2465, element="Index:") -> (index of element=w2474:i32)  [unwired: 1 in]
                n1361 = local write "New: Trap Density-VT"(w2382) -> ()
                n1362 = local write "Calc: Trap Density-VT"(w2382) -> ()
                n1363 = Unbundle(w2463) -> (w2454:dbl[], w2453:dbl[])
                n1364 = Unbundle(w2451) -> (w2449:dbl[], w2448:dbl[])
                n1365 = Increment(x=w2474) -> (x+1=w2475:i32)
                n1366 = Array Subset(array=w2454, index=w2411, length=w2431) -> (w2461:dbl[])
                n1367 = Array Subset(array=w2453, index=w2411, length=w2431) -> (w2460:dbl[])
                n1368 = Array Subset(array=w2449, index=w2429, length=w2430) -> (w2456:dbl[])
                n1369 = Array Subset(array=w2448, index=w2429, length=w2430) -> (w2455:dbl[])
                n1370 = Index Array(array=w2465, index=w2475) -> (element=w2470:string)
                n1371 = local write "Vg Array-Log-Used"(w2455) -> ()
                n1372 = local write "Sat Id-Log-Used"(w2456) -> ()
                n1373 = local write "Sat Id-Used"(w2460) -> ()
                n1374 = local write "Index"(w2470) -> ()
                n1375 = local write "Sat Vg Array-Used"(w2461) -> ()
                n1376 = while {
                  tunnel: w2472 -> [w2502]
                  tunnel: w2470 -> [w2500]
                  tunnel: [w2499] -> _
                  tunnel: [w2499] -> w2471
                  tunnel: w2458 -> [w2498]
                  i -> [w2499]
                  stop <- w2495 stop-if-true
                  n1377 = Index Array(array=w2502, index=w2499) -> (element=w2503:string)
                  n1378 = xnode "Match Regular Expression"("input string"=w2503, "regular expression"=w2500) -> ("whole match"=w2501:string)  [unwired: 4 in, 4 out]
                  n1379 = Equal?(x=w2501, y=w2500) -> (x = y?=w2497:bool)
                  n1380 = Equal?(x=w2498, y=w2499) -> (x = y?=w2496:bool)
                  n1381 = Or(x=w2497, y=w2496) -> (x .or. y?=w2495:bool)
                }
                n1382 = Path To String(path=w2467) -> (string=w2469:string)
                n1383 = Index Array(array=w2472, index=w2471) -> (element=w2446:string)
                n1384 = local write "Image Name"(w2446) -> ()
                n1385 = Empty String/Path?(string/path=w2446) -> (empty?=w2447:bool)
                n1386 = Concatenate Strings(w2469, "\\", w2446) -> (w2468:string)
                n1387 = String To Path(string=w2468) -> (path=w2445:path)
                n1388 = local read "No Image"() -> (w2444:path)
                n1389 = Select(t=w2444, s=w2447, f=w2445) -> (s? t:f=w2438:path)
                n1390 = local write "Image File"(w2438) -> ()
                n1391 = local read "Image Out"() -> (w2436:T2)
                n1392 = call "IMAQ ReadFile"("File Path"=w2438, "Image"=w2436) -> ("Image Out"=w2437:T2)  [unwired: 5 in, 4 out]
                n1393 = local write "Image Out"(w2437) -> ()
                n1394 = local write "Image Out 2"(w2437) -> ()
              }
              frame #4 {
                # "Output ROI data"
                n1395 = local read "Image Folder"() -> (w2618:path)
                n1396 = Build Path(base path=w2618, name or relative path="ROI") -> (appended path=w2620:path)
                n1397 = local read "Index"() -> (w2619:string)
                n1398 = Build Path(base path=w2620, name or relative path=w2619) -> (appended path=w2625:path)
                n1399 = invoke on="Image Out" class="ImageControl" method="Clear ROI"() -> (error out=w2624:errorcluster)  [unwired: 3 in, 2 out]
                n1400 = call <vilib>:"Check if File or Folder Exists.vi"("error in (no error)"=w2624, "path"=w2625) -> ("file or folder exists?"=w2622:bool, "dup path"=w2623:path)  [unwired: 7 in, 1 out]
                n1401 = case shown="True" w2622 {
                  tunnel: w2623 -> [_ w2626]
                  frame False {
                  }
                  frame True {
                    n1402 = Read from Text File(file (use dialog)=w2626) -> (text=w2630:string)  [unwired: 3 in, 3 out]
                    n1403 = property on="Image Out" class="ImageControl"() -> ("ROI"=w2627:T10)  [unwired: 2 in, 2 out]
                    n1404 = Unflatten From String(type=w2627, binary string=w2630) -> (value=w2628:T10, error out=w2629:errorcluster)  [unwired: 3 in, 1 out]
                    n1405 = property on="Image Out" class="ImageControl"(error in=w2629, "ROI"=w2628) -> ()  [unwired: 1 in, 2 out]
                  }
                }
              }
            }
            n1406 = flat-sequence {
              tunnel: [w2073] -> w2060
              tunnel: w2060 -> [w2087]
              frame #0 {
                # "Makes Empty File for Transformer Data"
                n1407 = local read "Data Folder"() -> (w2062:path)
                n1408 = Build Path(base path=w2062, name or relative path="Stats") -> (appended path=w2064:path)
                n1409 = call <vilib>:"Check if File or Folder Exists.vi"("path"=w2064) -> ("file or folder exists?"=w2065:bool, "dup path"=w2066:path)  [unwired: 8 in, 1 out]
                n1410 = case shown="False" w2065 {
                  tunnel: [w2070 w2072] -> w2067
                  tunnel: w2066 -> [w2071 w2072]
                  frame False {
                    n1411 = Create Folder(path (use dialog)=w2071) -> (created path=w2070:path)  [unwired: 2 in, 2 out]
                  }
                  frame True {
                  }
                }
                n1412 = Build Path(base path=w2067, name or relative path="Tranformer Data.txt") -> (appended path=w2069:path)
                n1413 = call-poly <vilib>:"Write To Spreadsheet File.vi"("append to file? (new file:F)"=TRUE, "file path (dialog if empty)"=w2069) -> ()  [unwired: 6 in, 1 out]
              }
              frame #1 {
                # "Adds Headers if they don't exist"
                n1414 = Concatenate Strings("Stats\\", "Tranformer Data.txt") -> (w2080:string)
                n1415 = local read "Data Folder"() -> (w2079:path)
                n1416 = Build Path(base path=w2079, name or relative path=w2080) -> (appended path=w2073:path)
                n1417 = call-poly <vilib>:"Read From Spreadsheet File.vi"("file path (dialog if empty)"=w2073) -> ("first row"=w2078:string[])  [unwired: 6 in, 4 out]
                n1418 = Search 1D Array(1D array=w2078, element="DeviceID") -> (index of element=w2076:i32)  [unwired: 1 in]
                n1419 = Equal?(x=w2076, y=0) -> (x = y?=w2074:bool)
                n1420 = case shown="False" w2074 {
                  tunnel: w2073 -> [w2084 _]
                  frame False {
                    n1421 = local read "Transformer \nHeaders"() -> (w2083:string[])
                    n1422 = call-poly <vilib>:"Write To Spreadsheet File.vi"("1D data"=w2083, "file path (dialog if empty)"=w2084) -> ()  [unwired: 6 in, 1 out]
                  }
                  frame True {
                  }
                }
              }
              frame #2 {
                # "Adds current device if it doesn't exist"
                n1423 = local read "Current \nRecord"() -> (w2090:string[])
                n1424 = Index Array(array=w2090, index=0) -> (element=w2089:string)
                n1425 = Concatenate Strings("Stats\\", "Tranformer Data.txt") -> (w2093:string)
                n1426 = local read "Data Folder"() -> (w2092:path)
                n1427 = local write "Current Device ID"(w2089) -> ()
                n1428 = local read "Current Device ID"() -> (w2099:string)
                n1429 = Build Path(base path=w2092, name or relative path=w2093) -> (appended path=w2091:path)
                n1430 = call-poly <vilib>:"Read From Spreadsheet File.vi"("file path (dialog if empty)"=w2091) -> ("all rows"=w2086:string[][])  [unwired: 6 in, 4 out]
                n1431 = Index Array(array=w2086, index (col)=0) -> (element=w2097:string[])  [unwired: 1 in]
                n1432 = Search 1D Array(1D array=w2097, element=w2099) -> (index of element=w2085:i32)  [unwired: 1 in]
                n1433 = Equal?(x=w2085, y=-1) -> (x = y?=w2088:bool)
                n1434 = case shown="False" w2088 {
                  tunnel: w2087 -> [w2101 w2114]
                  tunnel: w2085 -> [w2106 _]
                  tunnel: w2086 -> [w2107 _]
                  frame False {
                    n1435 = local read "Current \nRecord"() -> (w2105:string[])
                    n1436 = Replace Array Subset(array=w2107, new element=w2105, index (row)=w2106) -> (w2102:string[][])  [unwired: 1 in]
                    n1437 = flat-sequence {
                      tunnel: [w2108] -> _
                      tunnel: [w2109] -> _
                      tunnel: [w2109] -> w2104
                      tunnel: [w2108] -> w2103
                      tunnel: w2102 -> [w2109]
                      tunnel: w2101 -> [w2108]
                      tunnel: w2104 -> [w2111]
                      tunnel: w2103 -> [w2110]
                      frame #0 {
                        n1438 = Delete(path (use dialog)=w2108) -> ()  [unwired: 4 in, 3 out]
                      }
                      frame #1 {
                        n1439 = call-poly <vilib>:"Write To Spreadsheet File.vi"("append to file? (new file:F)"=TRUE, "2D data"=w2111, "file path (dialog if empty)"=w2110) -> ()  [unwired: 5 in, 1 out]
                      }
                    }
                  }
                  frame True {
                    n1440 = local read "Current \nRecord"() -> (w2113:string[])
                    n1441 = call-poly <vilib>:"Write To Spreadsheet File.vi"("append to file? (new file:F)"=TRUE, "1D data"=w2113, "file path (dialog if empty)"=w2114) -> ()  [unwired: 5 in, 1 out]
                  }
                }
              }
            }
          }
          event "Export": Mouse Down {
            n1442 = event-data() -> ()  [unwired: 1 in, 7 out]
            n1443 = local read "Data Folder"() -> (w2635:path)
            n1444 = Build Path(base path=w2635, name or relative path="Stats") -> (appended path=w2636:path)
            n1445 = call <vilib>:"Check if File or Folder Exists.vi"("path"=w2636) -> ("file or folder exists?"=w2652:bool, "dup path"=w2651:path)  [unwired: 8 in, 1 out]
            n1446 = local read "Project"() -> (w2648:path)
            n1447 = call <userlib>:"OA_ConnectToOrigin.vi"() -> ("error out"=w2649:errorcluster, "Origin.IOApplication"=w2650:refnum<k7>)  [unwired: 8 in]
            n1448 = case shown="False" w2652 {
              tunnel: w2651 -> [w2769 w2770]
              tunnel: [w2768 w2770] -> w2634
              frame False {
                n1449 = Create Folder(path (use dialog)=w2769) -> (created path=w2768:path)  [unwired: 2 in, 2 out]
              }
              frame True {
              }
            }
            n1450 = call <userlib>:"OA_Load.vi"("error in (no error)"=w2649, "Path"=w2648, "Origin.IOApplication"=w2650) -> ("error out"=w2646:errorcluster, "Origin.IOApplication"=w2647:refnum<k7>)  [unwired: 1 out]
            n1451 = call <userlib>:"OAExecute.vi"("script"="document -m 3;", "Error IO"=w2646, "Origin.IOApplication"=w2647) -> ("Error IO Out"=w2644:errorcluster, "Origin.IOApplication"=w2645:refnum<k7>)  [unwired: 1 in, 1 out]
            n1452 = call "File Dialog"("start path"=w2636) -> ("selected path"=w2639:path)  [unwired: 11 in, 3 out]
            n1453 = local read "Independant Variable"() -> (w2631:string)
            n1454 = stacked-sequence {
              tunnel: w2635 -> [w2665 w2669 w2683 w2697 w2711 w2725 w2740 w2755]
              tunnel: w2634 -> [w2664 w2670 w2684 w2698 w2712 w2726 w2739 w2756]
              tunnel: w2645 -> [w2661 w2672 w2686 w2700 w2714 w2728 w2742 w2758]
              tunnel: w2644 -> [w2663 w2671 w2685 w2699 w2713 w2727 w2741 w2757]
              tunnel: [_ _ _ _ _ _ _ w2753] -> w2633
              tunnel: [_ _ _ _ _ _ _ w2754] -> w2632
              tunnel: w2631 -> [w2654 w2668 w2682 w2696 w2710 w2724 w2738 w2752]
              frame #0 {
                n1455 = call "Param_Analysis_7_24b_JW.vi"("Independant Variable"=w2654, "error in (no error)"=w2663, "Data Folder"=w2665, "Parameter String"="Mobility-Sat (cm^2/Vs):", "Parameter Name"="Mobility-Sat", "Stats Folder"=w2664) -> ("error out"=w2657:errorcluster, "Output Array"=w2655:string[][])  [unwired: 3 in, 1 out]
                n1456 = call "Origin_Export_7_24a_JW.vi"("Analysis Array"=w2655, "error in (no error)"=w2657, "Parameter Worksheet Name"="[MOBSvsLTable]Mobilities", "Parameter Folder Script"="pe_cd \"Mobility-Sat\";", "Origin.IOApplication"=w2661) -> ("error out"=w2656:errorcluster, "reference out"=w2658:refnum<k7>)  [unwired: 4 in, 1 out]
                n1457 = call <userlib>:"OAExecute.vi"("script"="window -a MOBSvsLTable;\nwindow -s TV;", "Error IO"=w2656, "Origin.IOApplication"=w2658) -> ()  [unwired: 1 in, 3 out]
              }
              frame #1 {
                n1458 = call "Param_Analysis_7_24b_JW.vi"("Independant Variable"=w2668, "error in (no error)"=w2671, "Data Folder"=w2669, "Parameter String"="Mobility-Lin (cm^2/Vs):", "Parameter Name"="Mobility-Lin", "Stats Folder"=w2670) -> ("error out"=w2674:errorcluster, "Output Array"=w2676:string[][])  [unwired: 3 in, 1 out]
                n1459 = call "Origin_Export_7_24a_JW.vi"("Analysis Array"=w2676, "error in (no error)"=w2674, "Parameter Worksheet Name"="[MOBLvsLTable]Mobilities", "Parameter Folder Script"="pe_cd \"Mobility-Lin\";", "Origin.IOApplication"=w2672) -> ("error out"=w2673:errorcluster, "reference out"=w2675:refnum<k7>)  [unwired: 4 in, 1 out]
                n1460 = call <userlib>:"OAExecute.vi"("script"="window -a MOBLvsLTable;\nwindow -s TV;", "Error IO"=w2673, "Origin.IOApplication"=w2675) -> ()  [unwired: 1 in, 3 out]
              }
              frame #2 {
                n1461 = call "Param_Analysis_7_24b_JW.vi"("Independant Variable"=w2682, "error in (no error)"=w2685, "Data Folder"=w2683, "Parameter String"="Off I-Sat (A):", "Parameter Name"="Off I-Sat", "Stats Folder"=w2684) -> ("error out"=w2689:errorcluster, "Output Array"=w2687:string[][])  [unwired: 3 in, 1 out]
                n1462 = call "Origin_Export_7_24a_JW.vi"("Analysis Array"=w2687, "error in (no error)"=w2689, "Parameter Worksheet Name"="[OffItable]OffCurrents", "Parameter Folder Script"="pe_cd \"Off I-Sat\";", "Origin.IOApplication"=w2686) -> ("error out"=w2688:errorcluster, "reference out"=w2690:refnum<k7>)  [unwired: 4 in, 1 out]
                n1463 = call <userlib>:"OAExecute.vi"("script"="window -a OffItable;\nwindow -s TV;", "Error IO"=w2688, "Origin.IOApplication"=w2690) -> ()  [unwired: 1 in, 3 out]
              }
              frame #3 {
                n1464 = call "Param_Analysis_7_24b_JW.vi"("Independant Variable"=w2696, "error in (no error)"=w2699, "Data Folder"=w2697, "Parameter String"="On/Off I-Sat:", "Parameter Name"="OnOff Ratio", "Stats Folder"=w2698) -> ("error out"=w2703:errorcluster, "Output Array"=w2701:string[][])  [unwired: 3 in, 1 out]
                n1465 = call "Origin_Export_7_24a_JW.vi"("Analysis Array"=w2701, "error in (no error)"=w2703, "Parameter Worksheet Name"="[OnOffTable]On/Off Ratios", "Parameter Folder Script"="pe_cd \"On Off Ratio\";", "Origin.IOApplication"=w2700) -> ("error out"=w2702:errorcluster, "reference out"=w2704:refnum<k7>)  [unwired: 4 in, 1 out]
                n1466 = call <userlib>:"OAExecute.vi"("script"="window -a OnOffTable;\nwindow -s TV;", "Error IO"=w2702, "Origin.IOApplication"=w2704) -> ()  [unwired: 1 in, 3 out]
              }
              frame #4 {
                n1467 = call "Param_Analysis_7_24b_JW.vi"("Independant Variable"=w2710, "error in (no error)"=w2713, "Data Folder"=w2711, "Parameter String"="STS-Sat (V/decade):", "Parameter Name"="STS-Sat", "Stats Folder"=w2712) -> ("error out"=w2717:errorcluster, "Output Array"=w2715:string[][])  [unwired: 3 in, 1 out]
                n1468 = call "Origin_Export_7_24a_JW.vi"("Analysis Array"=w2715, "error in (no error)"=w2717, "Parameter Worksheet Name"="[STable]Threshold Swing", "Parameter Folder Script"="pe_cd \"STS-Sat\";", "Origin.IOApplication"=w2714) -> ("error out"=w2716:errorcluster, "reference out"=w2718:refnum<k7>)  [unwired: 4 in, 1 out]
                n1469 = call <userlib>:"OAExecute.vi"("script"="window -a STable;\nwindow -s TV;", "Error IO"=w2716, "Origin.IOApplication"=w2718) -> ()  [unwired: 1 in, 3 out]
              }
              frame #5 {
                n1470 = call "Param_Analysis_7_24b_JW.vi"("Independant Variable"=w2724, "error in (no error)"=w2727, "Data Folder"=w2725, "Parameter String"="Trap Density-STS (Traps/Vcm^2):", "Parameter Name"="Trap Density-STS", "Stats Folder"=w2726) -> ("error out"=w2731:errorcluster, "Output Array"=w2729:string[][])  [unwired: 3 in, 1 out]
                n1471 = call "Origin_Export_7_24a_JW.vi"("Analysis Array"=w2729, "error in (no error)"=w2731, "Parameter Worksheet Name"="[NSTSTable]Trap Densities", "Parameter Folder Script"="pe_cd \"Trap Density-STS\";", "Origin.IOApplication"=w2728) -> ("error out"=w2730:errorcluster, "reference out"=w2732:refnum<k7>)  [unwired: 4 in, 1 out]
                n1472 = call <userlib>:"OAExecute.vi"("script"="window -a NSTSTable;\nwindow -s TV;", "Error IO"=w2730, "Origin.IOApplication"=w2732) -> ()  [unwired: 1 in, 3 out]
              }
              frame #6 {
                n1473 = call "Param_Analysis_7_24b_JW.vi"("Independant Variable"=w2738, "error in (no error)"=w2741, "Data Folder"=w2740, "Parameter String"="Trap Density-Vt (Traps/Vcm^2):", "Parameter Name"="Trap Density-Vt", "Stats Folder"=w2739) -> ("error out"=w2745:errorcluster, "Output Array"=w2743:string[][])  [unwired: 3 in, 1 out]
                n1474 = call "Origin_Export_7_24a_JW.vi"("Analysis Array"=w2743, "error in (no error)"=w2745, "Parameter Worksheet Name"="[NVTTable]Trap Densities", "Parameter Folder Script"="pe_cd \"Trap Density-Vt\";", "Origin.IOApplication"=w2742) -> ("error out"=w2744:errorcluster, "reference out"=w2746:refnum<k7>)  [unwired: 4 in, 1 out]
                n1475 = call <userlib>:"OAExecute.vi"("script"="window -a NVTTable;\nwindow -s TV;", "Error IO"=w2744, "Origin.IOApplication"=w2746) -> ()  [unwired: 1 in, 3 out]
              }
              frame #7 {
                n1476 = call "Param_Analysis_7_24b_JW.vi"("Independant Variable"=w2752, "error in (no error)"=w2757, "Data Folder"=w2755, "Parameter String"="Vt-Sat (V):", "Parameter Name"="Vt-Sat", "Stats Folder"=w2756) -> ("error out"=w2761:errorcluster, "Output Array"=w2759:string[][])  [unwired: 3 in, 1 out]
                n1477 = call "Origin_Export_7_24a_JW.vi"("Analysis Array"=w2759, "error in (no error)"=w2761, "Parameter Worksheet Name"="[VtTable]Threshold Voltages", "Parameter Folder Script"="pe_cd \"Vt-Sat\";", "Origin.IOApplication"=w2758) -> ("error out"=w2760:errorcluster, "reference out"=w2762:refnum<k7>)  [unwired: 4 in, 1 out]
                n1478 = call <userlib>:"OAExecute.vi"("script"="window -a VtTable;\nwindow -s TV;", "Error IO"=w2760, "Origin.IOApplication"=w2762) -> ("Error IO Out"=w2753:errorcluster, "Origin.IOApplication"=w2754:refnum<k7>)  [unwired: 1 in, 1 out]
              }
            }
            n1479 = Path To String(path=w2639) -> (string=w2638:string)
            n1480 = call <userlib>:"OAExecute.vi"("script"="pe_cd /; ", "Error IO"=w2633, "Origin.IOApplication"=w2632) -> ("Error IO Out"=w2640:errorcluster, "Origin.IOApplication"=w2641:refnum<k7>)  [unwired: 1 in, 1 out]
            n1481 = call <userlib>:"OASaveProject.vi"("path"=w2638, "Error IO"=w2640, "Origin.IOApplication"=w2641) -> ()  [unwired: 3 out]
          }
          event "Blank Button": Mouse Down {
            n1482 = event-data() -> ()  [unwired: 1 in, 7 out]
            n1483 = local read "Data File"() -> (w2778:path)
            n1484 = Strip Path(path=w2778) -> (stripped path=w2774:path, name=w2776:string)
            n1485 = Path To String(path=w2774) -> (string=w2773:string)
            n1486 = Concatenate Strings(w2773, "\\", "X_", w2776) -> (w2772:string)
            n1487 = String To Path(string=w2772) -> (path=w2771:path)
            n1488 = Move(source path=w2778, 10:w2771) -> ()  [unwired: 3 in, 3 out]
            n1489 = local write "Data File"(w2771) -> ()
          }
          event "Cancel Button": Mouse Down {
            (unwired) 6
            n1490 = event-data() -> ()  [unwired: 1 in, 7 out]
            n1491 = call "Simulate_Keyboard.vi"("Action"=2, "Virtual Key"=162) -> ()  [unwired: 7 in, 1 out]
          }
        }
        n1492 = Multiply(x=w523, y=10) -> (x*y=w525:sgl)
        n1493 = case shown="\"0\"" w564 {
          tunnel: w538 -> [w617 w623 w627 w629 w633 w635 w637 w639 w641 w643 w645 w647 w649 w651 w653 w655 w657 w659 w661 w663 w665 w667 w669 w671 w673 w675 w677 w679 w681 w683 w685 w687 w689 w691 w693 w695 w697 w699 w701 w703 w705 w707 w709 w711 w713 w715 w717 w719 w721 w723 w725 w727 w729 w731 w733 w735 w737 w739 w741 w743 w745 w747 w749 w751 w753 w755 w757 w759 w761 w763 w765 w767 w769 w771 w773 w775 w777 w779 w781 w783 w785 w787 w789 w791 w793 w795 w797 w799 w801 w803 w805 w807 w809 w811 w813 w815 w817 w819 w821 w823 w825 w827 w829 w831 w833]
          tunnel: [w617 w622 w626 w629 w633 w635 w637 w639 w641 w643 w645 w647 w649 w651 w653 w655 w657 w659 w661 w663 w665 w667 w669 w671 w673 w675 w677 w679 w681 w683 w685 w687 w689 w691 w693 w695 w697 w699 w701 w703 w705 w707 w709 w711 w713 w715 w717 w719 w721 w723 w725 w727 w729 w731 w733 w735 w737 w739 w741 w743 w745 w747 w749 w751 w753 w755 w757 w759 w761 w763 w765 w767 w769 w771 w773 w775 w777 w779 w781 w783 w785 w787 w789 w791 w793 w795 w797 w799 w801 w803 w805 w807 w809 w811 w813 w815 w817 w819 w821 w823 w825 w827 w829 w831 w833] -> w563
          tunnel: w539 -> [w619 w621 w625 w631 w632 w634 w636 w638 w640 w642 w644 w646 w648 w650 w652 w654 w656 w658 w660 w662 w664 w666 w668 w670 w672 w674 w676 w678 w680 w682 w684 w686 w688 w690 w692 w694 w696 w698 w700 w702 w704 w706 w708 w710 w712 w714 w716 w718 w720 w722 w724 w726 w728 w730 w732 w734 w736 w738 w740 w742 w744 w746 w748 w750 w752 w754 w756 w758 w760 w762 w764 w766 w768 w770 w772 w774 w776 w778 w780 w782 w784 w786 w788 w790 w792 w794 w796 w798 w800 w802 w804 w806 w808 w810 w812 w814 w816 w818 w820 w822 w824 w826 w828 w830 w832]
          tunnel: [w618 w621 w625 w630 w632 w634 w636 w638 w640 w642 w644 w646 w648 w650 w652 w654 w656 w658 w660 w662 w664 w666 w668 w670 w672 w674 w676 w678 w680 w682 w684 w686 w688 w690 w692 w694 w696 w698 w700 w702 w704 w706 w708 w710 w712 w714 w716 w718 w720 w722 w724 w726 w728 w730 w732 w734 w736 w738 w740 w742 w744 w746 w748 w750 w752 w754 w756 w758 w760 w762 w764 w766 w768 w770 w772 w774 w776 w778 w780 w782 w784 w786 w788 w790 w792 w794 w796 w798 w800 w802 w804 w806 w808 w810 w812 w814 w816 w818 w820 w822 w824 w826 w828 w830 w832] -> w562
          tunnel: w525 -> [w616 w620 w624 w628 _ _ _ _ _ _ _ _ _ _ _ _ _ _ _ _ _ _ _ _ _ _ _ _ _ _ _ _ _ _ _ _ _ _ _ _ _ _ _ _ _ _ _ _ _ _ _ _ _ _ _ _ _ _ _ _ _ _ _ _ _ _ _ _ _ _ _ _ _ _ _ _ _ _ _ _ _ _ _ _ _ _ _ _ _ _ _ _ _ _ _ _ _ _ _ _ _ _ _ _ _]
          frame "DOWN" {
            n1494 = Add(x=w619, y=w616) -> (x+y=w618:sgl)
          }
          frame "LEFT" {
            n1495 = Subtract(x=w623, y=w620) -> (x-y=w622:sgl)
          }
          frame "RIGHT" {
            n1496 = Add(x=w627, y=w624) -> (x+y=w626:sgl)
          }
          frame "UP" {
            n1497 = Subtract(x=w631, y=w628) -> (x-y=w630:sgl)
          }
          frame "ENTER (num pad)" {
          }
          frame "' (quote)" {
          }
          frame "END" {
          }
          frame "EQUALS" {
          }
          frame "ESCAPE" {
          }
          frame "GRAVE (`)" {
          }
          frame "HOME" {
          }
          frame "INSERT" {
          }
          frame "LBRACKET" {
          }
          frame "LCONTROL" {
          }
          frame "L ALT" {
          }
          frame "LSHIFT" {
          }
          frame "LWIN" {
          }
          frame "MINUS" {
          }
          frame "MULTIPLY" {
          }
          frame "NEXT" {
          }
          frame "NUMLOCK" {
          }
          frame "NUMPAD_0" {
          }
          frame "NUMPAD_1" {
          }
          frame "NUMPAD_2" {
          }
          frame "NUMPAD_3" {
          }
          frame "NUMPAD_4" {
          }
          frame "NUMPAD_5" {
          }
          frame "NUMPAD_6" {
          }
          frame "NUMPAD_7" {
          }
          frame "NUMPAD_8" {
          }
          frame "NUMPAD_9" {
          }
          frame "PAUSE" {
          }
          frame "PERIOD" {
          }
          frame "PRIOR (PG UP)" {
          }
          frame "RBRACKET" {
          }
          frame "RCONTROL" {
          }
          frame "RETURN" {
          }
          frame "R ALT" {
          }
          frame "RSHIFT" {
          }
          frame "RWIN" {
          }
          frame "SCROLL" {
          }
          frame "SEMICOLON" {
          }
          frame "SLASH" {
          }
          frame "SPACE" {
          }
          frame "SUBTRACT" {
          }
          frame "TAB" {
          }
          frame "DIVIDE" {
          }
          frame "DELETE" {
          }
          frame "DECIMAL" {
          }
          frame "COMMA" {
          }
          frame "CAPITAL" {
          }
          frame "BACKSLASH" {
          }
          frame "BACK" {
          }
          frame "ADD" {
          }
          frame "F15" {
          }
          frame "F14" {
          }
          frame "F13" {
          }
          frame "F12" {
          }
          frame "F11" {
          }
          frame "F10" {
          }
          frame "F9" {
          }
          frame "F8" {
          }
          frame "F7" {
          }
          frame "F6" {
          }
          frame "F5" {
          }
          frame "F4" {
          }
          frame "F3" {
          }
          frame "F2" {
          }
          frame "F1" {
          }
          frame "Z" {
          }
          frame "Y" {
          }
          frame "X" {
          }
          frame "W" {
          }
          frame "V" {
          }
          frame "U" {
          }
          frame "T" {
          }
          frame "S" {
          }
          frame "R" {
          }
          frame "Q" {
          }
          frame "P" {
          }
          frame "O" {
          }
          frame "N" {
          }
          frame "M" {
          }
          frame "L" {
          }
          frame "K" {
          }
          frame "J" {
          }
          frame "I" {
          }
          frame "H" {
          }
          frame "G" {
          }
          frame "F" {
          }
          frame "E" {
          }
          frame "D" {
          }
          frame "C" {
          }
          frame "B" {
          }
          frame "A" {
          }
          frame "9" {
          }
          frame "8" {
          }
          frame "7" {
          }
          frame "6" {
          }
          frame "5" {
          }
          frame "4" {
          }
          frame "3" {
          }
          frame "2" {
          }
          frame "1" {
          }
          frame "0" {
          }
        }
        n1498 = Bundle(w541, w540, w555, w554, 0.0) -> (w553:cluster{dbl, dbl, dbl, dbl, dbl})  [unwired: 1 in]
        n1499 = Bundle("X"=w563, "Y"=w562) -> (w557:cluster{"X":sgl, "Y":sgl})  [unwired: 1 in]
        n1500 = Divide(x=20, y=w524) -> (x/y=w527:sgl)
        n1501 = property on="Image Out" class="ImageControl"("Image Center Position"=w557) -> ()  [unwired: 2 in, 2 out]
        n1502 = call "IMAQ Convert Rectangle to ROI (Polygon)"("Rectangle"=w553) -> ("ROI Descriptor"=w551:T3)  [unwired: 7 in, 2 out]
        n1503 = Bundle("Application Font", w527, w531, w531, w531, w531, w531, TRUE, w529) -> (w533:T16)  [unwired: 1 in]
        n1504 = property on="Image Out 2" class="ImageControl"("ROI"=w551) -> ()  [unwired: 2 in, 2 out]
        n1505 = Bundle(w529, w533, w529, w529) -> (w532:T17)  [unwired: 1 in]
        n1506 = property on="Image Out" class="ImageControl"() -> ("ROI"=w516:T10)  [unwired: 2 in, 2 out]
        n1507 = Unbundle By Name(w516) -> ("Contours"=w580:T14)
        n1508 = local read "Image Out"() -> (w535:T2)
        n1509 = call "IMAQ Clear Overlay"("Image"=w535) -> ("Image Out"=w534:T2)  [unwired: 9 in, 1 out]
        n1510 = Initialize Array(0) -> (w578:i32[])  [unwired: 1 in]
        n1511 = local read "Magnification"() -> (w569:u16)
        n1512 = Array Size(array=w580) -> (size(s)=w579:i32)
        n1513 = Build Array(0.505025, 0.252522, 0.127742, 0.050345, 0.031129) -> (w570:dbl[])
        n1514 = Array Subset(array=w570, index=w569, length=1) -> (w567:dbl[])
        n1515 = property on="Image Out" class="ImageControl"() -> ("ZoomInteger"=w559:cluster{"X":i32, "Y":i32})  [unwired: 2 in, 2 out]
        n1516 = To Double Precision Float(number=w567) -> (double precision float=w566:dbl[])
        n1517 = for {
          N: w579 -> [_]
          shift-right: [w856] -> _
          shift-left: w580 -> [w856]
          shift-right: [w854] -> w565
          shift-left: w578 -> [w853]
          tunnel: w566 -> [w852]
          shift-right: [w849] -> _
          shift-left: w534 -> [w851]
          tunnel: w532 -> [w844]
          i -> [w848]
          n1518 = Index Array(array=w856, index=w848) -> (element=w865:T18)
          n1519 = Unbundle(w865) -> ("Points"=w864:i32[])  [unwired: 2 out]
          n1520 = Array To Cluster(array=w864) -> (cluster=w863:T19)
          n1521 = Unbundle(w863) -> ("Points[0]"=w843:i32, "Points[1]"=w840:i32, "Points[2]"=w855:i32, "Points[3]"=w861:i32)  [unwired: 5 out]
          n1522 = Add(x=w843, y=10) -> (x+y=w841:i32)
          n1523 = Subtract(x=w840, y=w861) -> (x-y=w860:i32)
          n1524 = Subtract(x=w843, y=w855) -> (x-y=w862:i32)
          n1525 = Square(x=w860) -> (x^2=w858:i32)
          n1526 = Square(x=w862) -> (x^2=w859:i32)
          n1527 = Add(x=w859, y=w858) -> (x+y=w857:i32)
          n1528 = Square Root(x=w857) -> (sqrt(x)=w834:dbl)
          n1529 = Multiply(x=w834, y=0.5) -> (x*y=w837:dbl)
          n1530 = Add(x=w837, y=w840) -> (x+y=w839:dbl)
          n1531 = Bundle(w841, w839) -> (w850:cluster{i32, dbl})  [unwired: 1 in]
          n1532 = Multiply(x=w834, y=w852) -> (x*y=w847:dbl[])
          n1533 = Index Array(array=w847) -> (element=w846:dbl)  [unwired: 1 in]
          n1534 = Number To Fractional String(number=w846) -> (F-format string=w845:string)  [unwired: 3 in]
          n1535 = call "IMAQ Overlay Text"("BG Color (Transparent)"=u32 0, "Text Color (black)"=u32 16448250, "Font, Size & Style"=w844, "String"=w845, "Origin"=w850, "Image"=w851) -> ("Image Out"=w849:T2)  [unwired: 4 in, 1 out]
          n1536 = Build Array (concatenate)(w853, w847) -> (w854:dbl[])
          n1537 = local write "Numeric 3"(w834) -> ()
        }
        n1538 = local write "ROI Descriptor"(w516) -> ()
        n1539 = Unbundle(w559) -> ("X"=w558:i32)  [unwired: 1 out]
        n1540 = Add Array Elements(numeric array=w565) -> (sum=w576:dbl)
        n1541 = local write "Distances"(w565) -> ()
        n1542 = local write "Total Width"(w576) -> ()
        n1543 = local write "Zoom"(w558) -> ()
        n1544 = local read "Manual-Width"() -> (w515:bool)
        n1545 = local read "Total Width"() -> (w519:dbl)
        n1546 = local read "Rec: Width"() -> (w517:dbl)
        n1547 = Not(x=w515) -> (.not. x?=w513:bool)
        n1548 = Equal To 0?(x=w519) -> (x = 0?=w514:bool)
        n1549 = Or(x=w514, y=w515) -> (x .or. y?=w518:bool)
        n1550 = And(x=w514, y=w513) -> (x .and. y?=w512:bool)
        n1551 = case shown="True" w512 {
          tunnel: w517 -> [_ w594]
          frame False {
          }
          frame True {
            n1552 = local write "New: Width"(w594) -> ()
          }
        }
        n1553 = case shown="False" w518 {
          tunnel: w519 -> [w595 _]
          frame False {
            n1554 = local write "New: Width"(w595) -> ()
          }
          frame True {
          }
        }
        n1555 = local read "Manuel-Dielectric"() -> (w441:bool)
        n1556 = local read "Rec: Dielectric (d)"() -> (w440:dbl)
        n1557 = local read "Manuel-Length"() -> (w442:bool)
        n1558 = local read "Rec: Length"() -> (w443:dbl)
        n1559 = case shown="False" w442 {
          tunnel: w443 -> [w585 _]
          frame False {
            n1560 = local write "New: Length"(w585) -> ()
          }
          frame True {
          }
        }
        n1561 = case shown="False" w441 {
          tunnel: w440 -> [w584 _]
          frame False {
            n1562 = local write "New: Dielectric"(w584) -> ()
          }
          frame True {
          }
        }
      }
    }
  }
  n1563 = Build Array("DeviceID", "Fabricator", "Deposition", "Date", "Sample", "Row", "Column", "L (um)", "W (um)", "Material", "Treatment", "TC (mM)", "Solvent", "C (%)", "ST (C)", "Drops", "Wait (s)", "RT (F)", "RH (%)", "Ramp (s)", "RPM", "Accel (RPM/s)", "Time (s)", "Mobility", "On/Off", "Vt", "S.T.S") -> (→"Transformer \nHeaders":string[])
